vi "RS_SMBV100A.vi"(4 "error in":T15, 7 "Command":T16) -> (0 "error out":T15, 3 "Response":T13)   [LabVIEW 2018]
uses:
  MOKO_LabViewLibrary/MokoLowLevel/MokoLowLovelControl/MLLC_Command.ctl
  MOKO_LabViewLibrary/MokoLowLevel/MokoLowLovelControl/MLLC_Error.ctl
  MOKO_LabViewLibrary/MokoLowLevel/MokoLowLovelControl/MLLC_Mode.ctl
  MOKO_LabViewLibrary/MokoLowLevel/MokoLowLovelControl/MLLC_Response.ctl
  data/RS_SMBV100A_DynamWaypoints.ctl
  data/RS_SMBV100A_DynamWaypoint.ctl
  MOKO_LabViewLibrary/MokoLowLevel/MokoLowLovelControl/MLLC_ConnectCluster.ctl
  MOKO_LabViewLibrary/MokoLowLevel/MokoLowLovelControl/MLLC_InterfaceType.ctl
  MOKO_LabViewLibrary/MokoLowLevel/MokoLowLovelControl/MLLC_OpenedSession.ctl
  MOKO_LabViewLibrary/MokoLowLevel/MokoLowLovelControl/MLLC_InterfaceSettings.ctl
  MOKO_LabViewLibrary/MokoLowLevel/MokoLowLovelControl/MLLC_InterfaceKind.ctl
  MOKO_LabViewLibrary/MokoLowLevel/MokoLowLovelControl/MLLC_DriverName.ctl
  MOKO_LabViewLibrary/MokoLowLevel/MokoLowLovelControl/MLLC_ErrorCode.ctl
  MOKO_LabViewLibrary/MokoLowLevel/MokoLowLovelControl/MLLC_ResponseInit.ctl
  MOKO_LabViewLibrary/MokoLowLevel/MokoLowLovelControl/MLLC_Request.ctl
panel:
  in  "Request":T1="*IDN?"
  in  "ResponseInit":T2="Rohde&Schwarz,SMBV100A"
  in  "Error Code":T3=5450
  in  "Driver Name":T4="RS_SMBV100A"
  in  "Settings":T12={"GPS SCENARIO"="****************************** MOVEMENT FILE ******************************\nRESOLUTION: 50\nREFERENCE: 11.583333,48.150,500\nSTART: 0, 0, 0, 10\nSTAY: 10000\nLINE: 200, 0, 0\nLINE: 100, 0, 19.6\nLINE: 600, 0, 0\nLINE: 100, 0, -19.6\nARC: 1000, 500, 180\nLINE: -200, 0, 0\nLINE: -100, 0, 19.6\nLINE: -600, 0, 0\nLINE: -100, 0, -19.6\nARC: 0, 500, 180", "GLONASS SCENARIO"="****************************** MOVEMENT FILE ******************************\nRESOLUTION: 50\nREFERENCE: 11.583333,48.150,500\nSTART: 0, 0, 0, 10\nSTAY: 10000\nLINE: 200, 0, 0\nLINE: 100, 0, 19.6\nLINE: 600, 0, 0\nLINE: 100, 0, -19.6\nARC: 1000, 500, 180\nLINE: -200, 0, 0\nLINE: -100, 0, 19.6\nLINE: -600, 0, 0\nLINE: -100, 0, -19.6\nARC: 0, 500, 180", "GPS WAYPOINTS"=[], "GLONASS WAYPOINTS"=[], "GALILOE SCENARIO"="****************************** MOVEMENT FILE ******************************\nRESOLUTION: 50\nREFERENCE: 11.583333,48.150,500\nSTART: 0, 0, 0, 10\nSTAY: 10000\nLINE: 200, 0, 0\nLINE: 100, 0, 19.6\nLINE: 600, 0, 0\nLINE: 100, 0, -19.6\nARC: 1000, 500, 180\nLINE: -200, 0, 0\nLINE: -100, 0, 19.6\nLINE: -600, 0, 0\nLINE: -100, 0, -19.6\nARC: 0, 500, 180", "GALILEO WAYPOINTS"=[], "GPS WAYPOINTS STRING"="", "BASEBAND"="GPS", "BEIDOU SCENARIO"="****************************** MOVEMENT FILE ******************************\nRESOLUTION: 50\nREFERENCE: 11.583333,48.150,500\nSTART: 0, 0, 0, 10\nSTAY: 10000\nLINE: 200, 0, 0\nLINE: 100, 0, 19.6\nLINE: 600, 0, 0\nLINE: 100, 0, -19.6\nARC: 1000, 500, 180\nLINE: -200, 0, 0\nLINE: -100, 0, 19.6\nLINE: -600, 0, 0\nLINE: -100, 0, -19.6\nARC: 0, 500, 180", "QZSS SCENARIO"="****************************** MOVEMENT FILE ******************************\nRESOLUTION: 50\nREFERENCE: 11.583333,48.150,500\nSTART: 0, 0, 0, 10\nSTAY: 10000\nLINE: 200, 0, 0\nLINE: 100, 0, 19.6\nLINE: 600, 0, 0\nLINE: 100, 0, -19.6\nARC: 1000, 500, 180\nLINE: -200, 0, 0\nLINE: -100, 0, 19.6\nLINE: -600, 0, 0\nLINE: -100, 0, -19.6\nARC: 0, 500, 180", "BEIDOU WAYPOINTS"=[], "SSDK WAYPOINTS"=[], "Saved Data"=variant, "Data"={"Connect"={"InterfaceType"=enum."VISA", "OpenedSession"="TCPIP0::169.254.1.111::INSTR", "InterfaceSettings"={"Interface"=enum."Ethernet", "EOS 4 read"=enum."LF (\\n)", "EOS 4 write"=enum."LF (\\n)", "TMO, ms"=1000, "Sett"=variant}}}} {"SSDK WAYPOINTS"."Time" format="%<%.3X>T"; "SSDK WAYPOINTS"."Speed" format="%#.10g"; "SSDK WAYPOINTS"."Heigth" format="%#.10g"; "SSDK WAYPOINTS"."Longitude" format="%#.10g"; "SSDK WAYPOINTS"."Latitude" format="%#.10g"; "BEIDOU WAYPOINTS"."Time" format="%<%.3X>T"; "BEIDOU WAYPOINTS"."Speed" format="%#.10g"; "BEIDOU WAYPOINTS"."Heigth" format="%#.10g"; "BEIDOU WAYPOINTS"."Longitude" format="%#.10g"; "BEIDOU WAYPOINTS"."Latitude" format="%#.10g"; "GALILEO WAYPOINTS"."Time" format="%<%.3X>T"; "GALILEO WAYPOINTS"."Speed" format="%#.10g"; "GALILEO WAYPOINTS"."Heigth" format="%#.10g"; "GALILEO WAYPOINTS"."Longitude" format="%#.10g"; "GALILEO WAYPOINTS"."Latitude" format="%#.10g"; "GLONASS WAYPOINTS"."Time" format="%<%.3X>T"; "GLONASS WAYPOINTS"."Speed" format="%#.10g"; "GLONASS WAYPOINTS"."Heigth" format="%#.10g"; "GLONASS WAYPOINTS"."Longitude" format="%#.10g"; "GLONASS WAYPOINTS"."Latitude" format="%#.10g"; "GPS WAYPOINTS"."Time" format="%<%.3X>T"; "GPS WAYPOINTS"."Speed" format="%#.10g"; "GPS WAYPOINTS"."Heigth" format="%#.10g"; "GPS WAYPOINTS"."Longitude" format="%#.10g"; "GPS WAYPOINTS"."Latitude" format="%#.10g"}
  in  "Mode":T14=enum."Check"
  # "RS_SMBV100A"
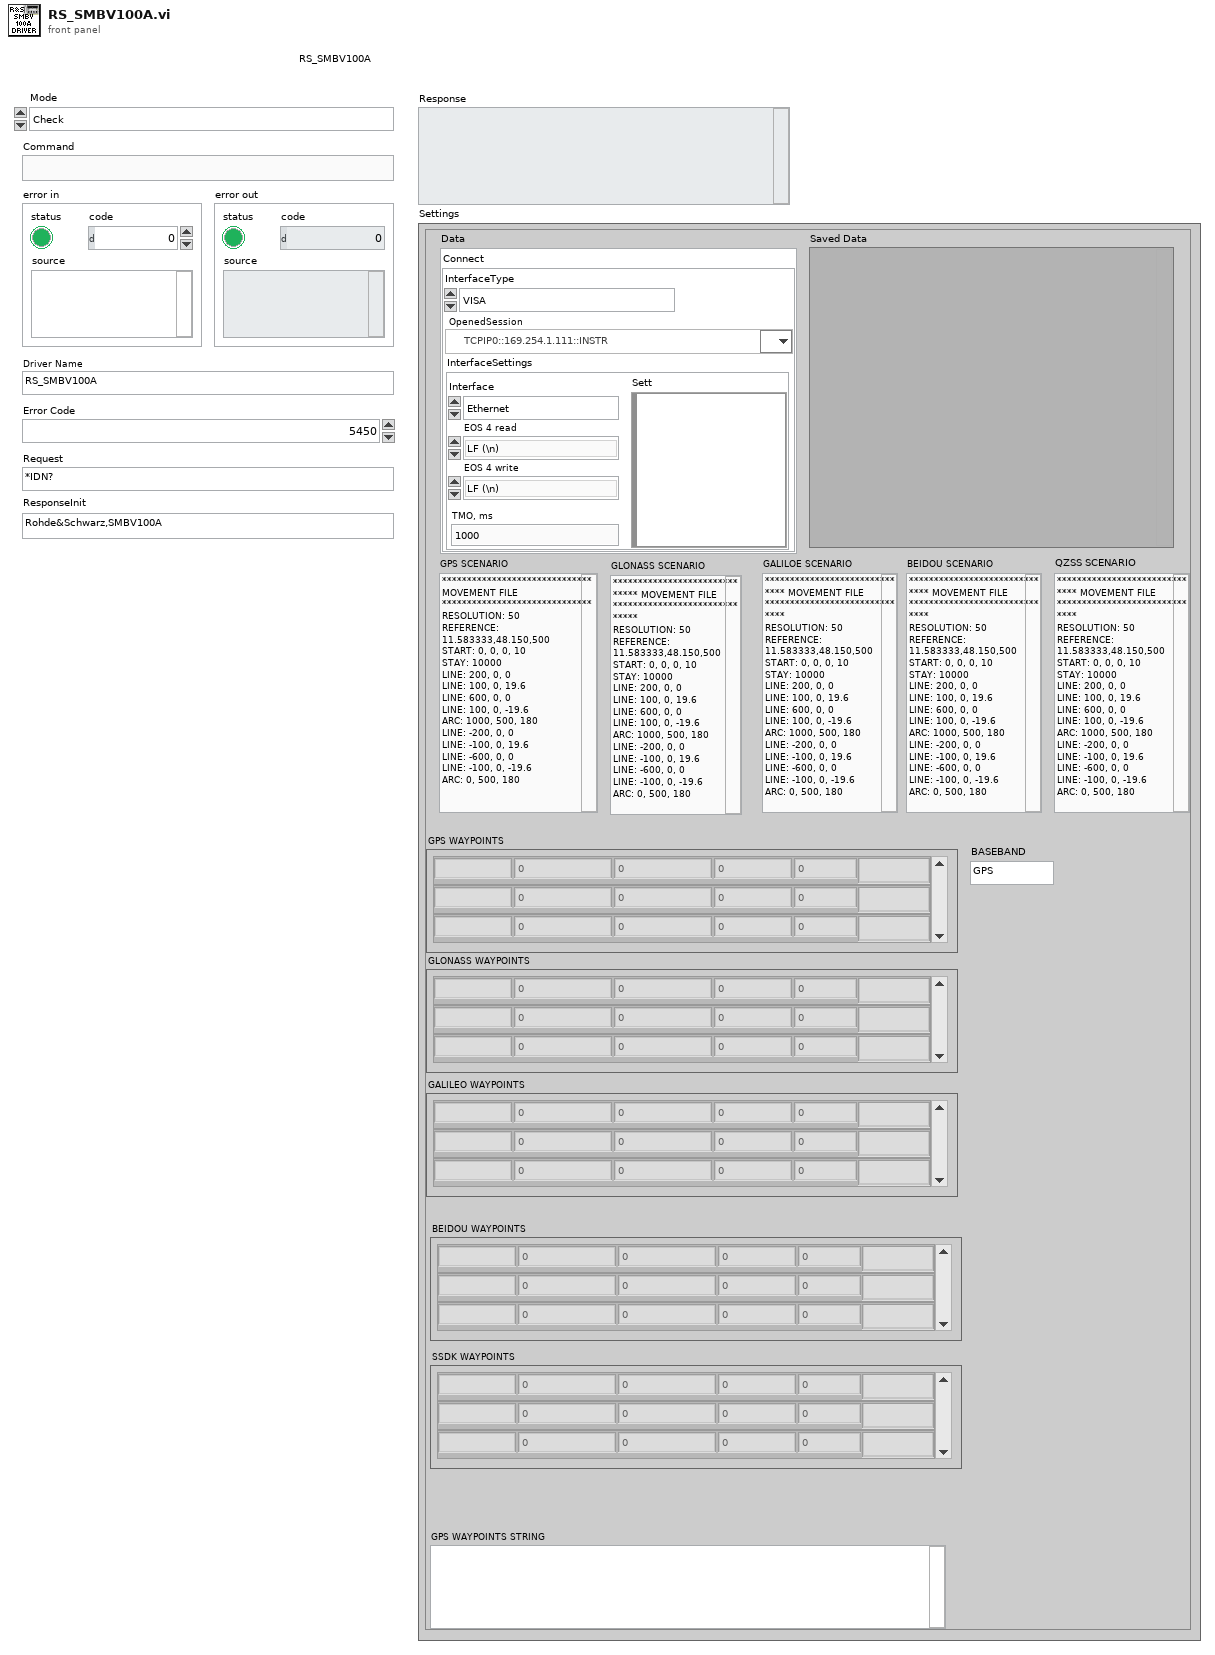
[diagram p1: front panel]
types:
  T1 = typedef "MLLC_Request.ctl" = string
  T2 = typedef "MLLC_ResponseInit.ctl" = string
  T3 = typedef "MLLC_ErrorCode.ctl" = u32
  T4 = typedef "MLLC_DriverName.ctl" = string
  T5 = typedef "RS_SMBV100A_DynamWaypoints.ctl" = T6[]
  T6 = typedef "RS_SMBV100A_DynamWaypoint.ctl" = cluster{"Time":timestamp, "Latitude":ext, "Longitude":ext, "Heigth":dbl, "Speed":dbl, "Scenario":string}
  T7 = typedef "MLLC_ConnectCluster.ctl" = cluster{"InterfaceType":T8, "OpenedSession":T9, "InterfaceSettings":T10}
  T8 = typedef "MLLC_InterfaceType.ctl" = enum16{"VISA", "Prologix USB-GPIB"}
  T9 = typedef "MLLC_OpenedSession.ctl" = refnum<visa-resource-name>
  T10 = typedef "MLLC_InterfaceSettings.ctl" = cluster{"Interface":T11, "EOS 4 read":enum16{"Default (=EOS 4 write)", "CR (\\r)", "LF (\\n)", "None"}, "EOS 4 write":enum16{"CR+LF (\\r\\n)", "CR (\\r)", "LF (\\n)", "None"}, "TMO, ms":i32, "Sett":variant}
  T11 = typedef "MLLC_InterfaceKind.ctl" = enum16{"RS232", "GPIB", "USB", "Ethernet", "another"}
  T12 = cluster{"GPS SCENARIO":string, "GLONASS SCENARIO":string, "GPS WAYPOINTS":T5, "GLONASS WAYPOINTS":T5, "GALILOE SCENARIO":string, "GALILEO WAYPOINTS":T5, "GPS WAYPOINTS STRING":string, "BASEBAND":string, "BEIDOU SCENARIO":string, "QZSS SCENARIO":string, "BEIDOU WAYPOINTS":T5, "SSDK WAYPOINTS":T5, "Saved Data":variant, "Data":cluster{"Connect":T7}}
  T13 = typedef "MLLC_Response.ctl" = string
  T14 = typedef "MLLC_Mode.ctl" = enum16{"get", "set", "close", "Init", "Check"}
  T15 = typedef "MLLC_Error.ctl" = errorcluster
  T16 = typedef "MLLC_Command.ctl" = string
  T17 = enum16{"open", "replace", "create", "open or create", "replace or create", "replace or create with confirmation"}
  T18 = typedef "RS_SMBV100A_Parsing Satelite.ctl" = cluster{"Time":dbl[], "Sat":dbl[], "State":dbl[], "NUMBERINSKY":dbl[], "STANDART":string[]}
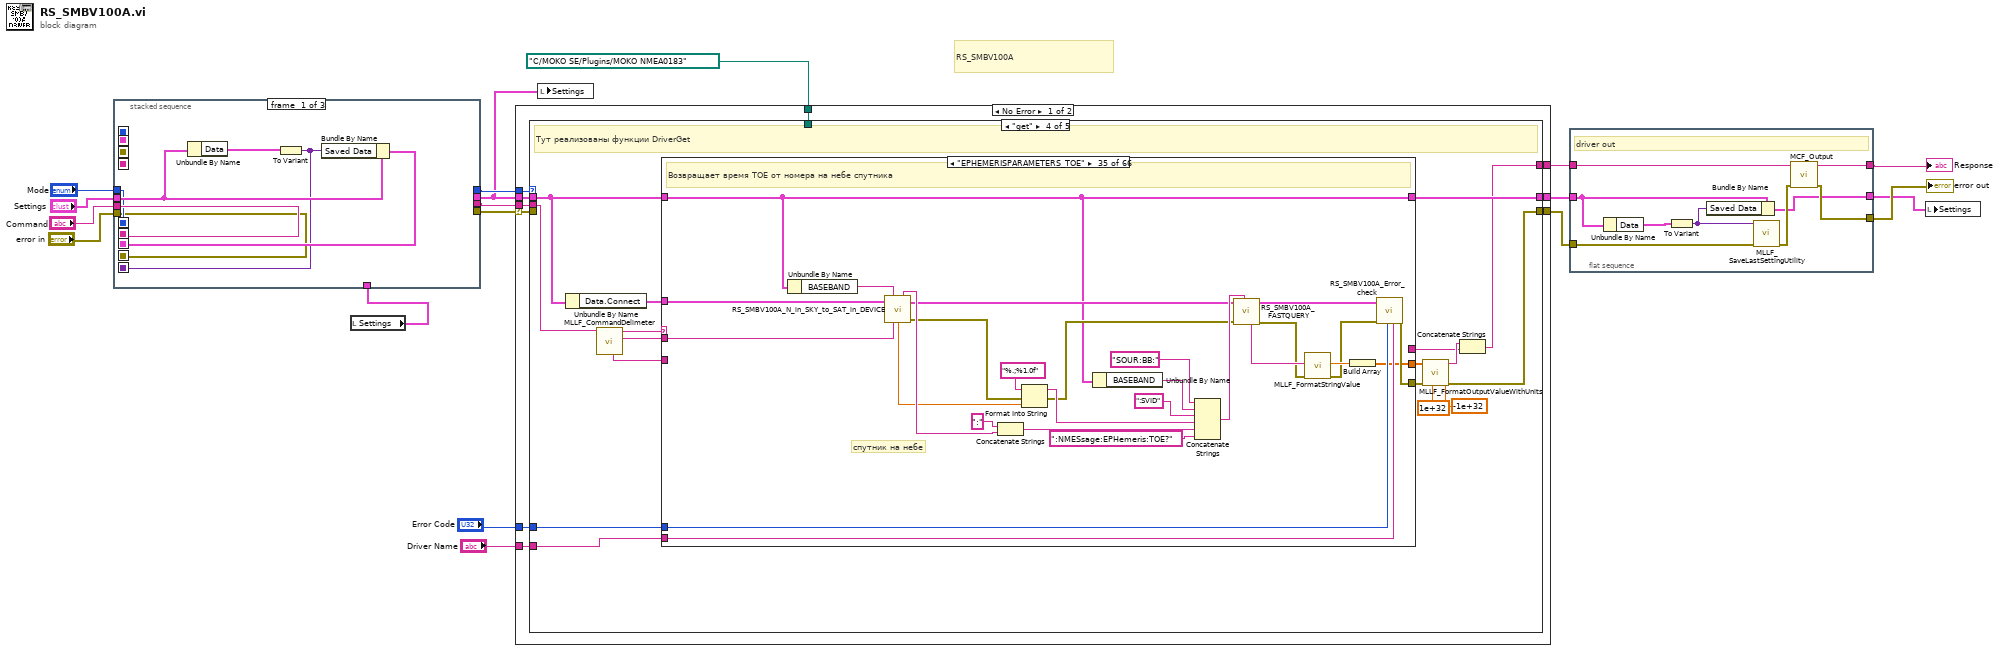
[diagram p0: block diagram]
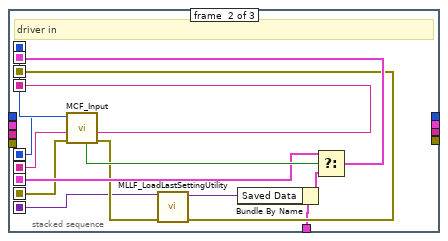
[diagram p2: hidden frame]
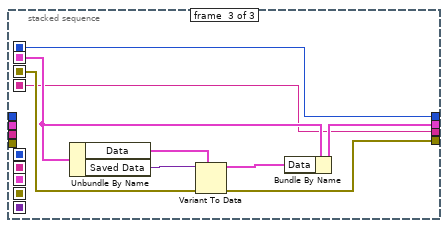
[diagram p3: hidden frame]
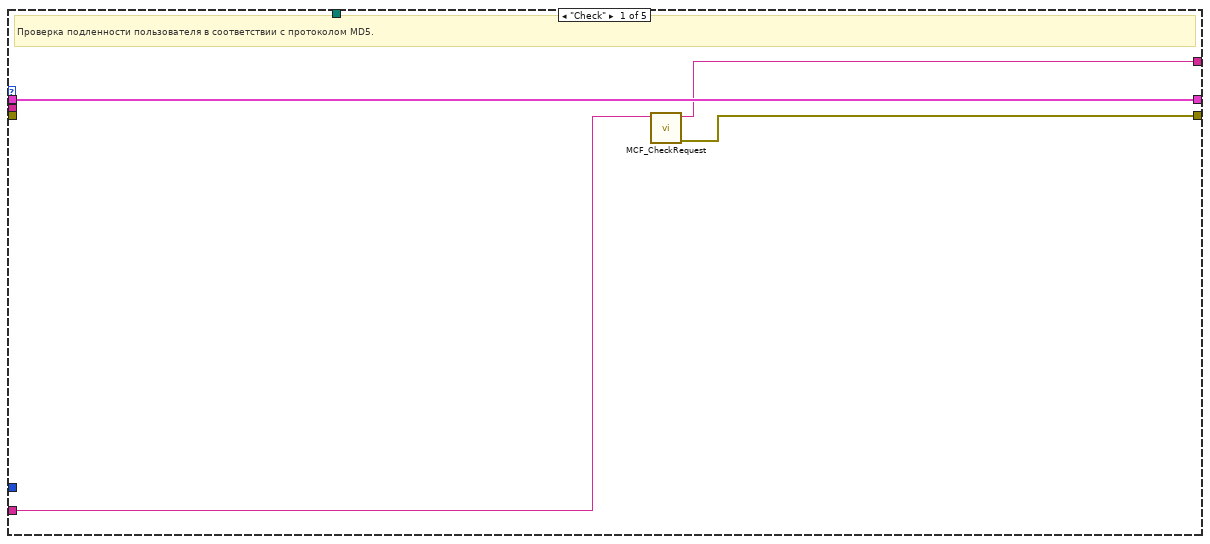
[diagram p4: hidden frame]
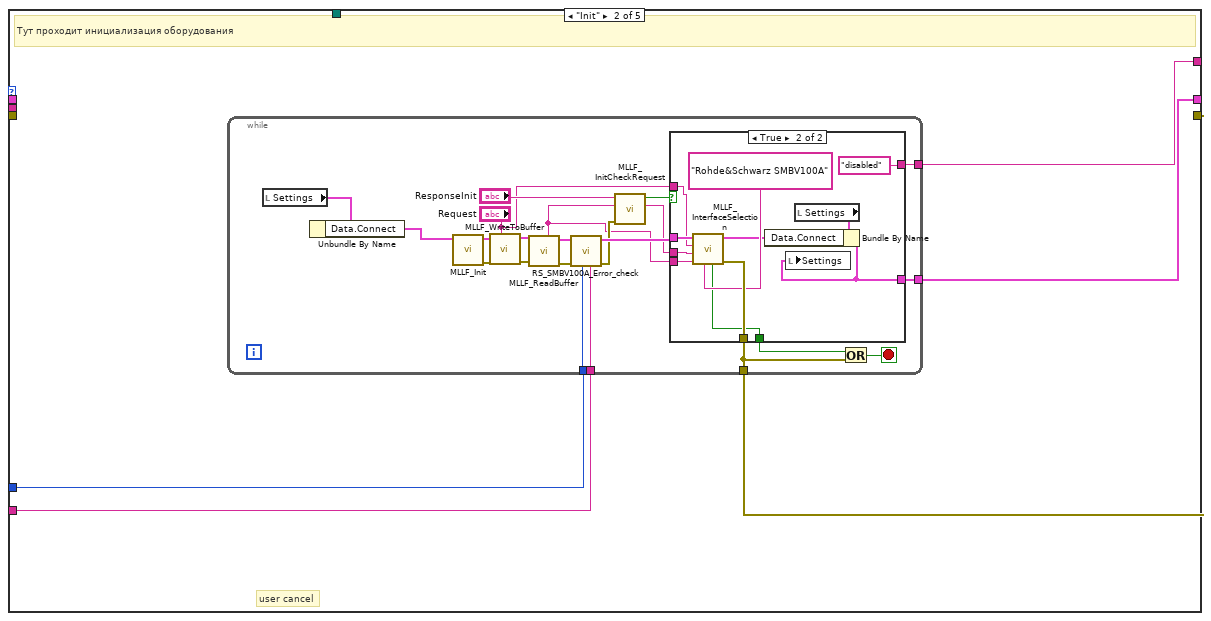
[diagram p5: hidden frame]
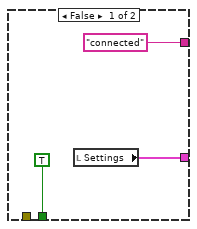
[diagram p6: hidden frame]
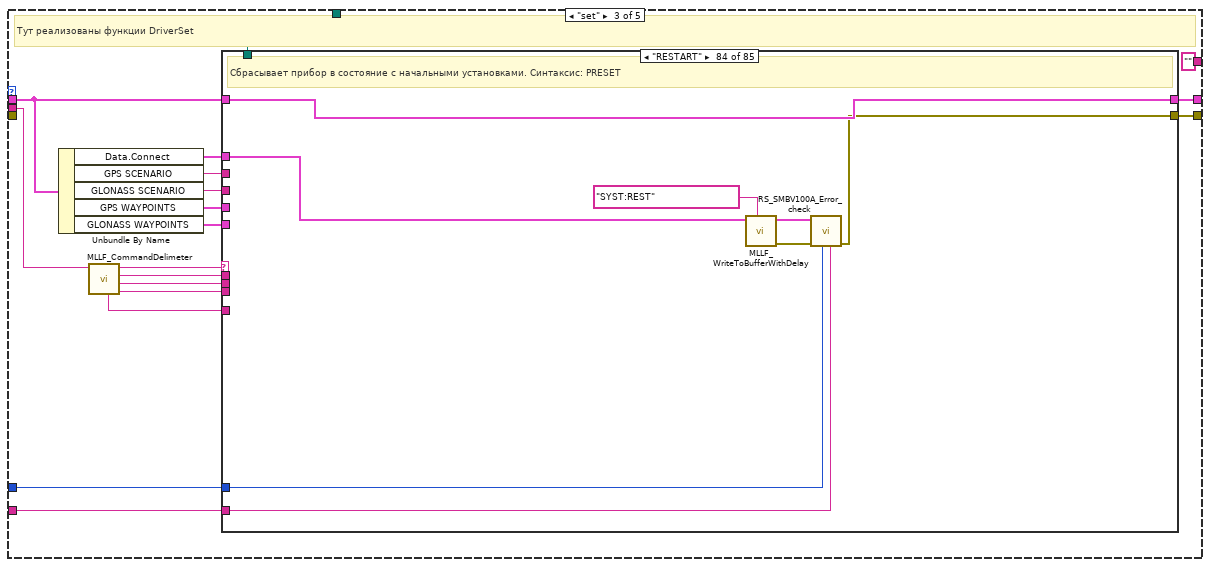
[diagram p7: hidden frame]
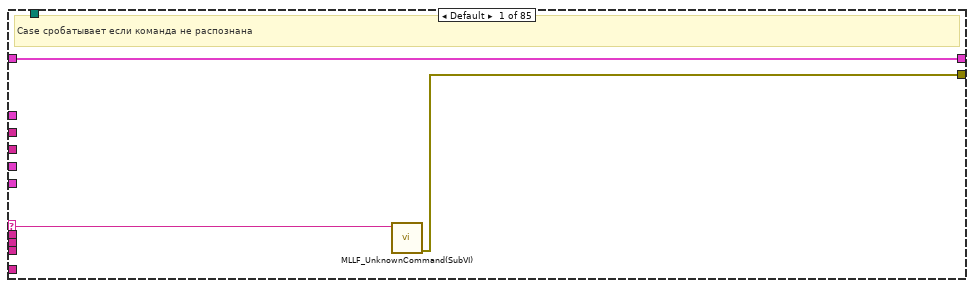
[diagram p8: hidden frame]
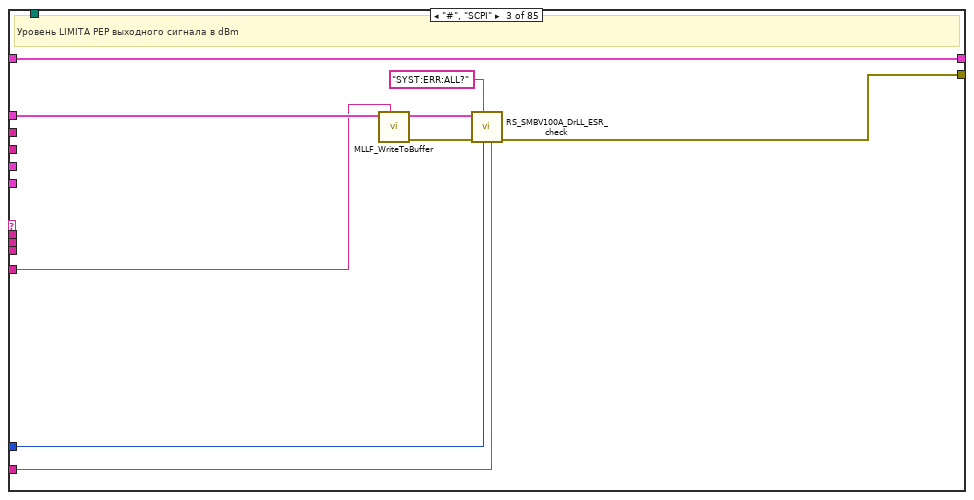
[diagram p10: hidden frame]
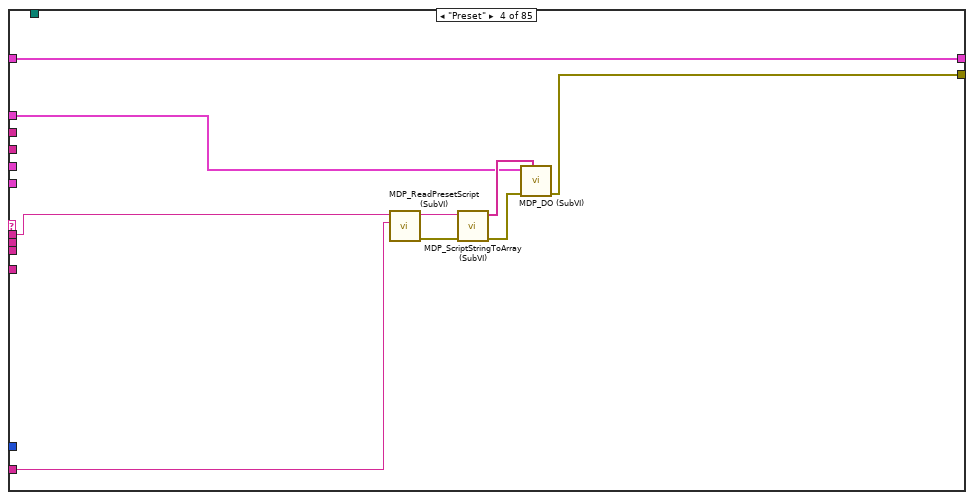
[diagram p11: hidden frame]
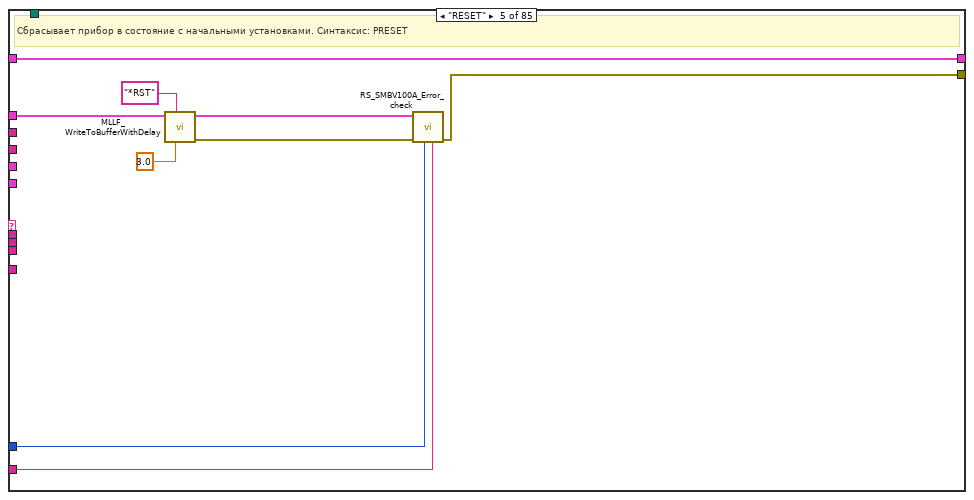
[diagram p12: hidden frame]
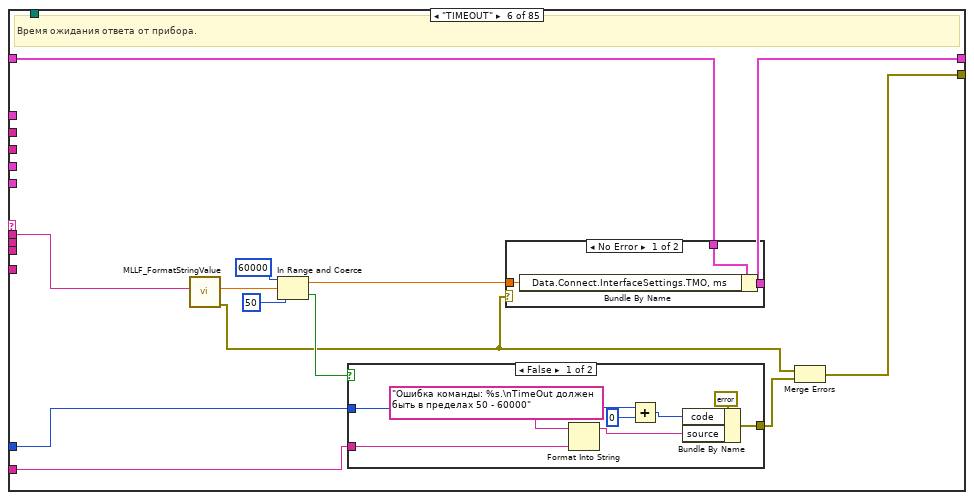
[diagram p13: hidden frame]
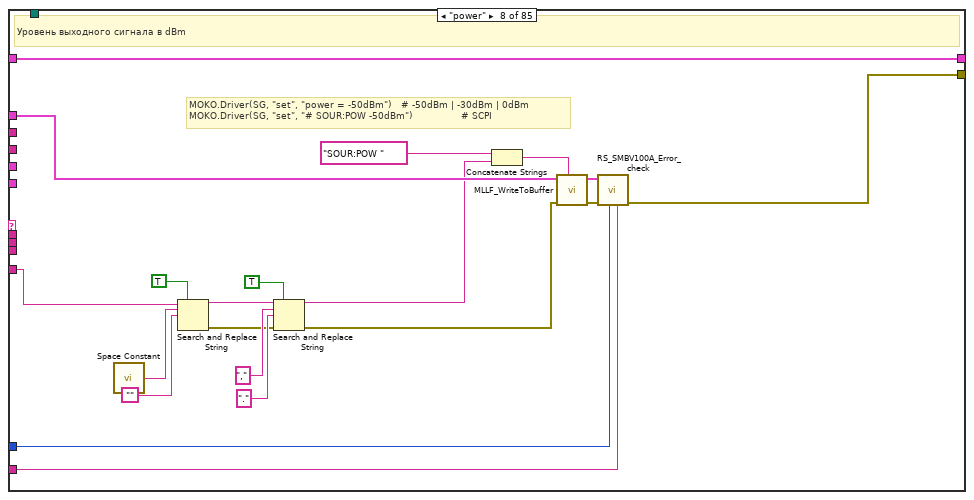
[diagram p17: hidden frame]
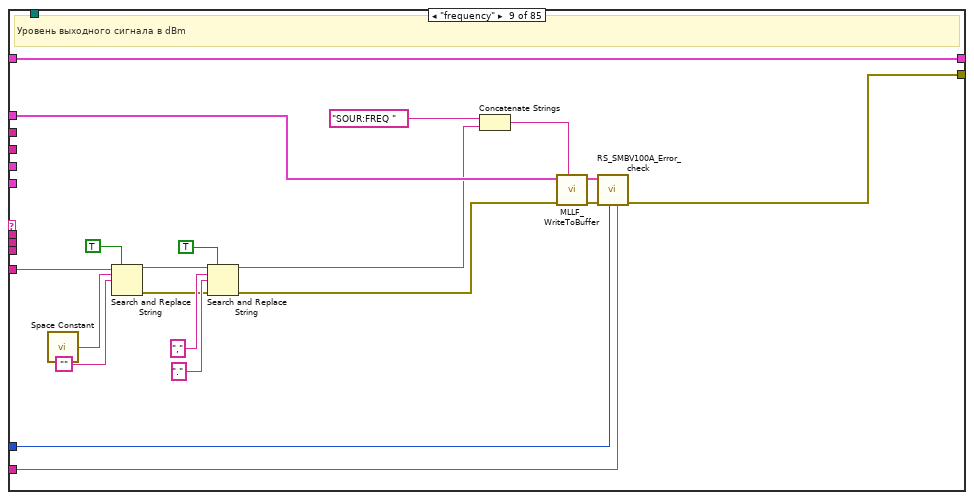
[diagram p18: hidden frame]
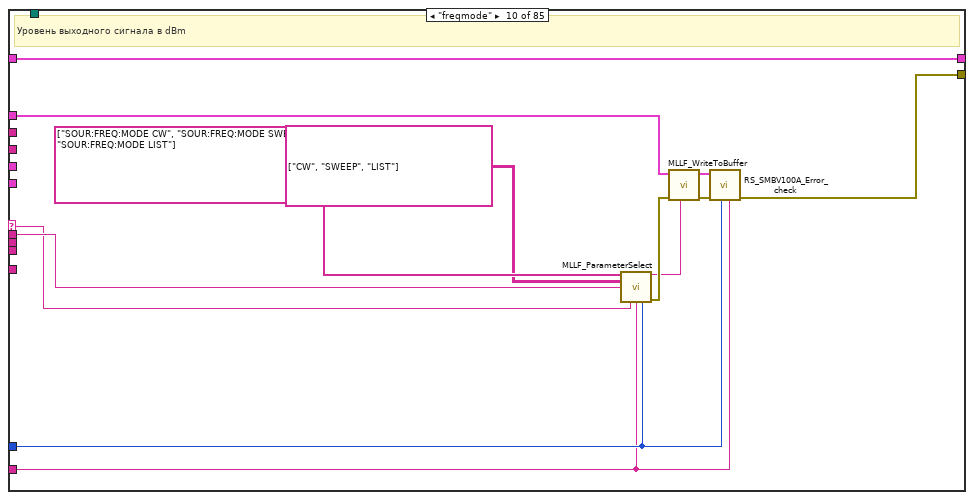
[diagram p19: hidden frame]
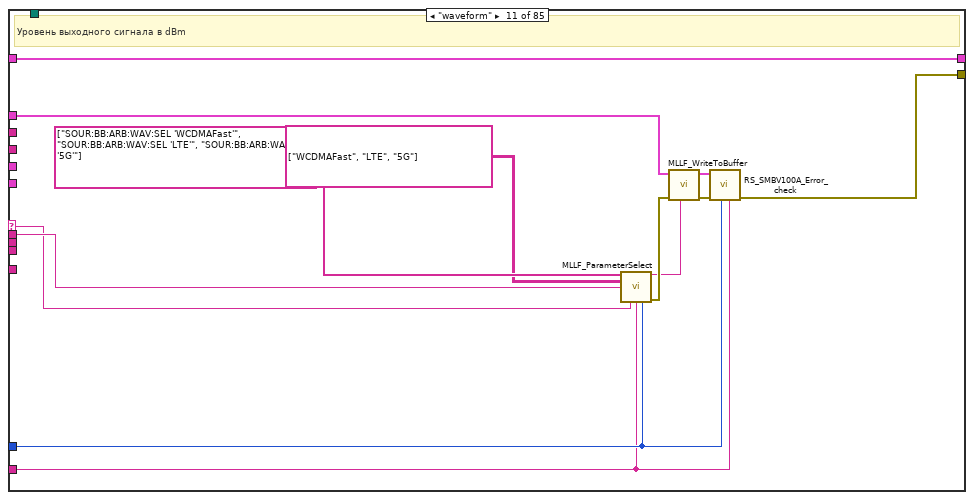
[diagram p20: hidden frame]
diagram:
  # "RS_SMBV100A"
  n1 = local read "Settings"() -> (w7:T12)
  n2 = stacked-sequence {
    seq-local: [w21 _ _] -> [_ w37 _]
    seq-local: [w20 _ _] -> [_ w38 _]
    seq-local: [w23 _ _] -> [_ w33 _]
    seq-local: [w19 _ _] -> [_ w32 _]
    seq-local: [w22 _ _] -> [_ w28 _]
    seq-local: [_ w29 _] -> [_ _ w45]
    seq-local: [_ w39 _] -> [_ _ w42]
    seq-local: [_ w36 _] -> [_ _ w41]
    seq-local: [_ w35 _] -> [_ _ w46]
    tunnel: "Command" -> [w21 _ _]
    tunnel: "Mode" -> [w20 _ _]
    tunnel: "error in" -> [w19 _ _]
    tunnel: "Settings" -> [w24 _ _]
    tunnel: w7 -> [_ w27 _]
    tunnel: [_ _ w41] -> w9
    tunnel: [_ _ w44] -> w10
    tunnel: [_ _ w43] -> w8
    tunnel: [_ _ w42] -> w11
    frame #0 {
      n3 = Unbundle By Name(w24) -> ("Data"=w25:cluster{"Connect":T7})
      n4 = To Variant(anything=w25) -> (Variant=w22:variant)
      n5 = Bundle By Name(cluster=w24, "Saved Data"=w22) -> (w23:T12)
    }
    frame #1 {
      # "driver in"
      n6 = call "MCF_Input.vi"("Error In"=w32, "Command in"=w37, "Mode in"=w38) -> ("Error Out"=w31:errorcluster, "Command out"=w36:string, "Mode out"=w39:T14, "Boolean"=w34:bool)  [unwired: 5 in]
      n7 = call "MLLF_LoadLastSettingUtility.vi"("Error In"=w31, "Save data in"=w28) -> ("Error Out"=w29:errorcluster, "Save data out"=w26:variant)  [unwired: 8 in]
      n8 = Bundle By Name(cluster=w27, "Saved Data"=w26) -> (w30:T12)
      n9 = Select(t=w33, s=w34, f=w30) -> (s? t:f=w35:T12)
    }
    frame #2 {
      n10 = Unbundle By Name(w46) -> ("Data"=w47:cluster{"Connect":T7}, "Saved Data"=w40:variant)
      n11 = Variant To Data(error in=w45, type=w47, Variant=w40) -> (data=w48:cluster{"Connect":T7}, error out=w43:errorcluster)
      n12 = Bundle By Name(cluster=w46, "Data"=w48) -> (w44:T12)
    }
  }
  n13 = case shown="No Error" w8 {
    selector: w8 -> [w55 w2154]
    tunnel: [w57 w2154] -> w4
    tunnel: w11 -> [w49 _]
    tunnel: [w58 _] -> w6
    tunnel: w9 -> [w56 _]
    tunnel: w10 -> [w52 w2153]
    tunnel: "Error Code" -> [w54 _]
    tunnel: "Driver Name" -> [w53 _]
    tunnel: [w51 w2153] -> w5
    tunnel: path "C:/MOKO SE/Plugins/MOKO NMEA0183" ("base path") -> [w50 _]
    frame No Error {
      n14 = case shown="\"get\"" w49 {
        tunnel: [w60 w63 "" ("Output String") w1264 "" ("Output String")] -> w58
        tunnel: [w59 w64 w121 w1263 w2151] -> w57
        tunnel: w56 -> [_ _ w104 w1276 _]
        tunnel: w55 -> [_ _ _ _ _]
        tunnel: w54 -> [_ w67 w120 w1273 _]
        tunnel: w53 -> [w61 w66 w117 w1272 _]
        tunnel: w52 -> [w62 _ w119 w1275 w2150]
        tunnel: [w62 w65 w118 w1274 w2150] -> w51
        tunnel: w50 -> [_ _ w116 _ _]
        frame "Check" {
          # "Проверка подленности пользователя в соответствии с протоколом MD5."
          n15 = call "MCF_CheckRequest.vi"("Driver Name"=w61) -> ("Error Out"=w59:errorcluster, "Output String"=w60:string)  [unwired: 9 in]
        }
        frame "Init" {
          # "user cancel"
          # "Тут проходит инициализация оборудования"
          n16 = while {
            tunnel: [w82] -> w64
            tunnel: w67 -> [w79]
            tunnel: w66 -> [w78]
            tunnel: [w75] -> w65
            tunnel: [w74] -> w63
            stop <- w81 stop-if-true
            n17 = local read "Settings"() -> (w84:T12)
            n18 = Unbundle By Name(w84) -> ("Data.Connect"=w85:T7)
            n19 = call "MLLF_Init.vi"("DriverConnect in"=w85) -> ("Error Out"=w87:errorcluster, "DriverConnect out"=w86:T7)  [unwired: 7 in]
            n20 = call "MLLF_WriteToBuffer.vi"("String"="Request", "error in"=w87, "DriverConnect in"=w86) -> ("error out"=w89:T15, "DriverConnect out"=w88:T7)  [unwired: 5 in]
            n21 = call "MLLF_ReadBuffer.vi"("Error In"=w89, "DriverConnect in"=w88) -> ("Error Out"=w76:errorcluster, "DriverConnect out"=w77:T7, "String"=w70:string)  [unwired: 6 in]
            n22 = call "RS_SMBV100A_Error_check.vi"("Driver Name"=w78, "Error Code"=w79, "Error In"=w76, "DriverConnect in"=w77) -> ("Error Out"=w72:errorcluster, "DriverConnect out"=w80:T7)  [unwired: 6 in]
            n23 = call "MLLF_InitCheckRequest.vi"("error in (no error)"=w72, "Answer"=w70, "Response Init"="ResponseInit") -> ("ResponseInit out"=w69:string, "Design"=w71:bool)  [unwired: 5 in, 2 out]
            n24 = case shown="True" w71 {
              tunnel: w80 -> [_ w102]
              tunnel: [TRUE w96] -> w83
              tunnel: [_ w103] -> w82
              tunnel: [w91 w98] -> w75
              tunnel: ["connected" "disabled"] -> w74
              tunnel: w70 -> [_ w95]
              tunnel: w69 -> [_ w94]
              tunnel: "Request" -> [_ w93]
              frame False {
                n25 = local read "Settings"() -> (w91:T12)
              }
              frame True {
                n26 = call "MLLF_InterfaceSelection.vi"("Driver Name"="Rohde&Schwarz SMBV100A" ("String"), "Answer:"=w95, "Response"=w94, "Request"=w93, "DriverConnect in"=w102) -> ("error out"=w103:T15, "DriverConnect out"=w100:T7, "stop init?"=w96:bool)  [unwired: 2 in, 2 out]
                n27 = local read "Settings"() -> (w99:T12)
                n28 = Bundle By Name(cluster=w99, "Data.Connect"=w100) -> (w98:T12)
                n29 = local write "Settings"(w98) -> ()
              }
            }
            n30 = Or(x=w83, y=w82) -> (x .or. y?=w81:bool)
          }
        }
        frame "set" {
          # "Тут реализованы функции DriverSet"
          n31 = Unbundle By Name(w119) -> ("Data.Connect"=w114:T7, "GPS SCENARIO"=w113:string, "GLONASS SCENARIO"=w112:string, "GPS WAYPOINTS"=w111:T5, "GLONASS WAYPOINTS"=w110:T5)
          n32 = call "MLLF_CommandDelimeter.vi"("command with param"=w104) -> ("param 3"=w106:string, "param 2"=w107:string, "param 1"=w108:string, "command"=w109:string, "Spit delimetre"=w105:string)  [unwired: 6 in]
          n33 = case shown="\"RESTART\"" w109 {
            selector: w109 -> [w123 _ _ _ _ _ _ _ _ w224 w237 _ w258 w266 _ _ _ _ _ _ _ _ _ _ _ _ w396 _ _ _ _ _ _ _ w530 w547 w562 _ _ _ w622 _ w661 w678 w697 _ _ w750 _ _ _ w793 _ w830 _ w862 w878 _ _ w913 _ _ w982 _ w1000 w1017 w1034 w1051 _ _ w1087 _ _ _ _ w1150 _ _ _ _ _ _ _ _ _]
            tunnel: [w122 _ w126 w135 w144 w156 _ w192 w212 w221 w234 w246 w255 w268 _ _ _ _ w304 w322 _ w351 _ w358 w374 w393 w404 _ w427 w446 w465 w484 w503 w522 w544 w561 w578 w594 w612 _ w630 w655 w669 w686 w711 w726 w739 w758 _ w778 w787 w801 w825 w840 w856 w871 w887 w901 _ w927 w948 w979 w990 _ w1008 w1025 w1043 w1059 w1075 _ w1095 w1110 w1122 _ w1144 w1166 _ w1181 w1200 _ w1215 w1222 w1230 w1238 w1253] -> w121
            tunnel: w120 -> [_ _ w130 _ w146 w157 _ w197 w217 w223 w236 w248 w257 w273 _ _ _ _ w303 _ _ w355 _ _ _ _ w409 _ w432 w451 w470 w489 w508 w527 w528 w545 w563 w593 _ _ w635 w660 w674 w691 w695 w731 w744 w748 _ w774 w792 w806 w829 w845 w861 w876 w892 w906 _ w911 w950 w981 w995 _ w1013 w1030 w1047 w1064 w1080 _ w1085 w1109 w1124 _ w1149 w1153 _ w1180 _ _ w1220 w1224 w1232 w1240 w1258]
            tunnel: w119 -> [w124 w125 w134 w143 w152 w155 w178 w198 w218 w231 w244 w252 w265 w278 w279 w280 w284 w288 w313 w326 w331 w338 w356 w359 w363 w387 w403 w413 w416 w436 w455 w472 w491 w510 w534 w551 w568 w603 w616 w621 w629 w644 w663 w680 w699 w714 w735 w752 w765 w769 w782 w795 w814 w832 w848 w865 w879 w897 w910 w915 w930 w953 w984 w999 w1002 w1019 w1037 w1053 w1069 w1084 w1089 w1105 w1117 w1128 w1129 w1154 w1167 w1190 w1203 w1207 w1221 w1229 w1237 w1245 w1259]
            tunnel: [w124 w125 w134 w143 w152 w154 w178 w198 w218 w231 w244 w252 w265 w278 w279 w280 w283 w288 w312 w325 w331 w338 w356 w359 w363 w387 w403 w413 w416 w436 w455 w472 w491 w510 w534 w551 w568 w602 w615 w621 w629 w644 w663 w680 w699 w714 w735 w752 w765 w769 w782 w795 w814 w832 w848 w865 w879 w897 w910 w915 w930 w953 w984 w999 w1002 w1019 w1037 w1053 w1069 w1084 w1089 w1105 w1117 w1128 w1129 w1154 w1167 w1189 w1202 w1207 w1221 w1229 w1237 w1245 w1259] -> w118
            tunnel: w114 -> [_ _ w133 w138 w147 _ _ w195 w215 w226 w239 w249 w260 w271 _ _ _ _ w306 _ _ w350 _ _ w383 w395 w407 _ w430 w449 w468 w487 w506 w525 w538 w555 w572 w596 _ _ w633 w658 w672 w689 w705 w729 w742 w759 _ w781 w790 w804 w824 w843 w859 w874 w890 w904 _ w923 w947 w978 w993 _ w1011 w1028 w1046 w1062 w1078 _ w1096 w1111 w1125 _ w1147 w1162 _ w1183 _ _ w1218 w1225 w1233 w1241 w1256]
            tunnel: w117 -> [_ _ w129 w136 w145 w158 _ w196 w216 w222 w235 w247 w256 w272 _ _ _ _ w302 _ _ w354 _ _ _ _ w408 _ w431 w450 w469 w488 w507 w526 w529 w546 w564 w592 _ _ w634 w659 w673 w690 w696 w730 w743 w749 _ w775 w791 w805 w828 w844 w860 w875 w891 w905 _ w912 w949 w980 w994 _ w1012 w1029 w1035 w1063 w1079 _ w1086 w1108 w1123 _ w1148 w1152 _ w1179 _ _ w1219 w1223 w1231 w1239 w1257]
            tunnel: w108 -> [_ _ _ w137 _ w153 _ _ _ w225 w238 _ w259 w267 _ _ w281 _ w291 w316 _ w333 _ _ w361 w392 w397 _ w418 w438 w457 w475 w494 w513 w531 w548 w565 w581 w606 _ w623 w641 w662 w679 w698 w716 w732 w751 _ w766 _ w794 w811 w831 w847 _ _ w894 _ w914 w934 w958 w983 _ w1001 w1018 w1036 w1052 w1068 _ w1088 w1102 _ _ w1135 w1151 _ w1169 w1195 _ w1211 _ _ _ w1249]
            tunnel: w113 -> [_ _ _ _ _ _ _ _ _ _ _ _ _ _ _ _ _ _ _ _ _ _ _ _ w369 _ _ _ _ _ _ _ _ _ _ _ _ _ _ _ _ _ _ _ _ _ _ _ _ _ _ _ _ _ _ _ _ _ _ _ _ _ _ _ _ _ _ _ _ _ _ _ _ _ _ _ _ _ _ _ _ _ _ _ _]
            tunnel: w112 -> [_ _ _ _ _ _ _ _ _ _ _ _ _ _ _ _ _ _ _ _ _ _ _ _ _ w389 _ _ _ _ _ _ _ _ _ _ _ _ _ _ _ _ _ _ _ _ _ _ _ _ _ _ _ _ _ _ _ _ _ _ _ _ _ _ _ _ _ _ _ _ _ _ _ _ _ _ _ _ _ _ _ _ _ _ _]
            tunnel: w111 -> [_ _ _ _ _ _ _ _ _ _ _ _ _ _ _ _ _ _ _ _ _ _ _ _ _ _ _ _ _ _ _ _ _ _ _ _ _ _ _ _ _ _ _ _ _ _ _ _ _ _ _ _ _ _ _ _ _ _ _ _ _ _ _ _ _ _ _ _ _ _ _ _ _ _ _ _ _ _ _ _ _ _ _ _ _]
            tunnel: w110 -> [_ _ _ _ _ _ _ _ _ _ _ _ _ _ _ _ _ _ _ _ _ _ _ w357 _ _ _ _ _ _ _ _ _ _ _ _ _ _ _ _ _ _ _ _ _ _ _ _ _ _ _ _ _ _ _ _ _ _ _ _ _ _ _ _ _ _ _ _ _ _ _ _ _ _ _ _ _ _ _ _ _ _ _ _ _]
            tunnel: w116 -> [_ _ _ _ _ _ _ _ _ _ _ _ _ _ _ _ _ _ w289 w315 _ _ _ _ w364 _ _ _ _ _ _ _ _ _ _ _ _ w579 w605 _ _ _ _ _ _ _ _ _ _ _ _ _ _ _ _ _ _ _ _ _ _ _ _ _ _ _ _ _ _ _ _ _ _ _ _ _ _ w1168 w1192 _ _ _ _ _ _]
            tunnel: w107 -> [_ _ _ _ _ _ _ _ _ _ _ _ _ _ _ _ _ _ _ _ _ w332 _ _ w360 _ _ _ _ _ _ _ _ _ _ _ _ _ _ _ _ w640 _ _ _ _ _ _ _ _ _ _ w810 _ _ _ _ _ _ _ _ _ _ _ _ _ _ _ _ _ _ _ _ _ _ _ _ _ _ _ _ _ _ _ _]
            tunnel: w106 -> [_ _ _ _ _ _ _ _ _ _ _ _ _ _ _ _ _ _ _ _ _ _ _ _ _ _ _ _ _ _ _ _ _ _ _ _ _ _ _ _ _ w639 _ _ _ _ _ _ _ _ _ _ _ _ _ _ _ _ _ _ _ _ _ _ _ _ _ _ _ _ _ _ _ _ _ _ _ _ _ _ _ _ _ _ _]
            tunnel: w105 -> [_ _ w132 _ _ _ _ w184 w209 _ _ _ _ _ _ _ _ _ _ _ _ _ _ _ _ _ _ _ _ _ _ _ _ _ _ _ _ _ _ _ _ _ _ _ _ _ _ _ _ _ _ _ _ _ _ _ _ _ _ _ _ _ _ _ _ _ _ _ _ _ _ _ _ _ _ _ _ _ _ _ _ _ _ _ _]
            frame Default {
              # "Case сробатывает если команда не распознана"
              n34 = call "MLLF_UnknownCommand(SubVI).vi"("Unknown command"=w123) -> ("error out"=w122:errorcluster)  [unwired: 10 in]
            }
            frame "______________ Standart ________________" {
            }
            frame "#", "SCPI" {
              # "Уровень LIMITA PEP выходного сигнала в dBm"
              n35 = call "MLLF_WriteToBuffer.vi"("String"=w132, "DriverConnect in"=w133) -> ("error out"=w127:T15, "DriverConnect out"=w128:T7)  [unwired: 6 in]
              n36 = call "RS_SMBV100A_DrLL_ESR_check.vi"("Driver Name"=w129, "Error Code"=w130, "Error Query"="SYST:ERR:ALL?", "Error In"=w127, "DriverConnect in"=w128) -> ("Error Out"=w126:errorcluster)  [unwired: 5 in, 1 out]
            }
            frame "Preset" {
              n37 = call "MDP_ReadPresetScript (SubVI).vi"("Driver Name"=w136, "String in"=w137) -> ("Error Out"=w140:errorcluster, "String out"=w141:string)  [unwired: 8 in]
              n38 = call "MDP_ScriptStringToArray (SubVI).vi"("Error In"=w140, "String script"=w141) -> ("Error Out"=w142:errorcluster, "Array script"=w139:string[])  [unwired: 8 in]
              n39 = call "MDP_DO (SubVI).vi"("Array script"=w139, "Error in (no error)"=w142, "DriverConnect in"=w138) -> ("Error Out"=w135:errorcluster)  [unwired: 7 in, 1 out]
            }
            frame "RESET" {
              # "Сбрасывает прибор в состояние с начальными установками. Синтаксис: PRESET"
              n40 = call "MLLF_WriteToBufferWithDelay.vi"("Delay Time ( 0,05 s)"=3.0, "Command"="*RST" ("String"), "DriverConnect in"=w147) -> ("Error Out"=w150:errorcluster, "DriverConnect out"=w151:T7)  [unwired: 7 in]
              n41 = call "RS_SMBV100A_Error_check.vi"("Driver Name"=w145, "Error Code"=w146, "Error In"=w150, "DriverConnect in"=w151) -> ("Error Out"=w144:errorcluster)  [unwired: 6 in, 1 out]
            }
            frame "TIMEOUT" {
              # "Время ожидания ответа от прибора."
              n42 = call "MLLF_FormatStringValue.vi"("String Value"=w153) -> ("error out"=w160:T15, "number"=w159:dbl)  [unwired: 8 in, 1 out]
              n43 = In Range and Coerce(upper limit=60000, x=w159, lower limit=50) -> (coerced(x)=w163:dbl, In Range?=w161:bool)
              n44 = case shown="False" w161 {
                tunnel: [w172 _] -> w162
                tunnel: w157 -> [w171 _]
                tunnel: w158 -> [w170 _]
                frame False {
                  n45 = Format Into String(format string="Ошибка команды: %s.\nTimeOut должен быть в пределах 50 - 60000", w170) -> (resulting string=w174:string)  [unwired: 2 in, 1 out]
                  n46 = Add(x=w171, y=0) -> (x+y=w175:T3)
                  n47 = Bundle By Name(cluster=errorcluster {"status"=TRUE, "code"=0, "source"=""} ("error out"), "code"=w175, "source"=w174) -> (w172:errorcluster)
                }
                frame True {
                }
              }
              n48 = case shown="No Error" w160 {
                tunnel: [w168 w169] -> w154
                tunnel: w155 -> [w167 w169]
                tunnel: w163 -> [w166 _]
                frame No Error {
                  n49 = Bundle By Name(cluster=w167, "Data.Connect.InterfaceSettings.TMO, ms"=w166) -> (w168:T12)
                }
                frame Error {
                }
              }
              n50 = Merge Errors(w160, w162) -> (w156:errorcluster)
            }
            frame "________________ Settings ________________" {
            }
            frame "power" {
              # "MOKO.Driver(SG, \"set\", \"power = -50dBm\")   # -50dBm | -30dBm | 0dBm\nMOKO.Driver(SG, \"set\", \"# SOUR:POW -50dBm\")                # SCPI"
              # "Уровень выходного сигнала в dBm"
              n51 = call <vilib>:"Space Constant.vi"() -> ("String"=w180:string)
              n52 = Search and Replace String(replace all?=TRUE ("replace all? (F)"), input string=w184, search string=w180, replace string="") -> (result string=w185:string, error out=w182:errorcluster)  [unwired: 4 in, 2 out]
              n53 = Search and Replace String(replace all?=TRUE ("replace all? (F)"), input string=w185, search string=",", replace string="." ("replace string (\"\")"), error in=w182) -> (result string=w183:string, error out=w181:errorcluster)  [unwired: 3 in, 2 out]
              n54 = Concatenate Strings("SOUR:POW " ("string"), w183) -> (w190:string)
              n55 = call "MLLF_WriteToBuffer.vi"("String"=w190, "error in"=w181, "DriverConnect in"=w195) -> ("error out"=w193:T15, "DriverConnect out"=w194:T7)  [unwired: 5 in]
              n56 = call "RS_SMBV100A_Error_check.vi"("Driver Name"=w196, "Error Code"=w197, "Error In"=w193, "DriverConnect in"=w194) -> ("Error Out"=w192:errorcluster)  [unwired: 6 in, 1 out]
            }
            frame "frequency" {
              # "Уровень выходного сигнала в dBm"
              n57 = call <vilib>:"Space Constant.vi"() -> ("String"=w201:string)
              n58 = Search and Replace String(replace all?=TRUE ("replace all? (F)"), input string=w209, search string=w201, replace string="") -> (result string=w204:string, error out=w199:errorcluster)  [unwired: 4 in, 2 out]
              n59 = Search and Replace String(replace all?=TRUE ("replace all? (F)"), input string=w204, search string=",", replace string="." ("replace string (\"\")"), error in=w199) -> (result string=w203:string, error out=w202:errorcluster)  [unwired: 3 in, 2 out]
              n60 = Concatenate Strings("SOUR:FREQ " ("string"), w203) -> (w210:string)
              n61 = call "MLLF_WriteToBuffer.vi"("String"=w210, "error in"=w202, "DriverConnect in"=w215) -> ("error out"=w213:T15, "DriverConnect out"=w214:T7)  [unwired: 5 in]
              n62 = call "RS_SMBV100A_Error_check.vi"("Driver Name"=w216, "Error Code"=w217, "Error In"=w213, "DriverConnect in"=w214) -> ("Error Out"=w212:errorcluster)  [unwired: 6 in, 1 out]
            }
            frame "freqmode" {
              # "Уровень выходного сигнала в dBm"
              n63 = call "MLLF_ParameterSelect.vi"("Command to equipment"=string[] ["SOUR:FREQ:MODE CW", "SOUR:FREQ:MODE SWEEP", "SOUR:FREQ:MODE LIST"], "Names"=string[][] [["CW"], ["SWEEP"], ["LIST"]], "Input"=w225, "Command"=w224, "Driver Name"=w222, "Error Code"=w223) -> ("Choice"=w219:string, "Error Out"=w229:errorcluster)  [unwired: 8 in]
              n64 = call "MLLF_WriteToBuffer.vi"("String"=w219, "error in"=w229, "DriverConnect in"=w226) -> ("error out"=w227:T15, "DriverConnect out"=w228:T7)  [unwired: 5 in]
              n65 = call "RS_SMBV100A_Error_check.vi"("Driver Name"=w222, "Error Code"=w223, "Error In"=w227, "DriverConnect in"=w228) -> ("Error Out"=w221:errorcluster)  [unwired: 6 in, 1 out]
            }
            frame "waveform" {
              # "Уровень выходного сигнала в dBm"
              n66 = call "MLLF_ParameterSelect.vi"("Command to equipment"=string[] ["SOUR:BB:ARB:WAV:SEL 'WCDMAFast'", "SOUR:BB:ARB:WAV:SEL 'LTE'", "SOUR:BB:ARB:WAV:SEL '5G'"], "Names"=string[][] [["WCDMAFast"], ["LTE"], ["5G"]], "Input"=w238, "Command"=w237, "Driver Name"=w235, "Error Code"=w236) -> ("Choice"=w232:string, "Error Out"=w242:errorcluster)  [unwired: 8 in]
              n67 = call "MLLF_WriteToBuffer.vi"("String"=w232, "error in"=w242, "DriverConnect in"=w239) -> ("error out"=w240:T15, "DriverConnect out"=w241:T7)  [unwired: 5 in]
              n68 = call "RS_SMBV100A_Error_check.vi"("Driver Name"=w235, "Error Code"=w236, "Error In"=w240, "DriverConnect in"=w241) -> ("Error Out"=w234:errorcluster)  [unwired: 6 in, 1 out]
            }
            frame "arb_reset" {
              # "Уровень выходного сигнала в dBm"
              n69 = call "MLLF_WriteToBuffer.vi"("String"="SOUR:BB:ARB:PRESet" ("Choice"), "DriverConnect in"=w249) -> ("error out"=w250:T15, "DriverConnect out"=w251:T7)  [unwired: 6 in]
              n70 = call "RS_SMBV100A_Error_check.vi"("Driver Name"=w247, "Error Code"=w248, "Error In"=w250, "DriverConnect in"=w251) -> ("Error Out"=w246:errorcluster)  [unwired: 6 in, 1 out]
            }
            frame "arb_state" {
              # "Уровень выходного сигнала в dBm"
              n71 = call "MLLF_ParameterSelect.vi"("Command to equipment"=string[] ["SOUR:BB:ARB:STAT ON", "SOUR:BB:ARB:STAT OFF"], "Names"=string[][] [["ON"], ["OFF"]], "Input"=w259, "Command"=w258, "Driver Name"=w256, "Error Code"=w257) -> ("Choice"=w253:string, "Error Out"=w263:errorcluster)  [unwired: 8 in]
              n72 = call "MLLF_WriteToBuffer.vi"("String"=w253, "error in"=w263, "DriverConnect in"=w260) -> ("error out"=w261:T15, "DriverConnect out"=w262:T7)  [unwired: 5 in]
              n73 = call "RS_SMBV100A_Error_check.vi"("Driver Name"=w256, "Error Code"=w257, "Error In"=w261, "DriverConnect in"=w262) -> ("Error Out"=w255:errorcluster)  [unwired: 6 in, 1 out]
            }
            frame "output" {
              # "ка = щт щаа"
              # "Включение\\Выключение блока RF\\A Mod"
              n74 = call "MLLF_ParameterSelect.vi"("Command to equipment"=string[] ["OUTP:STAT ON", "OUTP:STAT OFF"], "Names"=string[][] [["ON"], ["OFF"]], "Input"=w267, "Command"=w266, "Driver Name"=w272, "Error Code"=w273) -> ("Choice"=w274:string, "Error Out"=w275:errorcluster)  [unwired: 8 in]
              n75 = call "MLLF_WriteToBuffer.vi"("String"=w274, "error in"=w275, "DriverConnect in"=w271) -> ("error out"=w269:T15, "DriverConnect out"=w270:T7)  [unwired: 5 in]
              n76 = call "RS_SMBV100A_Error_check.vi"("Driver Name"=w272, "Error Code"=w273, "Error In"=w269, "DriverConnect in"=w270) -> ("Error Out"=w268:errorcluster)  [unwired: 6 in, 1 out]
            }
            frame "_______________________________________" {
            }
            frame "----- BASEBAND -----" {
              # "МОДУЛЬ BASEBAND"
            }
            frame "BASEBAND" {
              # "BASEBAND= GPS\nBASEBAND= GLON GLONASS\nBASEBAND  =   GALILEO GAL"
              # "МОДУЛЬ BASEBAND"
              n77 = case shown="\"GLON\", \"GLONASS\"" w281 {
                tunnel: ["GLON" ("regular expression") "GPS" "GAL" ("regular expression")] -> w282
                frame "GLON", "GLONASS" {
                }
                frame "GPS", Default {
                }
                frame "GAL", "GALILEO" {
                }
              }
              n78 = Bundle By Name(cluster=w284, "BASEBAND"=w282) -> (w283:T12)
            }
            frame "----GALILEO BASEBAND----" {
            }
            frame "GALILEO_LOAD_SCENARIO" {
              w310 = "'" ("string")
              # "?????????????????????????????????????????????????"
              # "Осуществляется подгрузка и в прибор и в драйвер сценария."
              # "загружаем сценарий для локации GAL"
              n79 = Search and Replace String(replace all?=TRUE, input string=w291, search string="\"", replace string="") -> (result string=w290:string)  [unwired: 4 in, 3 out]
              n80 = Concatenate Strings("GNSS\\scenario\\", w290, ".txt") -> (w300:string)
              n81 = Build Path(base path=w289, name or relative path=w300) -> (appended path=w295:path)
              n82 = Concatenate Strings("/hdd/unitess/GNSS/scenario/", w290, ".txt") -> (w296:string)
              n83 = Read from Text File(file (use dialog)=w295) -> (text=w314:string, error out=w305:errorcluster)  [unwired: 3 in, 2 out]
              n84 = Bundle By Name(cluster=w313, "GALILOE SCENARIO"=w314) -> (w312:T12)
              n85 = Concatenate Strings("SOUR:BB:GAL:LOC:WAYP:FILE " ("string"), w310, w296, w310) -> (w307:string)
              n86 = call "MLLF_WriteToBuffer.vi"("String"=w307, "error in"=w305, "DriverConnect in"=w306) -> ("error out"=w308:T15, "DriverConnect out"=w309:T7)  [unwired: 5 in]
              n87 = call "RS_SMBV100A_Error_check.vi"("Driver Name"=w302, "Error Code"=w303, "Error In"=w308, "DriverConnect in"=w309) -> ("Error Out"=w304:errorcluster)  [unwired: 6 in, 1 out]
            }
            frame "GALILEO_LOAD_WAYPOINTS" {
              # "Импортируем WAyPOINTS в драйвер"
              n88 = Search and Replace String(replace all?=TRUE, input string=w316, search string="\"", replace string="") -> (result string=w317:string)  [unwired: 4 in, 3 out]
              n89 = Concatenate Strings("GNSS\\waypoints\\", w317, ".txt") -> (w329:string)
              n90 = Build Path(base path=w315, name or relative path=w329) -> (appended path=w327:path)
              n91 = Read from Text File(file (use dialog)=w327) -> (text=w324:string, error out=w323:errorcluster)  [unwired: 3 in, 2 out]
              n92 = call "RS_SMBV100A_arrayStringToDOUBLE.vi"("string"=w324, "error in"=w323) -> ("Dynam waypoints"=w321:T5, "error out"=w322:errorcluster)  [unwired: 1 in]
              n93 = Bundle By Name(cluster=w326, "GALILEO WAYPOINTS"=w321) -> (w325:T12)
            }
            frame "---- GLONASS BASEBAND -----" {
              # "Функции настройки в локации GLONASS"
            }
            frame "EPHEMERIS_PARAMETERS_TOE", "EPHEMERISPARAMETERS_TOE" {
              # "спутник на небе"
              # "Функции настройки ephemeris в локации GPS - TOE"
              n94 = Unbundle By Name(w338) -> ("BASEBAND"=w335:string)
              n95 = To Upper Case(1:w333) -> (0:w334:string)
              n96 = call "RS_SMBV100A_N_in_SKY_to_SAT_in_DEVICE.vi"("DriverConnect in"=w350, "BASEBAND"=w335, "String Value"=w334) -> ("GNSS"=w342:string, "DriverConnect out"=w346:T7, "SATINSKY_for_DEVICE"=w339:dbl, "Error Out"=w345:errorcluster)  [unwired: 8 in, 1 out]
              n97 = Concatenate Strings(":" ("regular expression"), w342) -> (w341:string)
              n98 = Format Into String(format string="%.;%1.0f" ("format"), error in=w345, w339) -> (resulting string=w348:string, error out=w344:errorcluster)  [unwired: 1 in]
              n99 = Concatenate Strings("SOUR:BB:" ("regular expression"), w335, ":SVID" ("regular expression"), w348, w341, ":NMESsage:EPHemeris:TOE " ("regular expression"), w332) -> (w347:string)
              n100 = call "MLLF_WriteToBuffer.vi"("String"=w347, "error in"=w344, "DriverConnect in"=w346) -> ("error out"=w352:T15, "DriverConnect out"=w353:T7)  [unwired: 5 in]
              n101 = call "RS_SMBV100A_Error_check.vi"("Driver Name"=w354, "Error Code"=w355, "Error In"=w352, "DriverConnect in"=w353) -> ("Error Out"=w351:errorcluster)  [unwired: 6 in, 1 out]
            }
            frame "---------------------------- EXPORT ----------------------------------" {
            }
            frame "EXPORT_LOAD_EDWAYPOINTS_2_NMEA", "EXPORTLOADEDWAYPOINTS2NMEA" {
              # "ЭТОТ ФУНКЦИОНАЛ НЕ ИСПОЛЬЗУЕТСЯ"
              # "Импортируем загруженные файлы NMEA программу"
              n102 = call "RS_SMBV100A_ImportToNMEA.vi"("Dynam waypoints"=w357) -> ("error out"=w358:errorcluster)  [unwired: 10 in]
            }
            frame "EXPORTWAYPOINTS2FILE" {
              # "Записываем WAYPOINT по GLON в файл"
              n103 = Unbundle By Name(w363) -> ("BASEBAND"=w362:string)
              n104 = call "MLLF_FormatStringValue.vi"("String Value"=w361) -> ("error out"=w384:T15, "number"=w385:dbl)  [unwired: 8 in, 1 out]
              n105 = Search and Replace String(replace all?=TRUE, input string=w360, search string="\"", replace string="") -> (result string=w365:string)  [unwired: 4 in, 3 out]
              n106 = Concatenate Strings("GNSS\\waypoints\\", w365, ".txt") -> (w372:string)
              n107 = Build Path(base path=w364, name or relative path=w372) -> (appended path=w371:path)
              n108 = call "RS_SMBV100A_RequestWaypoints.vi"("DriverConnect in"=w383, "scenario time, c"=w385, "Error In"=w384, "BASEBAND"=w362, "Scenario in"=w369) -> ("Waypoints, txt"=w375:string, "Error Out"=w376:errorcluster)  [unwired: 7 in, 2 out]
              n109 = Open/Create/Replace File(file path (use dialog)=w371, error in=w376, operation (0:open)=T17."replace or create", access (0:read/write)=enum16{"read/write", "read-only", "write-only"}."read/write") -> (refnum out=w380:refnum<file>, error out=w377:errorcluster)  [unwired: 2 in, 1 out]
              n110 = Write to Text File(file (use dialog)=w380, text=w375, error in=w377) -> (refnum out=w378:refnum<file>, error out=w379:errorcluster)  [unwired: 1 in, 1 out]
              n111 = Close File(refnum=w378, error in=w379) -> (error out=w374:errorcluster)  [unwired: 1 out]
            }
            frame "EXPORTWAYPOINTS2NMEA" {
              # "Импортируем файлы NMEA программу"
              n112 = Unbundle By Name(w387) -> ("BASEBAND"=w386:string)
              n113 = call "MLLF_FormatStringValue.vi"("String Value"=w392) -> ("error out"=w390:T15, "number"=w391:dbl)  [unwired: 8 in, 1 out]
              n114 = call "RS_SMBV100A_RequestWaypoints.vi"("DriverConnect in"=w395, "scenario time, c"=w391, "Error In"=w390, "BASEBAND"=w386, "Scenario in"=w389) -> ("Dynam waypoints"=w388:T5, "Error Out"=w394:errorcluster)  [unwired: 7 in, 2 out]
              n115 = call "RS_SMBV100A_ImportToNMEA.vi"("error in"=w394, "Dynam waypoints"=w388) -> ("error out"=w393:errorcluster)  [unwired: 9 in]
            }
            frame "GLOBAL_EPHEMERIS_REAL_TIME_PROJECTION", "GLOBALEPHEMERISREAL_TIMEPROJECTION" {
              # "SOUR:BB:GLON:SAT:GRTP"
              # "GLON _ Global Ephemeris Real-Time Projection"
              n116 = Unbundle By Name(w403) -> ("BASEBAND"=w401:string)
              n117 = call "MLLF_ParameterSelect.vi"("Command to equipment"=string[] ["ON", "OFF"], "Names"=string[][] [["ON", "1", "ENABLE", "EN"], ["OFF", "0", "DISABLE", "DIS"]], "Input"=w397, "Command"=w396, "Driver Name"=w408, "Error Code"=w409) -> ("Choice"=w399:string, "Error Out"=w410:errorcluster)  [unwired: 8 in]
              n118 = Concatenate Strings("SOUR:BB:", w401, ":SAT:GRTP ", w399) -> (w398:string)
              n119 = call "MLLF_WriteToBuffer.vi"("String"=w398, "error in"=w410, "DriverConnect in"=w407) -> ("error out"=w405:T15, "DriverConnect out"=w406:T7)  [unwired: 5 in]
              n120 = call "RS_SMBV100A_Error_check.vi"("Driver Name"=w408, "Error Code"=w409, "Error In"=w405, "DriverConnect in"=w406) -> ("Error Out"=w404:errorcluster)  [unwired: 6 in, 1 out]
            }
            frame "---------------------- GNSS_CONFIGURATION ---------------------------------" {
            }
            frame "GNSS_CONFIGURATION_ALMANAC_FILE_GALILEO", "GNSSCONFIGURATION_ALMANACFILE_GALILEO" {
              w424 = "'" ("string")
              # "Выбор файла АЛЬМАНАХА GPS in GLON"
              n121 = Search and Replace String(replace all?=TRUE, input string=w418, search string="\"", replace string="") -> (result string=w417:string)  [unwired: 4 in, 3 out]
              n122 = Unbundle By Name(w416) -> ("BASEBAND"=w415:string)
              n123 = Concatenate Strings("/hdd/GNSS/almanac/" ("string"), w417) -> (w422:string)
              n124 = Concatenate Strings("SOURce1:BB:" ("string"), w415, ":NAVigation:ALManac:GAL:FILE " ("string"), w424, w422, w424) -> (w425:string)
              n125 = call "MLLF_WriteToBuffer.vi"("String"=w425, "DriverConnect in"=w430) -> ("error out"=w428:T15, "DriverConnect out"=w429:T7)  [unwired: 6 in]
              n126 = call "RS_SMBV100A_Error_check.vi"("Driver Name"=w431, "Error Code"=w432, "Error In"=w428, "DriverConnect in"=w429) -> ("Error Out"=w427:errorcluster)  [unwired: 6 in, 1 out]
            }
            frame "GNSS_CONFIGURATION_ALMANAC_FILE_GLONASS", "GNSSCONFIGURATION_ALMANACFILE_GLONASS" {
              w444 = "'" ("string")
              # "Выбор файла АЛЬМАНАХА Glonas in GLON"
              n127 = Search and Replace String(replace all?=TRUE, input string=w438, search string="\"", replace string="") -> (result string=w437:string)  [unwired: 4 in, 3 out]
              n128 = Unbundle By Name(w436) -> ("BASEBAND"=w435:string)
              n129 = Concatenate Strings("/hdd/GNSS/almanac/" ("string"), w437) -> (w442:string)
              n130 = Concatenate Strings("SOURce1:BB:" ("string"), w435, ":NAVigation:ALManac:GLON:FILE " ("string"), w444, w442, w444) -> (w445:string)
              n131 = call "MLLF_WriteToBuffer.vi"("String"=w445, "DriverConnect in"=w449) -> ("error out"=w447:T15, "DriverConnect out"=w448:T7)  [unwired: 6 in]
              n132 = call "RS_SMBV100A_Error_check.vi"("Driver Name"=w450, "Error Code"=w451, "Error In"=w447, "DriverConnect in"=w448) -> ("Error Out"=w446:errorcluster)  [unwired: 6 in, 1 out]
            }
            frame "GNSS_CONFIGURATION_ALMANAC_FILE_GPS", "GNSSCONFIGURATION_ALMANACFILE_GPS" {
              w463 = "'" ("string")
              # "Выбор файла АЛЬМАНАХА GPS in GLON"
              n133 = Search and Replace String(replace all?=TRUE, input string=w457, search string="\"", replace string="") -> (result string=w456:string)  [unwired: 4 in, 3 out]
              n134 = Concatenate Strings("/hdd/GNSS/almanac/" ("string"), w456) -> (w461:string)
              n135 = Unbundle By Name(w455) -> ("BASEBAND"=w453:string)
              n136 = Concatenate Strings("SOURce1:BB:" ("string"), w453, ":NAVigation:ALManac:GPS:FILE " ("string"), w463, w461, w463) -> (w464:string)
              n137 = call "MLLF_WriteToBuffer.vi"("String"=w464, "DriverConnect in"=w468) -> ("error out"=w466:T15, "DriverConnect out"=w467:T7)  [unwired: 6 in]
              n138 = call "RS_SMBV100A_Error_check.vi"("Driver Name"=w469, "Error Code"=w470, "Error In"=w466, "DriverConnect in"=w467) -> ("Error Out"=w465:errorcluster)  [unwired: 6 in, 1 out]
            }
            frame "GNSS_CONFIGURATION_RINEX_FILE_GAL", "GNSSCONFIGURATION_RINEXFILE_GAL" {
              w481 = "'" ("string")
              # "Выбор файла GPS RINEX GLON"
              n139 = Search and Replace String(replace all?=TRUE, input string=w475, search string="\"", replace string="") -> (result string=w474:string)  [unwired: 4 in, 3 out]
              n140 = Concatenate Strings("/hdd/GNSS/rinex/" ("string"), w474) -> (w479:string)
              n141 = Unbundle By Name(w472) -> ("BASEBAND"=w473:string)
              n142 = Concatenate Strings("SOURce1:BB:" ("string"), w473, ":RIN:ALM:GAL:FILE " ("string"), w481, w479, w481) -> (w482:string)
              n143 = call "MLLF_WriteToBuffer.vi"("String"=w482, "DriverConnect in"=w487) -> ("error out"=w485:T15, "DriverConnect out"=w486:T7)  [unwired: 6 in]
              n144 = call "RS_SMBV100A_Error_check.vi"("Driver Name"=w488, "Error Code"=w489, "Error In"=w485, "DriverConnect in"=w486) -> ("Error Out"=w484:errorcluster)  [unwired: 6 in, 1 out]
            }
            frame "GNSS_CONFIGURATION_RINEXFILE_GLONASS", "GNSSCONFIGURATION_RINEXFILE_GLONASS" {
              w500 = "'" ("string")
              # "Выбор файла GPS RINEX GLON"
              n145 = Search and Replace String(replace all?=TRUE, input string=w494, search string="\"", replace string="") -> (result string=w493:string)  [unwired: 4 in, 3 out]
              n146 = Concatenate Strings("/hdd/GNSS/rinex/" ("string"), w493) -> (w498:string)
              n147 = Unbundle By Name(w491) -> ("BASEBAND"=w492:string)
              n148 = Concatenate Strings("SOURce1:BB:" ("string"), w492, ":RIN:ALM:GLON:FILE " ("string"), w500, w498, w500) -> (w501:string)
              n149 = call "MLLF_WriteToBuffer.vi"("String"=w501, "DriverConnect in"=w506) -> ("error out"=w504:T15, "DriverConnect out"=w505:T7)  [unwired: 6 in]
              n150 = call "RS_SMBV100A_Error_check.vi"("Driver Name"=w507, "Error Code"=w508, "Error In"=w504, "DriverConnect in"=w505) -> ("Error Out"=w503:errorcluster)  [unwired: 6 in, 1 out]
            }
            frame "GNSS_CONFIGURATION_RINEX_FILE_GPS", "GNSSCONFIGURATION_RINEXFILE_GPS" {
              w519 = "'" ("string")
              # "Выбор файла GPS RINEX GLON"
              n151 = Search and Replace String(replace all?=TRUE, input string=w513, search string="\"", replace string="") -> (result string=w512:string)  [unwired: 4 in, 3 out]
              n152 = Concatenate Strings("/hdd/GNSS/rinex/" ("string"), w512) -> (w517:string)
              n153 = Unbundle By Name(w510) -> ("BASEBAND"=w511:string)
              n154 = Concatenate Strings("SOURce1:BB:" ("string"), w511, ":RIN:ALM:GPS:FILE " ("string"), w519, w517, w519) -> (w520:string)
              n155 = call "MLLF_WriteToBuffer.vi"("String"=w520, "DriverConnect in"=w525) -> ("error out"=w523:T15, "DriverConnect out"=w524:T7)  [unwired: 6 in]
              n156 = call "RS_SMBV100A_Error_check.vi"("Driver Name"=w526, "Error Code"=w527, "Error In"=w523, "DriverConnect in"=w524) -> ("Error Out"=w522:errorcluster)  [unwired: 6 in, 1 out]
            }
            frame "GNSS_CONFIGURATION_RINEX_FILE_GAL_STATE", "GNSSCONFIGURATION_RINEXFILE_GAL_STATE" {
              # "SOUR:BB:GLON:NAV:RIN:GAL:STAT OFF"
              # "Активировать\\Деактивировать GPS файла RINEX GLON"
              n157 = Unbundle By Name(w534) -> ("BASEBAND"=w536:string)
              n158 = call "MLLF_ParameterSelect.vi"("Command to equipment"=string[] ["ON\n", "OFF"], "Names"=string[][] [["ON", "1", "ENABLE", "EN"], ["OFF", "0", "DISABLE", "DIS"]], "Input"=w531, "Command"=w530, "Driver Name"=w529, "Error Code"=w528) -> ("Choice"=w533:string, "Error Out"=w541:errorcluster)  [unwired: 8 in]
              n159 = Concatenate Strings("SOUR:BB:", w536, ":NAV:RIN:GAL:STAT ", w533) -> (w532:string)
              n160 = call "MLLF_WriteToBuffer.vi"("String"=w532, "error in"=w541, "DriverConnect in"=w538) -> ("error out"=w539:T15, "DriverConnect out"=w540:T7)  [unwired: 5 in]
              n161 = call "RS_SMBV100A_Error_check.vi"("Driver Name"=w529, "Error Code"=w528, "Error In"=w539, "DriverConnect in"=w540) -> ("Error Out"=w544:errorcluster)  [unwired: 6 in, 1 out]
            }
            frame "GNSS_CONFIGURATION_RINEX_FILE_GLONASS_STATE", "GNSSCONFIGURATION_RINEXFILE_GLONASS_STATE" {
              # "SOUR:BB:GLON:NAV:RIN:GAL:STAT OFF"
              # "Активировать\\Деактивировать GPS файла RINEX GLON"
              n162 = Unbundle By Name(w551) -> ("BASEBAND"=w553:string)
              n163 = call "MLLF_ParameterSelect.vi"("Command to equipment"=string[] ["ON\n", "OFF"], "Names"=string[][] [["ON", "1", "ENABLE", "EN"], ["OFF", "0", "DISABLE", "DIS"]], "Input"=w548, "Command"=w547, "Driver Name"=w546, "Error Code"=w545) -> ("Choice"=w550:string, "Error Out"=w558:errorcluster)  [unwired: 8 in]
              n164 = Concatenate Strings("SOUR:BB:", w553, ":NAV:RIN:GLON:STAT ", w550) -> (w549:string)
              n165 = call "MLLF_WriteToBuffer.vi"("String"=w549, "error in"=w558, "DriverConnect in"=w555) -> ("error out"=w556:T15, "DriverConnect out"=w557:T7)  [unwired: 5 in]
              n166 = call "RS_SMBV100A_Error_check.vi"("Driver Name"=w546, "Error Code"=w545, "Error In"=w556, "DriverConnect in"=w557) -> ("Error Out"=w561:errorcluster)  [unwired: 6 in, 1 out]
            }
            frame "GNSS_CONFIGURATION_RINEX_FILE_GPS_STATE", "GNSSCONFIGURATION_RINEXFILE_GPS_STATE" {
              # "SOUR:BB:GLON:NAV:RIN:GAL:STAT OFF"
              # "Активировать\\Деактивировать GPS файла RINEX GLON"
              n167 = Unbundle By Name(w568) -> ("BASEBAND"=w570:string)
              n168 = call "MLLF_ParameterSelect.vi"("Command to equipment"=string[] ["ON\n", "OFF"], "Names"=string[][] [["ON", "1", "ENABLE", "EN"], ["OFF", "0", "DISABLE", "DIS"]], "Input"=w565, "Command"=w562, "Driver Name"=w564, "Error Code"=w563) -> ("Choice"=w567:string, "Error Out"=w575:errorcluster)  [unwired: 8 in]
              n169 = Concatenate Strings("SOUR:BB:", w570, ":NAV:RIN:GPS:STAT ", w567) -> (w566:string)
              n170 = call "MLLF_WriteToBuffer.vi"("String"=w566, "error in"=w575, "DriverConnect in"=w572) -> ("error out"=w573:T15, "DriverConnect out"=w574:T7)  [unwired: 5 in]
              n171 = call "RS_SMBV100A_Error_check.vi"("Driver Name"=w564, "Error Code"=w563, "Error In"=w573, "DriverConnect in"=w574) -> ("Error Out"=w578:errorcluster)  [unwired: 6 in, 1 out]
            }
            frame "GLONASS_LOAD_SCENARIO" {
              w600 = "'" ("string")
              # "Осуществляется подгрузка и в прибор и в драйвер сценария."
              # "загружаем сценарий для локации GLON"
              n172 = Search and Replace String(replace all?=TRUE, input string=w581, search string="\"", replace string="") -> (result string=w580:string)  [unwired: 4 in, 3 out]
              n173 = Concatenate Strings("GNSS\\scenario\\", w580, ".txt") -> (w590:string)
              n174 = Build Path(base path=w579, name or relative path=w590) -> (appended path=w585:path)
              n175 = Concatenate Strings("/hdd/GNSS/scenario/", w580, ".txt") -> (w586:string)
              n176 = Read from Text File(file (use dialog)=w585) -> (text=w604:string, error out=w595:errorcluster)  [unwired: 3 in, 2 out]
              n177 = Bundle By Name(cluster=w603, "GLONASS SCENARIO"=w604) -> (w602:T12)
              n178 = Concatenate Strings("SOUR:BB:GLON:LOC:WAYP:FILE " ("string"), w600, w586, w600) -> (w597:string)
              n179 = call "MLLF_WriteToBuffer.vi"("String"=w597, "error in"=w595, "DriverConnect in"=w596) -> ("error out"=w598:T15, "DriverConnect out"=w599:T7)  [unwired: 5 in]
              n180 = call "RS_SMBV100A_Error_check.vi"("Driver Name"=w592, "Error Code"=w593, "Error In"=w598, "DriverConnect in"=w599) -> ("Error Out"=w594:errorcluster)  [unwired: 6 in, 1 out]
            }
            frame "GLONASS_LOAD_WAYPOINTS" {
              # "Импортируем WAyPOINTS в драйвер"
              n181 = Search and Replace String(replace all?=TRUE, input string=w606, search string="\"", replace string="") -> (result string=w607:string)  [unwired: 4 in, 3 out]
              n182 = Concatenate Strings("GNSS\\waypoints\\", w607, ".txt") -> (w619:string)
              n183 = Build Path(base path=w605, name or relative path=w619) -> (appended path=w617:path)
              n184 = Read from Text File(file (use dialog)=w617) -> (text=w614:string, error out=w613:errorcluster)  [unwired: 3 in, 2 out]
              n185 = call "RS_SMBV100A_arrayStringToDOUBLE.vi"("string"=w614, "error in"=w613) -> ("Dynam waypoints"=w611:T5, "error out"=w612:errorcluster)  [unwired: 1 in]
              n186 = Bundle By Name(cluster=w616, "GLONASS WAYPOINTS"=w611) -> (w615:T12)
            }
            frame "------------------------------------ LOCALIZATION_DATA -----------------------------------" {
            }
            frame "LOCALIZATION_DATA_GEOGRAPHYCLOCATION", "LOCALIZATIONDATA_GEOGRAPHYCLOCATION" {
              # "выбираем позицию GLON приемника"
              n187 = Unbundle By Name(w629) -> ("BASEBAND"=w628:string)
              n188 = call "MLLF_ParameterSelect.vi"("Command to equipment"=string[] ["\"Waypoints\"", "\"User Defined\"", "\"New York\"", "\"BEIJING\"", "\"SEOUL\"", "\"SINGAPORE\"", "\"TAIPEI\"", "\"TOKYO\"", "\"SYDNEY\"", "\"LONDON\"", "\"MOSCOW\"", "\"MUNICH\"", "\"PARIS\""], "Names"=string[][] [["WAIPOINTS", "", ""], ["USER_DEFINE", "USER", "USER DEFINE"], ["NEW YORK", "NEW_YORK", ""], ["BEIJING", "", ""], ["SEOUL", "", ""], ["SINGAPORE", "", ""], ["TAIPEI", "", ""], ["TOKYO", "", ""], ["SYDNEY", "", ""], ["LONDON", "", ""], ["MOSCOW", "", ""], ["MUNICH", "", ""], ["PARIS", "", ""]], "Input"=w623, "Command"=w622, "Driver Name"=w634, "Error Code"=w635) -> ("Choice"=w625:string, "Error Out"=w636:errorcluster)  [unwired: 8 in]
              n189 = Concatenate Strings("SOUR:BB:", w628, ":LOC:SEL ", w625) -> (w624:string)
              n190 = call "MLLF_WriteToBuffer.vi"("String"=w624, "error in"=w636, "DriverConnect in"=w633) -> ("error out"=w631:T15, "DriverConnect out"=w632:T7)  [unwired: 5 in]
              n191 = call "RS_SMBV100A_Error_check.vi"("Driver Name"=w634, "Error Code"=w635, "Error In"=w631, "DriverConnect in"=w632) -> ("Error Out"=w630:errorcluster)  [unwired: 6 in, 1 out]
            }
            frame "LOCALIZATION_DATA_POSITION", "LOCALIZATIONDATA_POSITION" {
              w651 = ", " ("string")
              w653 = " %.;%1.7f" ("format")
              # "вот так правильно!"
              # "Позиция GLON приемника при USER DEFINE <Latitude> ,<Longitude>,<Altitude>"
              n192 = call "MLLF_FormatStringValue.vi"("String Value"=w641, "Format"=w653) -> ("error out"=w650:T15, "String Value Formated"=w645:T16)  [unwired: 7 in, 1 out]
              n193 = Unbundle By Name(w644) -> ("BASEBAND"=w642:string)
              n194 = call "MLLF_FormatStringValue.vi"("error in"=w650, "String Value"=w640, "Format"=w653) -> ("error out"=w649:T15, "String Value Formated"=w646:T16)  [unwired: 6 in, 1 out]
              n195 = call "MLLF_FormatStringValue.vi"("error in"=w649, "String Value"=w639, "Format"=w653) -> ("error out"=w648:T15, "String Value Formated"=w652:T16)  [unwired: 6 in, 1 out]
              n196 = Concatenate Strings("SOUR:BB:", w642, ":LOC:COOR:DEC " ("string"), w646, w651, w645, w651, w652) -> (w647:string)
              n197 = call "MLLF_WriteToBuffer.vi"("String"=w647, "error in"=w648, "DriverConnect in"=w658) -> ("error out"=w656:T15, "DriverConnect out"=w657:T7)  [unwired: 5 in]
              n198 = call "RS_SMBV100A_Error_check.vi"("Driver Name"=w659, "Error Code"=w660, "Error In"=w656, "DriverConnect in"=w657) -> ("Error Out"=w655:errorcluster)  [unwired: 6 in, 1 out]
            }
            frame "LOCALIZATION_DATA_READ_OUTMODE", "LOCALIZATIONDATA_READOUTMODE" {
              # "Использование сценария GLON"
              n199 = Unbundle By Name(w663) -> ("BASEBAND"=w664:string)
              n200 = call "MLLF_ParameterSelect.vi"("Command to equipment"=string[] ["CYCL", "OWAY", "RTR"], "Names"=string[][] [["CYCLE", "CYCLIC", ""], ["ONE WAY", "ONE", "OWAY"], ["ROUND TRIP", "ROUND", "RTR"]], "Input"=w662, "Command"=w661, "Driver Name"=w673, "Error Code"=w674) -> ("Choice"=w666:string, "Error Out"=w675:errorcluster)  [unwired: 8 in]
              n201 = Concatenate Strings("SOUR:BB:", w664, ":LOC:WAYP:ROM ", w666) -> (w665:string)
              n202 = call "MLLF_WriteToBuffer.vi"("String"=w665, "error in"=w675, "DriverConnect in"=w672) -> ("error out"=w670:T15, "DriverConnect out"=w671:T7)  [unwired: 5 in]
              n203 = call "RS_SMBV100A_Error_check.vi"("Driver Name"=w673, "Error Code"=w674, "Error In"=w670, "DriverConnect in"=w671) -> ("Error Out"=w669:errorcluster)  [unwired: 6 in, 1 out]
            }
            frame "LOCALIZATION_DATA_REFERENCE_FRAME", "LOCALIZATIONDATA_REFERENCEFRAME" {
              # "Использование сценария GLON"
              n204 = Unbundle By Name(w680) -> ("BASEBAND"=w683:string)
              n205 = call "MLLF_ParameterSelect.vi"("Command to equipment"=string[] ["WGS84", "PZ90"], "Names"=string[][] [["WGS84", "WGS_84", "WGS-84"], ["PZ90", "PZ_90", "PZ-90"]], "Input"=w679, "Command"=w678, "Driver Name"=w690, "Error Code"=w691) -> ("Choice"=w682:string, "Error Out"=w692:errorcluster)  [unwired: 8 in]
              n206 = Concatenate Strings("SOUR:BB:", w683, ":LOC:COOR:RFR ", w682) -> (w681:string)
              n207 = call "MLLF_WriteToBuffer.vi"("String"=w681, "error in"=w692, "DriverConnect in"=w689) -> ("error out"=w687:T15, "DriverConnect out"=w688:T7)  [unwired: 5 in]
              n208 = call "RS_SMBV100A_Error_check.vi"("Driver Name"=w690, "Error Code"=w691, "Error In"=w687, "DriverConnect in"=w688) -> ("Error Out"=w686:errorcluster)  [unwired: 6 in, 1 out]
            }
            frame "LOCALIZATION_DATA_SMOOTH_MOVEMENT", "LOCALIZATIONDATA_SMOOTHMOVEMENT" {
              # "Активировать функцию Smooth Movement"
              n209 = Unbundle By Name(w699) -> ("BASEBAND"=w702:string)
              n210 = call "MLLF_ParameterSelect.vi"("Command to equipment"=string[] ["ON\n", "OFF"], "Names"=string[][] [["ON", "1", "ENABLE", "EN"], ["OFF", "0", "DISABLE", "DIS"]], "Input"=w698, "Command"=w697, "Driver Name"=w696, "Error Code"=w695) -> ("Choice"=w701:string, "Error Out"=w708:errorcluster)  [unwired: 8 in]
              n211 = Concatenate Strings("SOUR:BB:", w702, ":LOC:SMOV ", w701) -> (w700:string)
              n212 = call "MLLF_WriteToBuffer.vi"("String"=w700, "error in"=w708, "DriverConnect in"=w705) -> ("error out"=w706:T15, "DriverConnect out"=w707:T7)  [unwired: 5 in]
              n213 = call "RS_SMBV100A_Error_check.vi"("Driver Name"=w696, "Error Code"=w695, "Error In"=w706, "DriverConnect in"=w707) -> ("Error Out"=w711:errorcluster)  [unwired: 6 in, 1 out]
            }
            frame "LOCALIZATION_DATA_WAIPOINTS", "LOCALIZATIONDATA_WAIPOINTS" {
              w723 = "'" ("string")
              # "Выбор файла сценария GPS приемника"
              n214 = Search and Replace String(replace all?=TRUE, input string=w716, search string="\"", replace string="") -> (result string=w715:string)  [unwired: 4 in, 3 out]
              n215 = Unbundle By Name(w714) -> ("BASEBAND"=w713:string)
              n216 = Concatenate Strings("/hdd/GNSS/scenario/" ("string"), w715, ".txt" ("string")) -> (w720:string)
              n217 = Concatenate Strings("SOUR:BB:", w713, ":LOC:WAYP:FILE " ("string"), w723, w720, w723) -> (w724:string)
              n218 = call "MLLF_WriteToBuffer.vi"("String"=w724, "DriverConnect in"=w729) -> ("error out"=w727:T15, "DriverConnect out"=w728:T7)  [unwired: 6 in]
              n219 = call "RS_SMBV100A_Error_check.vi"("Driver Name"=w730, "Error Code"=w731, "Error In"=w727, "DriverConnect in"=w728) -> ("Error Out"=w726:errorcluster)  [unwired: 6 in, 1 out]
            }
            frame "RFBAND" {
              # "Настройка частоты GLONASS грожданская/военная"
              n220 = Unbundle By Name(w735) -> ("BASEBAND"=w736:string)
              n221 = call "MLLF_ParameterSelect.vi"("Command to equipment"=string[] ["L1", "L2"], "Names"=string[][] [["L1", "L1/E2"], ["L2", ""]], "Input"=w732, "Driver Name"=w743, "Error Code"=w744) -> ("Choice"=w733:string, "Error Out"=w745:errorcluster)  [unwired: 9 in]
              n222 = Concatenate Strings("BB:", w736, ":RFB ", w733) -> (w734:string)
              n223 = call "MLLF_WriteToBuffer.vi"("String"=w734, "error in"=w745, "DriverConnect in"=w742) -> ("error out"=w740:T15, "DriverConnect out"=w741:T7)  [unwired: 5 in]
              n224 = call "RS_SMBV100A_Error_check.vi"("Driver Name"=w743, "Error Code"=w744, "Error In"=w740, "DriverConnect in"=w741) -> ("Error Out"=w739:errorcluster)  [unwired: 6 in, 1 out]
            }
            frame "TimeProjectionOfNavigationData" {
              # "<subsystem>:SVID<ch>:<GNSS>:NMESsage:\nRTPRojection."
              n225 = Unbundle By Name(w752) -> ("BASEBAND"=w755:string)
              n226 = call "MLLF_ParameterSelect.vi"("Command to equipment"=string[] ["ON\n", "OFF"], "Names"=string[][] [["ON", "1", "ENABLE", "EN"], ["OFF", "0", "DISABLE", "DIS"]], "Input"=w751, "Command"=w750, "Driver Name"=w749, "Error Code"=w748) -> ("Choice"=w753:string, "Error Out"=w762:errorcluster)  [unwired: 8 in]
              n227 = Concatenate Strings("SOURce1:BB:", w755, ":SATellite:GRTProjection ", w753) -> (w754:string)
              n228 = call "MLLF_WriteToBuffer.vi"("String"=w754, "error in"=w762, "DriverConnect in"=w759) -> ("error out"=w760:T15, "DriverConnect out"=w761:T7)  [unwired: 5 in]
              n229 = call "RS_SMBV100A_Error_check.vi"("Driver Name"=w749, "Error Code"=w748, "Error In"=w760, "DriverConnect in"=w761) -> ("Error Out"=w758:errorcluster)  [unwired: 6 in, 1 out]
            }
            frame "------------------------ SATELLITE_CONFIGURATIONS ---------------------------" {
            }
            frame "SATELLITE_CONFIGURATIONS_ELEVATION_MASK", "SATELLITECONFIGURATIONS_ELEVATIONMASK" {
              # "Угол отсечки по GLON"
              n230 = Unbundle By Name(w769) -> ("BASEBAND"=w770:string)
              n231 = call "MLLF_ParameterSelect.vi"("Command to equipment"=string[] ["0", "2.5", "5", "7.5", "10"], "Names"=string[][] [["0", ""], ["2.5", "2,5"], ["5", ""], ["7.5", "7,5"], ["10", ""]], "Input"=w766, "Driver Name"=w775, "Error Code"=w774) -> ("Choice"=w768:string, "Error Out"=w773:errorcluster)  [unwired: 9 in]
              n232 = Concatenate Strings("SOUR:BB:", w770, ":SEM ", w768) -> (w767:string)
              n233 = call "MLLF_WriteToBuffer.vi"("String"=w767, "error in"=w773, "DriverConnect in"=w781) -> ("error out"=w779:T15, "DriverConnect out"=w780:T7)  [unwired: 5 in]
              n234 = call "RS_SMBV100A_Error_check.vi"("Driver Name"=w775, "Error Code"=w774, "Error In"=w779, "DriverConnect in"=w780) -> ("Error Out"=w778:errorcluster)  [unwired: 6 in, 1 out]
            }
            frame "SATELLITECONFIGURATIONS_GETOPTIMALCONSTELATION" {
              # "Установить оптимальную конфигурацию спутников"
              n235 = Unbundle By Name(w782) -> ("BASEBAND"=w784:string)
              n236 = Concatenate Strings("SOUR:BB:", w784, ":GOC ") -> (w783:string)
              n237 = call "MLLF_WriteToBuffer.vi"("String"=w783, "DriverConnect in"=w790) -> ("error out"=w788:T15, "DriverConnect out"=w789:T7)  [unwired: 6 in]
              n238 = call "RS_SMBV100A_Error_check.vi"("Driver Name"=w791, "Error Code"=w792, "Error In"=w788, "DriverConnect in"=w789) -> ("Error Out"=w787:errorcluster)  [unwired: 6 in, 1 out]
            }
            frame "SATELLITECONFIGURATIONS_MAXIMUMNUMBEROFSATELLITES" {
              # "Колличество спутников В модуле GLON"
              n239 = Unbundle By Name(w795) -> ("BASEBAND"=w798:string)
              n240 = call "MLLF_ParameterSelect.vi"("Command to equipment"=string[] ["1", "4", "5", "6", "7", "8", "9", "10", "11", "12", "13", "14", "15", "16", "17", "18", "19", "20", "21", "22", "23", "24"], "Names"=string[][] [["1"], ["4"], ["5"], ["6"], ["7"], ["8"], ["9"], ["10"], ["11"], ["12"], ["13"], ["14"], ["15"], ["16"], ["17"], ["18"], ["19"], ["20"], ["21"], ["22"], ["23"], ["24"]], "Input"=w794, "Command"=w793, "Driver Name"=w805, "Error Code"=w806) -> ("Choice"=w796:string, "Error Out"=w807:errorcluster)  [unwired: 8 in]
              n241 = Concatenate Strings("SOUR:BB:", w798, ":SAT:COUNT ", w796) -> (w797:string)
              n242 = call "MLLF_WriteToBuffer.vi"("String"=w797, "error in"=w807, "DriverConnect in"=w804) -> ("error out"=w802:T15, "DriverConnect out"=w803:T7)  [unwired: 5 in]
              n243 = call "RS_SMBV100A_Error_check.vi"("Driver Name"=w805, "Error Code"=w806, "Error In"=w802, "DriverConnect in"=w803) -> ("Error Out"=w801:errorcluster)  [unwired: 6 in, 1 out]
            }
            frame "SATELLITECONFIGURATIONS_PseudorangeBias" {
              # "Функции настройки ephemeris в локации GPS - TOE"
              n244 = Unbundle By Name(w814) -> ("BASEBAND"=w812:string)
              n245 = call "RS_SMBV100A_N_in_SKY_to_SAT_in_DEVICE.vi"("DriverConnect in"=w824, "BASEBAND"=w812, "String Value"=w811) -> ("DriverConnect out"=w820:T7, "SAT"=w815:dbl, "Error Out"=w819:errorcluster)  [unwired: 8 in, 2 out]
              n246 = Format Into String(format string="%.;%1.0f" ("format"), error in=w819, w815) -> (resulting string=w816:string, error out=w818:errorcluster)  [unwired: 1 in]
              n247 = Concatenate Strings("SOUR:BB:", w812, ":SATellite" ("regular expression"), w816, ":PRBias " ("regular expression"), w810) -> (w821:string)
              n248 = call "MLLF_WriteToBuffer.vi"("String"=w821, "error in"=w818, "DriverConnect in"=w820) -> ("error out"=w826:T15, "DriverConnect out"=w827:T7)  [unwired: 5 in]
              n249 = call "RS_SMBV100A_Error_check.vi"("Driver Name"=w828, "Error Code"=w829, "Error In"=w826, "DriverConnect in"=w827) -> ("Error Out"=w825:errorcluster)  [unwired: 6 in, 1 out]
            }
            frame "SATELLITECONFIGURATIONS_POWERMODE" {
              # "Модуль мощности GLON"
              n250 = Unbundle By Name(w832) -> ("BASEBAND"=w835:string)
              n251 = call "MLLF_ParameterSelect.vi"("Command to equipment"=string[] ["USER", "AUTO"], "Names"=string[][] [["USER"], ["AUTO"]], "Input"=w831, "Command"=w830, "Driver Name"=w844, "Error Code"=w845) -> ("Choice"=w834:string, "Error Out"=w846:errorcluster)  [unwired: 8 in]
              n252 = Concatenate Strings("SOUR:BB:", w835, ":POW:MODE ", w834) -> (w833:string)
              n253 = call "MLLF_WriteToBuffer.vi"("String"=w833, "error in"=w846, "DriverConnect in"=w843) -> ("error out"=w841:T15, "DriverConnect out"=w842:T7)  [unwired: 5 in]
              n254 = call "RS_SMBV100A_Error_check.vi"("Driver Name"=w844, "Error Code"=w845, "Error In"=w841, "DriverConnect in"=w842) -> ("Error Out"=w840:errorcluster)  [unwired: 6 in, 1 out]
            }
            frame "SATELLITECONFIGURATIONS_REFPOWER" {
              # "от -145 до 20 dBm"
              # "Опорная Мощность по GLON"
              n255 = call "MLLF_FormatStringValue.vi"("String Value"=w847, "Format"=" %.;%1.2f" ("format")) -> ("error out"=w852:T15, "String Value Formated"=w853:T16)  [unwired: 7 in, 1 out]
              n256 = Unbundle By Name(w848) -> ("BASEBAND"=w849:string)
              n257 = Concatenate Strings("SOUR:BB:", w849, ":POW:REF:POW " ("string"), w853) -> (w851:string)
              n258 = call "MLLF_WriteToBuffer.vi"("String"=w851, "error in"=w852, "DriverConnect in"=w859) -> ("error out"=w857:T15, "DriverConnect out"=w858:T7)  [unwired: 5 in]
              n259 = call "RS_SMBV100A_Error_check.vi"("Driver Name"=w860, "Error Code"=w861, "Error In"=w857, "DriverConnect in"=w858) -> ("Error Out"=w856:errorcluster)  [unwired: 6 in, 1 out]
            }
            frame "SATELLITECONFIGURATIONS_REFSATELLITE" {
              # "!!!!!!!!!!!!!!!! N.A. -  устанавливается по умолчанию при сбросе\nНО не выставляется из CASE!!! так как указано в документации\n!!!!!!!!!!!!!!!!!!!!!!!!!!!!!!!!!!!!!!!!!!!!!!!!!!!!!!!!!!!!!!!!!!!!!!!!!!!!!!!!!\nПроизводители вкурсе ИХ КАСЯК!!!"
              # "Опорный спутник по мощности GLON"
              n260 = Unbundle By Name(w865) -> ("BASEBAND"=w866:string)
              n261 = call "MLLF_ParameterSelect.vi"("Command to equipment"=string[] ["-1", "1", "2", "3", "4", "5", "6", "7", "8", "9", "10", "11", "12", "13", "14", "15", "16", "17", "18", "19", "20", "21", "22", "23", "24"], "Names"=string[][] [["N.A.", "NA"], ["1", ""], ["2", ""], ["3", ""], ["4", ""], ["5", ""], ["6", ""], ["7", ""], ["8", ""], ["9", ""], ["10", ""], ["11", ""], ["12", ""], ["13", ""], ["14", ""], ["15", ""], ["16", ""], ["17", ""], ["18", ""], ["19", ""], ["20", ""], ["21", ""], ["22", ""], ["23", ""], ["24", ""]], "Input"=w862, "Driver Name"=w875, "Error Code"=w876) -> ("Choice"=w863:string, "Error Out"=w877:errorcluster)  [unwired: 9 in]
              n262 = Concatenate Strings("SOUR:BB:", w866, ":POW:REF:SAT ", w863) -> (w864:string)
              n263 = call "MLLF_WriteToBuffer.vi"("String"=w864, "error in"=w877, "DriverConnect in"=w874) -> ("error out"=w872:T15, "DriverConnect out"=w873:T7)  [unwired: 5 in]
              n264 = call "RS_SMBV100A_Error_check.vi"("Driver Name"=w875, "Error Code"=w876, "Error In"=w872, "DriverConnect in"=w873) -> ("Error Out"=w871:errorcluster)  [unwired: 6 in, 1 out]
            }
            frame "SATELLITECONFIGURATIONS_REFSTANDART" {
              # "SOUR:BB:GLON:POW:REF:STAN GAL"
              # "Опорный стандарт по мощности GLON"
              n265 = Unbundle By Name(w879) -> ("BASEBAND"=w882:string)
              n266 = call "MLLF_ParameterSelect.vi"("Command to equipment"=string[] ["GPS", "GLON", "GAL"], "Names"=string[][] [["GPS"], ["GLONASS"], ["GALILEO"]], "Input"=w878, "Driver Name"=w891, "Error Code"=w892) -> ("Choice"=w880:string, "Error Out"=w893:errorcluster)  [unwired: 9 in]
              n267 = Concatenate Strings("SOUR:BB:", w882, ":POW:REF:STAN ", w880) -> (w881:string)
              n268 = call "MLLF_WriteToBuffer.vi"("String"=w881, "error in"=w893, "DriverConnect in"=w890) -> ("error out"=w888:T15, "DriverConnect out"=w889:T7)  [unwired: 5 in]
              n269 = call "RS_SMBV100A_Error_check.vi"("Driver Name"=w891, "Error Code"=w892, "Error In"=w888, "DriverConnect in"=w889) -> ("Error Out"=w887:errorcluster)  [unwired: 6 in, 1 out]
            }
            frame "SIMULATIONMODE", "SMODE" {
              # "SOUR:BB:GLON:SMOD  USER"
              # "Выбор симуляции GLONASS статический\\автоматический\\пользовательский"
              n270 = Unbundle By Name(w897) -> ("BASEBAND"=w898:string)
              n271 = call "MLLF_ParameterSelect.vi"("Command to equipment"=string[] ["STAT", "AUTO", "USER"], "Names"=string[][] [["STATIC"], ["AUTO"], ["USER"]], "Input"=w894, "Driver Name"=w905, "Error Code"=w906) -> ("Choice"=w895:string, "Error Out"=w907:errorcluster)  [unwired: 9 in]
              n272 = Concatenate Strings("SOUR:BB:", w898, ":SMOD ", w895) -> (w896:string)
              n273 = call "MLLF_WriteToBuffer.vi"("String"=w896, "error in"=w907, "DriverConnect in"=w904) -> ("error out"=w902:T15, "DriverConnect out"=w903:T7)  [unwired: 5 in]
              n274 = call "RS_SMBV100A_Error_check.vi"("Driver Name"=w905, "Error Code"=w906, "Error In"=w902, "DriverConnect in"=w903) -> ("Error Out"=w901:errorcluster)  [unwired: 6 in, 1 out]
            }
            frame "----------------------------  SIMULATION_START_TIME ----------------------------------------" {
            }
            frame "SIMULATION_START_TIME", "SIMULATIONSTARTTIME" {
              # "SOUR:BB:GLON:NAV:SIM:TBAS UTC"
              # "Формат времени GLON"
              n275 = Unbundle By Name(w915) -> ("BASEBAND"=w918:string)
              n276 = call "MLLF_ParameterSelect.vi"("Command to equipment"=string[] ["UTC", "GLO", "GPS"], "Names"=string[][] [["UTC", ""], ["GLO", "GLONASS"], ["GPS", ""]], "Input"=w914, "Command"=w913, "Driver Name"=w912, "Error Code"=w911) -> ("Choice"=w916:string, "Error Out"=w924:errorcluster)  [unwired: 8 in]
              n277 = Concatenate Strings("SOUR:BB:", w918, ":NAV:SIM:TBAS ", w916) -> (w917:string)
              n278 = call "MLLF_WriteToBuffer.vi"("String"=w917, "error in"=w924, "DriverConnect in"=w923) -> ("error out"=w921:T15, "DriverConnect out"=w922:T7)  [unwired: 5 in]
              n279 = call "RS_SMBV100A_Error_check.vi"("Driver Name"=w912, "Error Code"=w911, "Error In"=w921, "DriverConnect in"=w922) -> ("Error Out"=w927:errorcluster)  [unwired: 6 in, 1 out]
            }
            frame "SIMULATIONSTARTTIME_DATE" {
              # "SOUR:BB:GLON:NAV:SIM:DATE %,;%<%Y,%m,%d>T"
              # "Вносим дату времени GLON"
              n280 = Search and Replace String(replace all?=TRUE, input string=w934, search string=".", replace string=",") -> (result string=w936:string, error out=w935:errorcluster)  [unwired: 4 in, 2 out]
              n281 = Unbundle By Name(w930) -> ("BASEBAND"=w931:string)
              n282 = Scan From String(format string="%.;%<%d,%m,%Y>T", input string=w936, error in=w935) -> (error out=w940:errorcluster, output 1=w943:timestamp)  [unwired: 2 in, 2 out]
              n283 = Format Into String(format string="%,;%<%Y,%m,%d>T", error in=w940, w943) -> (resulting string=w929:string, error out=w941:errorcluster)  [unwired: 1 in]
              n284 = Concatenate Strings("SOUR:BB:", w931, ":NAV:SIM:DATE ", w929) -> (w928:string)
              n285 = call "MLLF_WriteToBuffer.vi"("String"=w928, "error in"=w941, "DriverConnect in"=w947) -> ("error out"=w945:T15, "DriverConnect out"=w946:T7)  [unwired: 5 in]
              n286 = call "RS_SMBV100A_Error_check.vi"("Driver Name"=w949, "Error Code"=w950, "Error In"=w945, "DriverConnect in"=w946) -> ("Error Out"=w948:errorcluster)  [unwired: 6 in, 1 out]
            }
            frame "SIMULATIONSTARTTIME_TIME" {
              w966 = " %.;%1.3f" ("format")
              # "SOUR:BB:GLON:NAV:SIM:TIME %.;%<%H,%M,%S%5u>T"
              # "string               sec     sec"
              # "GLONASS_SIMULATIONSTARTTIME_TIME= 05,00,00.000 3456 -34551"
              # "Вносим время времени GLON"
              n287 = Unbundle By Name(w953) -> ("BASEBAND"=w954:string)
              n288 = Match Pattern(string=w958, regular expression="[\\s\\t]+") -> (before substring=w962:string, after substring=w967:string)  [unwired: 1 in, 2 out]
              n289 = Match Pattern(string=w967, regular expression="[\\s\\t]+") -> (before substring=w964:string, after substring=w963:string)  [unwired: 1 in, 2 out]
              n290 = call "MLLF_FormatStringValue.vi"("String Value"=w964, "Format"=w966) -> ("error out"=w965:T15, "number"=w960:dbl)  [unwired: 7 in, 1 out]
              n291 = call "MLLF_FormatStringValue.vi"("error in"=w965, "String Value"=w963, "Format"=w966) -> ("error out"=w961:T15, "number"=w959:dbl)  [unwired: 6 in, 1 out]
              n292 = Scan From String(format string="%.;%<%H,%M,%S%5u>T", input string=w962, error in=w961) -> (error out=w972:errorcluster, output 1=w973:timestamp)  [unwired: 2 in, 2 out]
              n293 = Add(x=w973, y=w960) -> (x+y=w970:timestamp)
              n294 = Add(x=w970, y=w959) -> (x+y=w971:timestamp)
              n295 = Format Into String(format string="%.;%<%H,%M,%S%5u>T", error in=w972, w971) -> (resulting string=w952:string, error out=w957:errorcluster)  [unwired: 1 in]
              n296 = Concatenate Strings("SOUR:BB:", w954, ":NAV:SIM:TIME ", w952) -> (w951:string)
              n297 = call "MLLF_WriteToBuffer.vi"("String"=w951, "error in"=w957, "DriverConnect in"=w978) -> ("error out"=w976:T15, "DriverConnect out"=w977:T7)  [unwired: 5 in]
              n298 = call "RS_SMBV100A_Error_check.vi"("Driver Name"=w980, "Error Code"=w981, "Error In"=w976, "DriverConnect in"=w977) -> ("Error Out"=w979:errorcluster)  [unwired: 6 in, 1 out]
            }
            frame "STATE" {
              # "Включение/выключения модуляции"
              n299 = Unbundle By Name(w984) -> ("BASEBAND"=w987:string)
              n300 = call "MLLF_ParameterSelect.vi"("Command to equipment"=string[] ["ON", "OFF"], "Names"=string[][] [["ON", "1", "ENABLE", "EN"], ["OFF", "0", "DISABLE", "DIS"]], "Input"=w983, "Command"=w982, "Driver Name"=w994, "Error Code"=w995) -> ("Choice"=w986:string, "Error Out"=w996:errorcluster)  [unwired: 8 in]
              n301 = Concatenate Strings("SOUR:BB:", w987, ":STAT ", w986) -> (w985:string)
              n302 = call "MLLF_WriteToBuffer.vi"("String"=w985, "error in"=w996, "DriverConnect in"=w993) -> ("error out"=w991:T15, "DriverConnect out"=w992:T7)  [unwired: 5 in]
              n303 = call "RS_SMBV100A_Error_check.vi"("Driver Name"=w994, "Error Code"=w995, "Error In"=w991, "DriverConnect in"=w992) -> ("Error Out"=w990:errorcluster)  [unwired: 6 in, 1 out]
            }
            frame "-------------------- SYSTEM_CONFIGURATION -----------------------------------" {
            }
            frame "SYSTEM_CONFIGURATION_ANTI_SPOOFING", "SYSTEMCONFIGURATION_ANTI_SPOOFING" {
              # "GLON ANTI-SPOOFING"
              n304 = Unbundle By Name(w1002) -> ("BASEBAND"=w1005:string)
              n305 = call "MLLF_ParameterSelect.vi"("Command to equipment"=string[] ["ON", "OFF"], "Names"=string[][] [["ON", "1", "ENABLE", "EN"], ["OFF", "0", "DISABLE", "DIS"]], "Input"=w1001, "Command"=w1000, "Driver Name"=w1012, "Error Code"=w1013) -> ("Choice"=w1004:string, "Error Out"=w1014:errorcluster)  [unwired: 8 in]
              n306 = Concatenate Strings("SOUR:BB:", w1005, ":SAT:ASP ", w1004) -> (w1003:string)
              n307 = call "MLLF_WriteToBuffer.vi"("String"=w1003, "error in"=w1014, "DriverConnect in"=w1011) -> ("error out"=w1009:T15, "DriverConnect out"=w1010:T7)  [unwired: 5 in]
              n308 = call "RS_SMBV100A_Error_check.vi"("Driver Name"=w1012, "Error Code"=w1013, "Error In"=w1009, "DriverConnect in"=w1010) -> ("Error Out"=w1008:errorcluster)  [unwired: 6 in, 1 out]
            }
            frame "SYSTEM_CONFIGURATION_GLONASS", "SYSTEMCONFIGURATION_GLONASS" {
              # "Подмешиваем спутники GLONASS"
              n309 = Unbundle By Name(w1019) -> ("BASEBAND"=w1022:string)
              n310 = call "MLLF_ParameterSelect.vi"("Command to equipment"=string[] ["ON", "OFF"], "Names"=string[][] [["ON", "1", "ENABLE", "EN"], ["OFF", "0", "DISABLE", "DIS"]], "Input"=w1018, "Command"=w1017, "Driver Name"=w1029, "Error Code"=w1030) -> ("Choice"=w1021:string, "Error Out"=w1031:errorcluster)  [unwired: 8 in]
              n311 = Concatenate Strings("SOUR:BB:", w1022, ":HYBR:GLON:STAT  ", w1021) -> (w1020:string)
              n312 = call "MLLF_WriteToBuffer.vi"("String"=w1020, "error in"=w1031, "DriverConnect in"=w1028) -> ("error out"=w1026:T15, "DriverConnect out"=w1027:T7)  [unwired: 5 in]
              n313 = call "RS_SMBV100A_Error_check.vi"("Driver Name"=w1029, "Error Code"=w1030, "Error In"=w1026, "DriverConnect in"=w1027) -> ("Error Out"=w1025:errorcluster)  [unwired: 6 in, 1 out]
            }
            frame "SYSTEM_CONFIGURATION_GALILEO", "SYSTEMCONFIGURATION_GALILEO" {
              # "Подмешиваем спутники GPS"
              n314 = Unbundle By Name(w1037) -> ("BASEBAND"=w1040:string)
              n315 = call "MLLF_ParameterSelect.vi"("Command to equipment"=string[] ["ON", "OFF"], "Names"=string[][] [["ON", "1", "ENABLE", "EN"], ["OFF", "0", "DISABLE", "DIS"]], "Input"=w1036, "Command"=w1034, "Driver Name"=w1035, "Error Code"=w1047) -> ("Choice"=w1038:string, "Error Out"=w1048:errorcluster)  [unwired: 8 in]
              n316 = Concatenate Strings("SOUR:BB:", w1040, ":HYBR:GAL:STAT  ", w1038) -> (w1039:string)
              n317 = call "MLLF_WriteToBuffer.vi"("String"=w1039, "error in"=w1048, "DriverConnect in"=w1046) -> ("error out"=w1044:T15, "DriverConnect out"=w1045:T7)  [unwired: 5 in]
              n318 = call "RS_SMBV100A_Error_check.vi"("Driver Name"=w1035, "Error Code"=w1047, "Error In"=w1044, "DriverConnect in"=w1045) -> ("Error Out"=w1043:errorcluster)  [unwired: 6 in, 1 out]
            }
            frame "SYSTEM_CONFIGURATION_GPS", "SYSTEMCONFIGURATION_GPS" {
              # "Подмешиваем спутники GPS"
              n319 = Unbundle By Name(w1053) -> ("BASEBAND"=w1056:string)
              n320 = call "MLLF_ParameterSelect.vi"("Command to equipment"=string[] ["ON", "OFF"], "Names"=string[][] [["ON", "1", "ENABLE", "EN"], ["OFF", "0", "DISABLE", "DIS"]], "Input"=w1052, "Command"=w1051, "Driver Name"=w1063, "Error Code"=w1064) -> ("Choice"=w1055:string, "Error Out"=w1065:errorcluster)  [unwired: 8 in]
              n321 = Concatenate Strings("SOUR:BB:", w1056, ":HYBR:GPS:STAT  ", w1055) -> (w1054:string)
              n322 = call "MLLF_WriteToBuffer.vi"("String"=w1054, "error in"=w1065, "DriverConnect in"=w1062) -> ("error out"=w1060:T15, "DriverConnect out"=w1061:T7)  [unwired: 5 in]
              n323 = call "RS_SMBV100A_Error_check.vi"("Driver Name"=w1063, "Error Code"=w1064, "Error In"=w1060, "DriverConnect in"=w1061) -> ("Error Out"=w1059:errorcluster)  [unwired: 6 in, 1 out]
            }
            frame "SYSTEM_CONFIGURATION_USE_COMMON_RF_FREQUENCY", "SYSTEMCONFIGURATION_USECOMMONRFFREQUENCY" {
              # "Используем опорную частоту GLON"
              n324 = Unbundle By Name(w1069) -> ("BASEBAND"=w1072:string)
              n325 = call "MLLF_ParameterSelect.vi"("Command to equipment"=string[] ["ON", "OFF"], "Names"=string[][] [["ON", "1", "ENABLE", "EN"], ["OFF", "0", "DISABLE", "DIS"]], "Input"=w1068, "Driver Name"=w1079, "Error Code"=w1080) -> ("Choice"=w1070:string, "Error Out"=w1081:errorcluster)  [unwired: 9 in]
              n326 = Concatenate Strings("SOUR:BB:", w1072, ":UCRF ", w1070) -> (w1071:string)
              n327 = call "MLLF_WriteToBuffer.vi"("String"=w1071, "error in"=w1081, "DriverConnect in"=w1078) -> ("error out"=w1076:T15, "DriverConnect out"=w1077:T7)  [unwired: 5 in]
              n328 = call "RS_SMBV100A_Error_check.vi"("Driver Name"=w1079, "Error Code"=w1080, "Error In"=w1076, "DriverConnect in"=w1077) -> ("Error Out"=w1075:errorcluster)  [unwired: 6 in, 1 out]
            }
            frame "---------------------------- TIME_CONVERSION_CONFIGURATION  ----------------------------" {
            }
            frame "TIME_CONVERSION_CONFIGURATION_SIMULATE_LEAP_SECOND_TRANSITION", "TIMECONVERSIONCONFIGURATION_SIMULATELEAPSECONDTRANSITION" {
              # "SOUR:BB:GLON:NAVigation:TCONversion:LEAP:SLST ON"
              n329 = Unbundle By Name(w1089) -> ("BASEBAND"=w1092:string)
              n330 = call "MLLF_ParameterSelect.vi"("Command to equipment"=string[] ["ON\n", "OFF"], "Names"=string[][] [["ON", "1", "ENABLE", "EN"], ["OFF", "0", "DISABLE", "DIS"]], "Input"=w1088, "Command"=w1087, "Driver Name"=w1086, "Error Code"=w1085) -> ("Choice"=w1090:string, "Error Out"=w1099:errorcluster)  [unwired: 8 in]
              n331 = Concatenate Strings("SOUR:BB:", w1092, ":NAVigation:TCONversion:LEAP:SLST ", w1090) -> (w1091:string)
              n332 = call "MLLF_WriteToBuffer.vi"("String"=w1091, "error in"=w1099, "DriverConnect in"=w1096) -> ("error out"=w1097:T15, "DriverConnect out"=w1098:T7)  [unwired: 5 in]
              n333 = call "RS_SMBV100A_Error_check.vi"("Driver Name"=w1086, "Error Code"=w1085, "Error In"=w1097, "DriverConnect in"=w1098) -> ("Error Out"=w1095:errorcluster)  [unwired: 6 in, 1 out]
            }
            frame "TIME_CONVERSION_CONFIGURATION_CURRENT_LEAP_SECONDS", "TIMECONVERSIONCONFIGURATION_CURRENTLEAPSECONDS" {
              n334 = call "MLLF_FormatStringValue.vi"("String Value"=w1102, "Format"=" %.;%1.7f" ("format")) -> ("error out"=w1112:T15, "String Value Formated"=w1113:T16)  [unwired: 7 in, 1 out]
              n335 = Unbundle By Name(w1105) -> ("BASEBAND"=w1104:string)
              n336 = Concatenate Strings("SOUR:BB:", w1104, ":NAVigation:TCONversion:LEAP:SEC " ("string"), w1113) -> (w1107:string)
              n337 = call "MLLF_WriteToBuffer.vi"("String"=w1107, "error in"=w1112, "DriverConnect in"=w1111) -> ("error out"=w1115:T15, "DriverConnect out"=w1116:T7)  [unwired: 5 in]
              n338 = call "RS_SMBV100A_Error_check.vi"("Driver Name"=w1108, "Error Code"=w1109, "Error In"=w1115, "DriverConnect in"=w1116) -> ("Error Out"=w1110:errorcluster)  [unwired: 6 in, 1 out]
            }
            frame "TIME_CONVERSION_CONFIGURATION_SYNCHRONIZE", "TIMECONVERSIONCONFIGURATION_SYNCHRONIZE" {
              n339 = Unbundle By Name(w1117) -> ("BASEBAND"=w1120:string)
              n340 = Concatenate Strings("SOUR:BB:", w1120, ":NAVigation:TCONversion:LEAP:SYNC" ("string")) -> (w1118:string)
              n341 = call "MLLF_WriteToBuffer.vi"("String"=w1118, "DriverConnect in"=w1125) -> ("error out"=w1126:T15, "DriverConnect out"=w1127:T7)  [unwired: 6 in]
              n342 = call "RS_SMBV100A_Error_check.vi"("Driver Name"=w1123, "Error Code"=w1124, "Error In"=w1126, "DriverConnect in"=w1127) -> ("Error Out"=w1122:errorcluster)  [unwired: 6 in, 1 out]
            }
            frame "---------------------------------------  VEHICLE ------------------------------------------" {
            }
            frame "VEHICLE_DESCRIPTION_FILE", "VEHICLEDESCRIPTIONFILE" {
              w1142 = "\"" ("string")
              # "Выбор СВОЙСТВА средства передвижения GLON приемника"
              n343 = Search and Replace String(replace all?=TRUE, input string=w1135, search string="\"", replace string="") -> (result string=w1134:string)  [unwired: 4 in, 3 out]
              n344 = Unbundle By Name(w1129) -> ("BASEBAND"=w1132:string)
              n345 = Concatenate Strings("/hdd/GNSS/vehicle/" ("string"), w1134, ".xvd" ("string")) -> (w1140:string)
              n346 = Concatenate Strings(":VEHicle:FILE " ("string"), w1142, w1140, w1142) -> (w1130:string)
              n347 = Concatenate Strings("SOURce1:BB:", w1132, w1130) -> (w1131:string)
              n348 = call "MLLF_WriteToBuffer.vi"("String"=w1131, "DriverConnect in"=w1147) -> ("error out"=w1145:T15, "DriverConnect out"=w1146:T7)  [unwired: 6 in]
              n349 = call "RS_SMBV100A_Error_check.vi"("Driver Name"=w1148, "Error Code"=w1149, "Error In"=w1145, "DriverConnect in"=w1146) -> ("Error Out"=w1144:errorcluster)  [unwired: 6 in, 1 out]
            }
            frame "VEHICLE_TYPE", "VEHICLETYPE" {
              # "Выбор средства передвижения GLON приемника"
              n350 = Unbundle By Name(w1154) -> ("BASEBAND"=w1157:string)
              n351 = call "MLLF_ParameterSelect.vi"("Command to equipment"=string[] ["PEDESTRIAN", "LAND VEHICLE", "SHIP", "AIRCRAFT", "SPACECRAFT", "HIL"], "Names"=string[][] [["PEDESTRIAN"], ["LAND VEHICLE"], ["SHIP"], ["AIRCRAFT"], ["SPACECRAFT"], ["HIL"]], "Input"=w1151, "Command"=w1150, "Driver Name"=w1152, "Error Code"=w1153) -> ("Choice"=w1155:string, "Error Out"=w1163:errorcluster)  [unwired: 8 in]
              n352 = Concatenate Strings("SOUR:BB:", w1157, ":VEH:TYPE ", w1155) -> (w1156:string)
              n353 = call "MLLF_WriteToBuffer.vi"("String"=w1156, "error in"=w1163, "DriverConnect in"=w1162) -> ("error out"=w1160:T15, "DriverConnect out"=w1161:T7)  [unwired: 5 in]
              n354 = call "RS_SMBV100A_Error_check.vi"("Driver Name"=w1152, "Error Code"=w1153, "Error In"=w1160, "DriverConnect in"=w1161) -> ("Error Out"=w1166:errorcluster)  [unwired: 6 in, 1 out]
            }
            frame "----- LOAD SCENARIO -----" {
              # "Функции настройки в локации GPS"
            }
            frame "GPS_LOAD_SCENARIO" {
              w1187 = "'" ("string")
              # "Осуществляется подгрузка и в прибор и в драйвер сценария."
              # "загружаем сценарий для локации GPS"
              n355 = Search and Replace String(replace all?=TRUE, input string=w1169, search string="\"", replace string="") -> (result string=w1170:string)  [unwired: 4 in, 3 out]
              n356 = Concatenate Strings("GNSS\\scenario\\", w1170) -> (w1178:string)
              n357 = Build Path(base path=w1168, name or relative path=w1178) -> (appended path=w1174:path)
              n358 = Concatenate Strings("/hdd/GNSS/scenario/", w1170) -> (w1175:string)
              n359 = Read from Text File(file (use dialog)=w1174) -> (text=w1191:string, error out=w1182:errorcluster)  [unwired: 3 in, 2 out]
              n360 = Bundle By Name(cluster=w1190, "GPS SCENARIO"=w1191) -> (w1189:T12)
              n361 = Concatenate Strings("SOUR:BB:GPS:LOC:WAYP:FILE " ("string"), w1187, w1175, w1187) -> (w1184:string)
              n362 = call "MLLF_WriteToBuffer.vi"("String"=w1184, "error in"=w1182, "DriverConnect in"=w1183) -> ("error out"=w1185:T15, "DriverConnect out"=w1186:T7)  [unwired: 5 in]
              n363 = call "RS_SMBV100A_Error_check.vi"("Driver Name"=w1179, "Error Code"=w1180, "Error In"=w1185, "DriverConnect in"=w1186) -> ("Error Out"=w1181:errorcluster)  [unwired: 6 in, 1 out]
            }
            frame "GPS_LOAD_WAYPOINTS" {
              # "Импортируем WAYPOINTS в драйвер"
              n364 = Search and Replace String(replace all?=TRUE, input string=w1195, search string="\"", replace string="") -> (result string=w1194:string)  [unwired: 4 in, 3 out]
              n365 = Concatenate Strings("GNSS\\waypoints\\", w1194) -> (w1206:string)
              n366 = Build Path(base path=w1192, name or relative path=w1206) -> (appended path=w1204:path)
              n367 = Read from Text File(file (use dialog)=w1204) -> (text=w1193:string, error out=w1201:errorcluster)  [unwired: 3 in, 2 out]
              n368 = call "RS_SMBV100A_arrayStringToDOUBLE.vi"("string"=w1193, "error in"=w1201) -> ("Dynam waypoints"=w1199:T5, "error out"=w1200:errorcluster)  [unwired: 1 in]
              n369 = Bundle By Name(cluster=w1203, "GPS WAYPOINTS"=w1199, "GPS WAYPOINTS STRING"=w1193) -> (w1202:T12)
            }
            frame "----- Standart Function -----" {
              # "Стандартные функции"
            }
            frame "LEVEL", "RF_LEVEL_AMPLITUDE" {
              # "Уровень выходного сигнала в dBm"
              n370 = call "MLLF_FormatStringValue.vi"("String Value"=w1211, "Format"=" %.;%1.2f" ("format")) -> ("error out"=w1210:T15, "String Value Formated"=w1212:T16)  [unwired: 7 in, 1 out]
              n371 = Concatenate Strings("SOUR:POW:LEV:IMM:AMPL " ("string"), w1212, " dBm" ("string")) -> (w1209:string)
              n372 = call "MLLF_WriteToBuffer.vi"("String"=w1209, "error in"=w1210, "DriverConnect in"=w1218) -> ("error out"=w1216:T15, "DriverConnect out"=w1217:T7)  [unwired: 5 in]
              n373 = call "RS_SMBV100A_Error_check.vi"("Driver Name"=w1219, "Error Code"=w1220, "Error In"=w1216, "DriverConnect in"=w1217) -> ("Error Out"=w1215:errorcluster)  [unwired: 6 in, 1 out]
            }
            frame "SHUTDOWN" {
              # "Сбрасывает прибор в состояние с начальными установками. Синтаксис: PRESET"
              n374 = call "MLLF_WriteToBufferWithDelay.vi"("Command"="SYST:SHUT" ("String"), "DriverConnect in"=w1225) -> ("Error Out"=w1227:errorcluster, "DriverConnect out"=w1228:T7)  [unwired: 8 in]
              n375 = call "RS_SMBV100A_Error_check.vi"("Driver Name"=w1223, "Error Code"=w1224, "Error In"=w1227, "DriverConnect in"=w1228) -> ("Error Out"=w1222:errorcluster)  [unwired: 6 in, 1 out]
            }
            frame "REBOOT" {
              # "Сбрасывает прибор в состояние с начальными установками. Синтаксис: PRESET"
              n376 = call "MLLF_WriteToBufferWithDelay.vi"("Command"="SYST:REB" ("String"), "DriverConnect in"=w1233) -> ("Error Out"=w1235:errorcluster, "DriverConnect out"=w1236:T7)  [unwired: 8 in]
              n377 = call "RS_SMBV100A_Error_check.vi"("Driver Name"=w1231, "Error Code"=w1232, "Error In"=w1235, "DriverConnect in"=w1236) -> ("Error Out"=w1230:errorcluster)  [unwired: 6 in, 1 out]
            }
            frame "RESTART" {
              # "Сбрасывает прибор в состояние с начальными установками. Синтаксис: PRESET"
              n378 = call "MLLF_WriteToBufferWithDelay.vi"("Command"="SYST:REST" ("String"), "DriverConnect in"=w1241) -> ("Error Out"=w1243:errorcluster, "DriverConnect out"=w1244:T7)  [unwired: 8 in]
              n379 = call "RS_SMBV100A_Error_check.vi"("Driver Name"=w1239, "Error Code"=w1240, "Error In"=w1243, "DriverConnect in"=w1244) -> ("Error Out"=w1238:errorcluster)  [unwired: 6 in, 1 out]
            }
            frame "RF_LEVEL_LIMIT" {
              # "Уровень LIMITA PEP выходного сигнала в dBm"
              n380 = call "MLLF_FormatStringValue.vi"("String Value"=w1249, "Format"=" %.;%1.2f" ("format")) -> ("error out"=w1248:T15, "String Value Formated"=w1250:T16)  [unwired: 7 in, 1 out]
              n381 = Concatenate Strings("SOUR:POW:LIM:AMPL " ("string"), w1250, " dBm" ("string")) -> (w1247:string)
              n382 = call "MLLF_WriteToBuffer.vi"("String"=w1247, "error in"=w1248, "DriverConnect in"=w1256) -> ("error out"=w1254:T15, "DriverConnect out"=w1255:T7)  [unwired: 5 in]
              n383 = call "RS_SMBV100A_Error_check.vi"("Driver Name"=w1257, "Error Code"=w1258, "Error In"=w1254, "DriverConnect in"=w1255) -> ("Error Out"=w1253:errorcluster)  [unwired: 6 in, 1 out]
            }
          }
        }
        frame "get" {
          # "Тут реализованы функции DriverGet"
          n384 = Unbundle By Name(w1275) -> ("Data.Connect"=w1269:T7)
          n385 = call "MLLF_CommandDelimeter.vi"("command with param"=w1276) -> ("param 1"=w1261:string, "command"=w1262:string, "Spit delimetre"=w1260:string)  [unwired: 6 in, 2 out]
          n386 = case shown="\"EPHEMERISPARAMETERS_TOE\"" w1262 {
            selector: w1262 -> [w1278 _ _ _ _ _ _ _ _ _ _ _ _ _ _ _ _ _ _ _ _ _ _ _ _ _ _ _ _ _ _ _ _ _ _ _ _ _ _ _ _ _ _ _ _ _ _ _ _ _ _ _ _ _ _ _ _ _ _ _ _ _ _ _ _ _]
            tunnel: [w1277 _ w1284 _ _ _ w1303 w1317 w1331 _ _ _ w1352 w1368 w1384 w1399 w1415 w1431 w1447 w1463 w1479 w1495 w1511 w1527 w1543 w1559 w1575 w1591 w1607 w1623 w1639 w1655 w1671 _ w1703 w1721 w1745 w1757 w1770 w1810 w1846 w1870 w1882 w1913 _ w1925 w1936 w1947 w1958 w1969 w1980 w1991 w2002 w2013 w2024 w2035 w2046 w2057 w2068 w2079 w2090 w2101 w2112 w2118 w2135 w2146] -> w1268
            tunnel: w1273 -> [_ _ _ _ _ _ _ _ _ _ _ _ w1354 w1370 w1386 w1401 w1417 w1433 w1449 w1465 w1481 w1497 w1513 w1529 w1545 w1561 w1577 w1593 w1609 w1625 w1641 w1657 w1673 _ w1705 w1723 w1747 w1759 w1769 w1809 w1845 w1869 w1881 w1915 _ w1927 w1938 w1949 w1960 w1971 w1982 w1993 w2004 w2015 w2026 w2037 w2048 w2059 w2070 w2081 w2092 w2103 w2114 w2126 w2137 w2148]
            tunnel: [w1281 w1282 w1283 w1290 w1291 w1292 w1302 w1316 w1330 w1339 w1340 w1341 w1343 w1359 w1375 w1392 w1407 w1423 w1439 w1455 w1472 w1487 w1503 w1520 w1536 w1552 w1568 w1584 w1599 w1615 w1631 w1647 w1663 w1678 w1679 w1706 w1741 w1749 w1762 w1793 w1833 w1850 w1874 w1905 w1916 w1918 w1930 w1941 w1952 w1962 w1973 w1984 w1995 w2006 w2017 w2028 w2039 w2050 w2061 w2072 w2083 w2094 w2105 w2116 w2128 w2139] -> w1274
            tunnel: w1275 -> [w1281 w1282 w1283 w1290 w1291 w1292 w1302 w1316 w1330 w1339 w1340 w1341 w1343 w1359 w1375 w1392 w1407 w1423 w1439 w1455 w1472 w1487 w1503 w1520 w1536 w1552 w1568 w1584 w1599 w1615 w1631 w1647 w1663 w1678 w1679 w1706 w1741 w1749 w1762 w1793 w1833 w1850 w1874 w1905 w1916 w1918 w1930 w1941 w1952 w1962 w1973 w1984 w1995 w2006 w2017 w2028 w2039 w2050 w2061 w2072 w2083 w2094 w2105 w2116 w2128 w2139]
            tunnel: [w1279 _ _ w1288 _ _ _ _ _ _ _ _ w1351 w1367 w1383 w1393 w1410 w1425 w1441 w1457 w1474 w1490 w1507 w1521 w1538 w1554 w1570 w1586 w1601 w1617 w1634 w1649 w1665 _ w1702 _ _ _ _ _ w1841 w1865 _ w1912 _ w1924 w1935 w1946 w1954 w1965 w1976 w1986 w1998 w2009 w2020 w2031 w2042 w2052 w2064 w2075 w2086 w2097 w2108 _ w2131 w2142] -> w1270
            tunnel: w1269 -> [_ _ w1287 _ _ _ w1304 w1318 w1332 _ _ _ w1350 w1366 w1382 w1398 w1414 w1430 w1446 w1462 w1478 w1494 w1510 w1526 w1542 w1558 w1574 w1590 w1606 w1622 w1638 w1654 w1670 _ w1701 w1719 w1731 w1753 w1766 w1801 w1838 w1860 w1878 w1911 _ w1923 w1934 w1945 w1957 w1968 w1979 w1990 w2001 w2012 w2023 w2034 w2045 w2056 w2067 w2078 w2089 w2100 w2111 w2124 w2134 w2145]
            tunnel: w1272 -> [_ _ _ _ _ _ _ _ _ _ _ _ w1353 w1369 w1385 w1400 w1416 w1432 w1448 w1464 w1480 w1496 w1512 w1528 w1544 w1560 w1576 w1592 w1608 w1624 w1640 w1656 w1672 _ w1704 w1722 w1746 w1758 w1768 w1808 w1844 w1868 w1880 w1914 _ w1926 w1937 w1948 w1959 w1970 w1981 w1992 w2003 w2014 w2025 w2036 w2047 w2058 w2069 w2080 w2091 w2102 w2113 w2125 w2136 w2147]
            tunnel: [_ _ w1285 _ _ _ w1295 w1312 w1327 _ _ _ _ _ _ _ _ _ _ _ _ _ _ _ _ _ _ _ _ _ _ _ _ _ _ w1715 w1734 w1754 w1788 w1828 _ _ w1900 _ _ _ _ _ _ _ _ _ _ _ _ _ _ _ _ _ _ _ _ w2122 _ _] -> w1265
            tunnel: w1261 -> [_ _ _ _ _ _ _ _ _ _ _ _ w1347 w1363 w1379 w1395 w1411 w1427 w1443 w1459 w1475 w1491 w1506 w1523 w1539 w1555 w1571 w1587 w1603 w1619 w1635 w1651 w1667 _ w1700 _ _ _ w1765 w1797 w1837 w1862 w1877 w1910 _ _ _ _ _ _ _ _ _ _ _ _ _ _ _ _ _ _ _ _ _ _]
            tunnel: w1260 -> [_ _ w1286 _ _ _ _ _ _ _ _ _ _ _ _ _ _ _ _ _ _ _ _ _ _ _ _ _ _ _ _ _ _ _ _ _ _ _ _ _ _ _ _ _ _ _ _ _ _ _ _ _ _ _ _ _ _ _ _ _ _ _ _ _ _ _]
            frame "False", Default {
              # "DEFAULT"
              n387 = call "MLLF_UnknownCommand(SubVI).vi"("Unknown command"=w1278) -> ("error out"=w1277:errorcluster)  [unwired: 10 in]
              n388 = Build Array(0 ("TimeOut")) -> (w1279:i32[])
            }
            frame "______________ Standart ________________" {
            }
            frame "#", "SCPI" {
              n389 = call "RS_SMBV100A_FASTQUERY.vi"("input"=w1286, "DriverConnect in"=w1287) -> ("Error Out"=w1284:errorcluster, "output"=w1285:string)  [unwired: 7 in, 1 out]
            }
            frame "TIMEOUT" {
              # "Время ожидания ответа от прибора."
              n390 = Unbundle By Name(w1290) -> ("Data.Connect.InterfaceSettings.TMO, ms"=w1289:i32)
              n391 = Build Array(w1289) -> (w1288:i32[])
            }
            frame "________________________________________" {
            }
            frame "------ID-------" {
            }
            frame "model" {
              n392 = call "RS_SMBV100A_FASTQUERY.vi"("input"="*IDN?", "DriverConnect in"=w1304) -> ("Error Out"=w1303:errorcluster, "output"=w1301:string)  [unwired: 7 in, 1 out]
              n393 = for {
                N: 4 -> [_]
                shift-right: [w1306] -> _
                shift-left: w1301 -> [w1309]
                tunnel: [w1308] -> w1300 mode=indexing
                stop <- w1307 stop-if-true
                n394 = Match Pattern(string=w1309, regular expression=",") -> (before substring=w1308:string, after substring=w1306:string)  [unwired: 1 in, 2 out]
                n395 = Empty String/Path?(string/path=w1306) -> (empty?=w1307:bool)
              }
              n396 = Index Array(array=w1300, index #1=0 ("index"), index #2=1 ("index")) -> (element #1=w1298:string, element #2=w1296:string)
              n397 = Concatenate Strings(w1298, " " ("string"), w1296) -> (w1295:string)
            }
            frame "FW", "ver", "version" {
              n398 = call "RS_SMBV100A_FASTQUERY.vi"("input"="*IDN?", "DriverConnect in"=w1318) -> ("Error Out"=w1317:errorcluster, "output"=w1313:string)  [unwired: 7 in, 1 out]
              n399 = for {
                N: 4 -> [_]
                shift-right: [w1320] -> _
                shift-left: w1313 -> [w1323]
                tunnel: [w1322] -> w1315 mode=indexing
                stop <- w1321 stop-if-true
                n400 = Match Pattern(string=w1323, regular expression=",") -> (before substring=w1322:string, after substring=w1320:string)  [unwired: 1 in, 2 out]
                n401 = Empty String/Path?(string/path=w1320) -> (empty?=w1321:bool)
              }
              n402 = Index Array(array=w1315, index=3) -> (element=w1312:string)
            }
            frame "serial", "serialNum", "SN" {
              n403 = call "RS_SMBV100A_FASTQUERY.vi"("input"="*IDN?", "DriverConnect in"=w1332) -> ("Error Out"=w1331:errorcluster, "output"=w1326:string)  [unwired: 7 in, 1 out]
              n404 = for {
                N: 4 -> [_]
                shift-right: [w1334] -> _
                shift-left: w1326 -> [w1337]
                tunnel: [w1336] -> w1329 mode=indexing
                stop <- w1335 stop-if-true
                n405 = Match Pattern(string=w1337, regular expression=",") -> (before substring=w1336:string, after substring=w1334:string)  [unwired: 1 in, 2 out]
                n406 = Empty String/Path?(string/path=w1334) -> (empty?=w1335:bool)
              }
              n407 = Index Array(array=w1329, index=2) -> (element=w1327:string)
            }
            frame "----- BASEBAND -----" {
            }
            frame "----- GPS BASEBAND -----" {
            }
            frame "----- GPS BASEBAND MASS WITH SARTIROVKA-----" {
            }
            frame "GNNS_N_NUMBER_ACTIVE_SAT" {
              # "колличество активных спутников на Созвездии."
              n408 = Unbundle By Name(w1343) -> ("BASEBAND"=w1344:string)
              n409 = call "RS_SMBV100A_N_ASKCONFIGURATION.vi"("DriverConnect in"=w1350, "BASEBAND"=w1344, "mass"=w1347) -> ("wrong sat"=w1345:bool, "DriverConnect out"=w1349:T7, "Parsing Satelite"=w1342:T18, "Error Out"=w1348:errorcluster)  [unwired: 9 in]
              n410 = case shown="False" w1345 {
                tunnel: [0.0 ("OUT GNSS NUMBERACTIVESAT") w1357] -> w1346
                tunnel: w1342 -> [_ w1356]
                frame True {
                  # "Если Тру вернуть Ноль\nтогда в скрипте проверку делать"
                }
                frame False {
                  n411 = call "RS_SMBV100A_PARS_SAT_TIME_AND_NUMBER.vi"("Parsing Satelite"=w1356) -> ("OUT GNSS NUMBERACTIVESAT"=w1357:dbl)  [unwired: 13 in, 5 out]
                }
              }
              n412 = Build Array(w1346) -> (w1351:dbl[])
              n413 = call "RS_SMBV100A_Error_check.vi"("Driver Name"=w1353, "Error Code"=w1354, "Error In"=w1348, "DriverConnect in"=w1349) -> ("Error Out"=w1352:errorcluster)  [unwired: 6 in, 1 out]
            }
            frame "GPS_N_NUMBER_ACTIVE_SAT" {
              # "колличество активных спутников GPS на Созвездии."
              n414 = Unbundle By Name(w1359) -> ("BASEBAND"=w1360:string)
              n415 = call "RS_SMBV100A_N_ASKCONFIGURATION.vi"("DriverConnect in"=w1366, "BASEBAND"=w1360, "mass"=w1363) -> ("wrong sat"=w1361:bool, "DriverConnect out"=w1365:T7, "Parsing Satelite"=w1358:T18, "Error Out"=w1364:errorcluster)  [unwired: 9 in]
              n416 = case shown="False" w1361 {
                tunnel: [0.0 ("OUT GNSS NUMBERACTIVESAT") w1373] -> w1362
                tunnel: w1358 -> [_ w1372]
                frame True {
                  # "Если Тру вернуть Ноль\nтогда в скрипте проверку делать"
                }
                frame False {
                  n417 = call "RS_SMBV100A_PARS_SAT_TIME_AND_NUMBER.vi"("Parsing Satelite"=w1372) -> ("OUT GPS NUMBERACTIVESAT"=w1373:dbl)  [unwired: 13 in, 5 out]
                }
              }
              n418 = Build Array(w1362) -> (w1367:dbl[])
              n419 = call "RS_SMBV100A_Error_check.vi"("Driver Name"=w1369, "Error Code"=w1370, "Error In"=w1364, "DriverConnect in"=w1365) -> ("Error Out"=w1368:errorcluster)  [unwired: 6 in, 1 out]
            }
            frame "GLONASS_N_NUMBER_ACTIVE_SAT" {
              # "колличество активных спутников GLONASS на Созвездии."
              n420 = Unbundle By Name(w1375) -> ("BASEBAND"=w1376:string)
              n421 = call "RS_SMBV100A_N_ASKCONFIGURATION.vi"("DriverConnect in"=w1382, "BASEBAND"=w1376, "mass"=w1379) -> ("wrong sat"=w1378:bool, "DriverConnect out"=w1381:T7, "Parsing Satelite"=w1374:T18, "Error Out"=w1380:errorcluster)  [unwired: 9 in]
              n422 = case shown="False" w1378 {
                tunnel: [0.0 ("OUT GNSS NUMBERACTIVESAT") w1389] -> w1377
                tunnel: w1374 -> [_ w1388]
                frame True {
                  # "Если Тру вернуть Ноль\nтогда в скрипте проверку делать"
                }
                frame False {
                  n423 = call "RS_SMBV100A_PARS_SAT_TIME_AND_NUMBER.vi"("Parsing Satelite"=w1388) -> ("OUT GLONASS NUMBERACTIVESAT"=w1389:dbl)  [unwired: 13 in, 5 out]
                }
              }
              n424 = Build Array(w1377) -> (w1383:dbl[])
              n425 = call "RS_SMBV100A_Error_check.vi"("Driver Name"=w1385, "Error Code"=w1386, "Error In"=w1380, "DriverConnect in"=w1381) -> ("Error Out"=w1384:errorcluster)  [unwired: 6 in, 1 out]
            }
            frame "GNSS_N_SAT_SORTED_MINTOMAX" {
              # "Массив порядка спутников(не номеров собственных) по времени от наименьшего времени"
              n426 = Unbundle By Name(w1392) -> ("BASEBAND"=w1391:string)
              n427 = call "RS_SMBV100A_N_ASKCONFIGURATION.vi"("DriverConnect in"=w1398, "BASEBAND"=w1391, "mass"=w1395) -> ("wrong sat"=w1394:bool, "DriverConnect out"=w1397:T7, "Parsing Satelite"=w1390:T18, "Error Out"=w1396:errorcluster)  [unwired: 9 in]
              n428 = case shown="False" w1394 {
                tunnel: [dbl[] [0.0] ("GNSS_SatSkySortedMinToMax") w1405] -> w1393
                tunnel: w1390 -> [_ w1403]
                frame True {
                  # "Если Тру вернуть Ноль\nтогда в скрипте проверку делать"
                }
                frame False {
                  n429 = call "RS_SMBV100A_PARS_SAT_TIME_AND_NUMBER.vi"("Parsing Satelite"=w1403) -> ("GNSS 2D SAT"=w1404:dbl[][])  [unwired: 13 in, 5 out]
                  n430 = call "RS_SMBV100A_CONVERT_DATASAT_2D_to_N1D.vi"("2D DATA SAT"=w1404) -> ("GNSS_SatSortedMinToMax"=w1405:dbl[])  [unwired: 2 in, 5 out]
                }
              }
              n431 = call "RS_SMBV100A_Error_check.vi"("Driver Name"=w1400, "Error Code"=w1401, "Error In"=w1396, "DriverConnect in"=w1397) -> ("Error Out"=w1399:errorcluster)  [unwired: 6 in, 1 out]
            }
            frame "GPS_N_SAT_SORTED_MINTOMAX" {
              # "Массив порядка GPS спутников(не номеров собственных) по времени от наименьшего времени"
              n432 = Unbundle By Name(w1407) -> ("BASEBAND"=w1408:string)
              n433 = call "RS_SMBV100A_N_ASKCONFIGURATION.vi"("DriverConnect in"=w1414, "BASEBAND"=w1408, "mass"=w1411) -> ("wrong sat"=w1409:bool, "DriverConnect out"=w1413:T7, "Parsing Satelite"=w1406:T18, "Error Out"=w1412:errorcluster)  [unwired: 9 in]
              n434 = case shown="False" w1409 {
                tunnel: [dbl[] [0.0] ("GNSS_SatSkySortedMinToMax") w1420] -> w1410
                tunnel: w1406 -> [_ w1419]
                frame True {
                  # "Если Тру вернуть Ноль\nтогда в скрипте проверку делать"
                }
                frame False {
                  n435 = call "RS_SMBV100A_PARS_SAT_TIME_AND_NUMBER.vi"("Parsing Satelite"=w1419) -> ("GPS 2D SAT"=w1421:dbl[][])  [unwired: 13 in, 5 out]
                  n436 = call "RS_SMBV100A_CONVERT_DATASAT_2D_to_N1D.vi"("2D DATA SAT"=w1421) -> ("GNSS_SatSortedMinToMax"=w1420:dbl[])  [unwired: 2 in, 5 out]
                }
              }
              n437 = call "RS_SMBV100A_Error_check.vi"("Driver Name"=w1416, "Error Code"=w1417, "Error In"=w1412, "DriverConnect in"=w1413) -> ("Error Out"=w1415:errorcluster)  [unwired: 6 in, 1 out]
            }
            frame "GLONASS_N_SAT_SORTED_MINTOMAX" {
              # "Массив порядка GLONASS спутников(не номеров собственных) по времени от наименьшего времени"
              n438 = Unbundle By Name(w1423) -> ("BASEBAND"=w1424:string)
              n439 = call "RS_SMBV100A_N_ASKCONFIGURATION.vi"("DriverConnect in"=w1430, "BASEBAND"=w1424, "mass"=w1427) -> ("wrong sat"=w1426:bool, "DriverConnect out"=w1429:T7, "Parsing Satelite"=w1422:T18, "Error Out"=w1428:errorcluster)  [unwired: 9 in]
              n440 = case shown="False" w1426 {
                tunnel: [dbl[] [0.0] ("GNSS_SatSkySortedMinToMax") w1437] -> w1425
                tunnel: w1422 -> [_ w1435]
                frame True {
                  # "Если Тру вернуть Ноль\nтогда в скрипте проверку делать"
                }
                frame False {
                  n441 = call "RS_SMBV100A_PARS_SAT_TIME_AND_NUMBER.vi"("Parsing Satelite"=w1435) -> ("GLONASS 2D SAT"=w1436:dbl[][])  [unwired: 13 in, 5 out]
                  n442 = call "RS_SMBV100A_CONVERT_DATASAT_2D_to_N1D.vi"("2D DATA SAT"=w1436) -> ("GNSS_SatSortedMinToMax"=w1437:dbl[])  [unwired: 2 in, 5 out]
                }
              }
              n443 = call "RS_SMBV100A_Error_check.vi"("Driver Name"=w1432, "Error Code"=w1433, "Error In"=w1428, "DriverConnect in"=w1429) -> ("Error Out"=w1431:errorcluster)  [unwired: 6 in, 1 out]
            }
            frame "GNSS_N_TIME_SORTED_MINTOMAX" {
              # "Массив времен в секундах GNSS спутников - от наименьшего времени"
              n444 = Unbundle By Name(w1439) -> ("BASEBAND"=w1440:string)
              n445 = call "RS_SMBV100A_N_ASKCONFIGURATION.vi"("DriverConnect in"=w1446, "BASEBAND"=w1440, "mass"=w1443) -> ("wrong sat"=w1442:bool, "DriverConnect out"=w1445:T7, "Parsing Satelite"=w1438:T18, "Error Out"=w1444:errorcluster)  [unwired: 9 in]
              n446 = case shown="False" w1442 {
                tunnel: [dbl[] [0.0] ("GNSS_SatSkySortedMinToMax") w1452] -> w1441
                tunnel: w1438 -> [_ w1451]
                frame True {
                  # "Если Тру вернуть Ноль\nтогда в скрипте проверку делать"
                }
                frame False {
                  n447 = call "RS_SMBV100A_PARS_SAT_TIME_AND_NUMBER.vi"("Parsing Satelite"=w1451) -> ("GNSS 2D SAT"=w1453:dbl[][])  [unwired: 13 in, 5 out]
                  n448 = call "RS_SMBV100A_CONVERT_DATASAT_2D_to_N1D.vi"("2D DATA SAT"=w1453) -> ("GNSS_TimeSortedMinToMax"=w1452:dbl[])  [unwired: 2 in, 5 out]
                }
              }
              n449 = call "RS_SMBV100A_Error_check.vi"("Driver Name"=w1448, "Error Code"=w1449, "Error In"=w1444, "DriverConnect in"=w1445) -> ("Error Out"=w1447:errorcluster)  [unwired: 6 in, 1 out]
            }
            frame "GPS_N_TIME_SORTED_MINTOMAX" {
              # "Массив времен в секундах GPS спутников - от наименьшего времени"
              n450 = Unbundle By Name(w1455) -> ("BASEBAND"=w1456:string)
              n451 = call "RS_SMBV100A_N_ASKCONFIGURATION.vi"("DriverConnect in"=w1462, "BASEBAND"=w1456, "mass"=w1459) -> ("wrong sat"=w1458:bool, "DriverConnect out"=w1461:T7, "Parsing Satelite"=w1454:T18, "Error Out"=w1460:errorcluster)  [unwired: 9 in]
              n452 = case shown="False" w1458 {
                tunnel: [dbl[] [0.0] ("GNSS_SatSkySortedMinToMax") w1468] -> w1457
                tunnel: w1454 -> [_ w1467]
                frame True {
                  # "Если Тру вернуть Ноль\nтогда в скрипте проверку делать"
                }
                frame False {
                  n453 = call "RS_SMBV100A_PARS_SAT_TIME_AND_NUMBER.vi"("Parsing Satelite"=w1467) -> ("GPS 2D SAT"=w1469:dbl[][])  [unwired: 13 in, 5 out]
                  n454 = call "RS_SMBV100A_CONVERT_DATASAT_2D_to_N1D.vi"("2D DATA SAT"=w1469) -> ("GNSS_TimeSortedMinToMax"=w1468:dbl[])  [unwired: 2 in, 5 out]
                }
              }
              n455 = call "RS_SMBV100A_Error_check.vi"("Driver Name"=w1464, "Error Code"=w1465, "Error In"=w1460, "DriverConnect in"=w1461) -> ("Error Out"=w1463:errorcluster)  [unwired: 6 in, 1 out]
            }
            frame "GLONASS_N_TIME_SORTED_MINTOMAX" {
              # "Массив времен в секундах GLONASS спутников - от наименьшего времени"
              n456 = Unbundle By Name(w1472) -> ("BASEBAND"=w1471:string)
              n457 = call "RS_SMBV100A_N_ASKCONFIGURATION.vi"("DriverConnect in"=w1478, "BASEBAND"=w1471, "mass"=w1475) -> ("wrong sat"=w1473:bool, "DriverConnect out"=w1477:T7, "Parsing Satelite"=w1470:T18, "Error Out"=w1476:errorcluster)  [unwired: 9 in]
              n458 = case shown="False" w1473 {
                tunnel: [dbl[] [0.0] ("GNSS_SatSkySortedMinToMax") w1484] -> w1474
                tunnel: w1470 -> [_ w1483]
                frame True {
                  # "Если Тру вернуть Ноль\nтогда в скрипте проверку делать"
                }
                frame False {
                  n459 = call "RS_SMBV100A_PARS_SAT_TIME_AND_NUMBER.vi"("Parsing Satelite"=w1483) -> ("GLONASS 2D SAT"=w1485:dbl[][])  [unwired: 13 in, 5 out]
                  n460 = call "RS_SMBV100A_CONVERT_DATASAT_2D_to_N1D.vi"("2D DATA SAT"=w1485) -> ("GNSS_TimeSortedMinToMax"=w1484:dbl[])  [unwired: 2 in, 5 out]
                }
              }
              n461 = call "RS_SMBV100A_Error_check.vi"("Driver Name"=w1480, "Error Code"=w1481, "Error In"=w1476, "DriverConnect in"=w1477) -> ("Error Out"=w1479:errorcluster)  [unwired: 6 in, 1 out]
            }
            frame "GNSS_N_SKY_SORTED_MINTOMAX" {
              # "Массив номеров GNSS спутников на небе - от наименьшего времени"
              n462 = Unbundle By Name(w1487) -> ("BASEBAND"=w1488:string)
              n463 = call "RS_SMBV100A_N_ASKCONFIGURATION.vi"("DriverConnect in"=w1494, "BASEBAND"=w1488, "mass"=w1491) -> ("wrong sat"=w1489:bool, "DriverConnect out"=w1493:T7, "Parsing Satelite"=w1486:T18, "Error Out"=w1492:errorcluster)  [unwired: 9 in]
              n464 = case shown="False" w1489 {
                tunnel: [dbl[] [0.0] ("GNSS_SatSkySortedMinToMax") w1501] -> w1490
                tunnel: w1486 -> [_ w1499]
                frame True {
                  # "Если Тру вернуть Ноль\nтогда в скрипте проверку делать"
                }
                frame False {
                  n465 = call "RS_SMBV100A_PARS_SAT_TIME_AND_NUMBER.vi"("Parsing Satelite"=w1499) -> ("GNSS 2D SAT"=w1500:dbl[][])  [unwired: 13 in, 5 out]
                  n466 = call "RS_SMBV100A_CONVERT_DATASAT_2D_to_N1D.vi"("2D DATA SAT"=w1500) -> ("GNSS_SatSkySortedMinToMax"=w1501:dbl[])  [unwired: 2 in, 5 out]
                }
              }
              n467 = call "RS_SMBV100A_Error_check.vi"("Driver Name"=w1496, "Error Code"=w1497, "Error In"=w1492, "DriverConnect in"=w1493) -> ("Error Out"=w1495:errorcluster)  [unwired: 6 in, 1 out]
            }
            frame "GPS_N_SKY_SORTED_MINTOMAX" {
              # "Массив номеров GPS спутников на небе - от наименьшего времени"
              n468 = Unbundle By Name(w1503) -> ("BASEBAND"=w1504:string)
              n469 = call "RS_SMBV100A_N_ASKCONFIGURATION.vi"("DriverConnect in"=w1510, "BASEBAND"=w1504, "mass"=w1506) -> ("wrong sat"=w1505:bool, "DriverConnect out"=w1509:T7, "Parsing Satelite"=w1502:T18, "Error Out"=w1508:errorcluster)  [unwired: 9 in]
              n470 = case shown="False" w1505 {
                tunnel: [dbl[] [0.0] ("GNSS_SatSkySortedMinToMax") w1517] -> w1507
                tunnel: w1502 -> [_ w1515]
                frame True {
                  # "Если Тру вернуть Ноль\nтогда в скрипте проверку делать"
                }
                frame False {
                  n471 = call "RS_SMBV100A_PARS_SAT_TIME_AND_NUMBER.vi"("Parsing Satelite"=w1515) -> ("GPS 2D SAT"=w1516:dbl[][])  [unwired: 13 in, 5 out]
                  n472 = call "RS_SMBV100A_CONVERT_DATASAT_2D_to_N1D.vi"("2D DATA SAT"=w1516) -> ("GNSS_SatSkySortedMinToMax"=w1517:dbl[])  [unwired: 2 in, 5 out]
                }
              }
              n473 = call "RS_SMBV100A_Error_check.vi"("Driver Name"=w1512, "Error Code"=w1513, "Error In"=w1508, "DriverConnect in"=w1509) -> ("Error Out"=w1511:errorcluster)  [unwired: 6 in, 1 out]
            }
            frame "GLONASS_N_SKY_SORTED_MINTOMAX" {
              # "Массив номеров GLONASS спутников на небе - от наименьшего времени"
              n474 = Unbundle By Name(w1520) -> ("BASEBAND"=w1519:string)
              n475 = call "RS_SMBV100A_N_ASKCONFIGURATION.vi"("DriverConnect in"=w1526, "BASEBAND"=w1519, "mass"=w1523) -> ("wrong sat"=w1522:bool, "DriverConnect out"=w1525:T7, "Parsing Satelite"=w1518:T18, "Error Out"=w1524:errorcluster)  [unwired: 9 in]
              n476 = case shown="False" w1522 {
                tunnel: [dbl[] [0.0] ("GNSS_SatSkySortedMinToMax") w1532] -> w1521
                tunnel: w1518 -> [_ w1531]
                frame True {
                  # "Если Тру вернуть Ноль\nтогда в скрипте проверку делать"
                }
                frame False {
                  n477 = call "RS_SMBV100A_PARS_SAT_TIME_AND_NUMBER.vi"("Parsing Satelite"=w1531) -> ("GLONASS 2D SAT"=w1533:dbl[][])  [unwired: 13 in, 5 out]
                  n478 = call "RS_SMBV100A_CONVERT_DATASAT_2D_to_N1D.vi"("2D DATA SAT"=w1533) -> ("GNSS_SatSkySortedMinToMax"=w1532:dbl[])  [unwired: 2 in, 5 out]
                }
              }
              n479 = call "RS_SMBV100A_Error_check.vi"("Driver Name"=w1528, "Error Code"=w1529, "Error In"=w1524, "DriverConnect in"=w1525) -> ("Error Out"=w1527:errorcluster)  [unwired: 6 in, 1 out]
            }
            frame "GNSS_N_SAT_SORTED_MAXTOMIN" {
              # "Массив порядка спутников(не номеров собственных) по времени от наибольшего времени"
              n480 = Unbundle By Name(w1536) -> ("BASEBAND"=w1535:string)
              n481 = call "RS_SMBV100A_N_ASKCONFIGURATION.vi"("DriverConnect in"=w1542, "BASEBAND"=w1535, "mass"=w1539) -> ("wrong sat"=w1537:bool, "DriverConnect out"=w1541:T7, "Parsing Satelite"=w1534:T18, "Error Out"=w1540:errorcluster)  [unwired: 9 in]
              n482 = case shown="False" w1537 {
                tunnel: [dbl[] [0.0] ("GNSS_SatSkySortedMinToMax") w1549] -> w1538
                tunnel: w1534 -> [_ w1547]
                frame True {
                  # "Если Тру вернуть Ноль\nтогда в скрипте проверку делать"
                }
                frame False {
                  n483 = call "RS_SMBV100A_PARS_SAT_TIME_AND_NUMBER.vi"("Parsing Satelite"=w1547) -> ("GNSS 2D SAT"=w1548:dbl[][])  [unwired: 13 in, 5 out]
                  n484 = call "RS_SMBV100A_CONVERT_DATASAT_2D_to_N1D.vi"("2D DATA SAT"=w1548) -> ("GNSS_SatSortedMaxToMin"=w1549:dbl[])  [unwired: 2 in, 5 out]
                }
              }
              n485 = call "RS_SMBV100A_Error_check.vi"("Driver Name"=w1544, "Error Code"=w1545, "Error In"=w1540, "DriverConnect in"=w1541) -> ("Error Out"=w1543:errorcluster)  [unwired: 6 in, 1 out]
            }
            frame "GPS_N_SAT_SORTED_MAXTOMIN" {
              # "Массив порядка GPS спутников(не номеров собственных) по времени от наибольшего времени"
              n486 = Unbundle By Name(w1552) -> ("BASEBAND"=w1551:string)
              n487 = call "RS_SMBV100A_N_ASKCONFIGURATION.vi"("DriverConnect in"=w1558, "BASEBAND"=w1551, "mass"=w1555) -> ("wrong sat"=w1553:bool, "DriverConnect out"=w1557:T7, "Parsing Satelite"=w1550:T18, "Error Out"=w1556:errorcluster)  [unwired: 9 in]
              n488 = case shown="False" w1553 {
                tunnel: [dbl[] [0.0] ("GNSS_SatSkySortedMinToMax") w1564] -> w1554
                tunnel: w1550 -> [_ w1563]
                frame True {
                  # "Если Тру вернуть Ноль\nтогда в скрипте проверку делать"
                }
                frame False {
                  n489 = call "RS_SMBV100A_PARS_SAT_TIME_AND_NUMBER.vi"("Parsing Satelite"=w1563) -> ("GPS 2D SAT"=w1565:dbl[][])  [unwired: 13 in, 5 out]
                  n490 = call "RS_SMBV100A_CONVERT_DATASAT_2D_to_N1D.vi"("2D DATA SAT"=w1565) -> ("GNSS_SatSortedMaxToMin"=w1564:dbl[])  [unwired: 2 in, 5 out]
                }
              }
              n491 = call "RS_SMBV100A_Error_check.vi"("Driver Name"=w1560, "Error Code"=w1561, "Error In"=w1556, "DriverConnect in"=w1557) -> ("Error Out"=w1559:errorcluster)  [unwired: 6 in, 1 out]
            }
            frame "GLONASS_N_SAT_SORTED_MAXTOMIN" {
              # "Массив порядка GLONASS спутников(не номеров собственных) по времени от наибольшего времени"
              n492 = Unbundle By Name(w1568) -> ("BASEBAND"=w1567:string)
              n493 = call "RS_SMBV100A_N_ASKCONFIGURATION.vi"("DriverConnect in"=w1574, "BASEBAND"=w1567, "mass"=w1571) -> ("wrong sat"=w1569:bool, "DriverConnect out"=w1573:T7, "Parsing Satelite"=w1566:T18, "Error Out"=w1572:errorcluster)  [unwired: 9 in]
              n494 = case shown="False" w1569 {
                tunnel: [dbl[] [0.0] ("GNSS_SatSkySortedMinToMax") w1581] -> w1570
                tunnel: w1566 -> [_ w1579]
                frame True {
                  # "Если Тру вернуть Ноль\nтогда в скрипте проверку делать"
                }
                frame False {
                  n495 = call "RS_SMBV100A_PARS_SAT_TIME_AND_NUMBER.vi"("Parsing Satelite"=w1579) -> ("GLONASS 2D SAT"=w1580:dbl[][])  [unwired: 13 in, 5 out]
                  n496 = call "RS_SMBV100A_CONVERT_DATASAT_2D_to_N1D.vi"("2D DATA SAT"=w1580) -> ("GNSS_SatSortedMaxToMin"=w1581:dbl[])  [unwired: 2 in, 5 out]
                }
              }
              n497 = call "RS_SMBV100A_Error_check.vi"("Driver Name"=w1576, "Error Code"=w1577, "Error In"=w1572, "DriverConnect in"=w1573) -> ("Error Out"=w1575:errorcluster)  [unwired: 6 in, 1 out]
            }
            frame "GPS_N_TIME_SORTED_MAXTOMIN" {
              # "Массив времен в секундах GPS спутников- по времени от наибольшего времени"
              n498 = Unbundle By Name(w1584) -> ("BASEBAND"=w1583:string)
              n499 = call "RS_SMBV100A_N_ASKCONFIGURATION.vi"("DriverConnect in"=w1590, "BASEBAND"=w1583, "mass"=w1587) -> ("wrong sat"=w1585:bool, "DriverConnect out"=w1589:T7, "Parsing Satelite"=w1582:T18, "Error Out"=w1588:errorcluster)  [unwired: 9 in]
              n500 = case shown="False" w1585 {
                tunnel: [dbl[] [0.0] ("GNSS_SatSkySortedMinToMax") w1596] -> w1586
                tunnel: w1582 -> [_ w1595]
                frame True {
                  # "Если Тру вернуть Ноль\nтогда в скрипте проверку делать"
                }
                frame False {
                  n501 = call "RS_SMBV100A_PARS_SAT_TIME_AND_NUMBER.vi"("Parsing Satelite"=w1595) -> ("GPS 2D SAT"=w1597:dbl[][])  [unwired: 13 in, 5 out]
                  n502 = call "RS_SMBV100A_CONVERT_DATASAT_2D_to_N1D.vi"("2D DATA SAT"=w1597) -> ("GNSS_TimeSortedMaxToMin"=w1596:dbl[])  [unwired: 2 in, 5 out]
                }
              }
              n503 = call "RS_SMBV100A_Error_check.vi"("Driver Name"=w1592, "Error Code"=w1593, "Error In"=w1588, "DriverConnect in"=w1589) -> ("Error Out"=w1591:errorcluster)  [unwired: 6 in, 1 out]
            }
            frame "GNSS_N_TIME_SORTED_MAXTOMIN" {
              # "Массив времен в секундах GNSS спутников- по времени от наибольшего времени"
              n504 = Unbundle By Name(w1599) -> ("BASEBAND"=w1600:string)
              n505 = call "RS_SMBV100A_N_ASKCONFIGURATION.vi"("DriverConnect in"=w1606, "BASEBAND"=w1600, "mass"=w1603) -> ("wrong sat"=w1602:bool, "DriverConnect out"=w1605:T7, "Parsing Satelite"=w1598:T18, "Error Out"=w1604:errorcluster)  [unwired: 9 in]
              n506 = case shown="False" w1602 {
                tunnel: [dbl[] [0.0] ("GNSS_SatSkySortedMinToMax") w1612] -> w1601
                tunnel: w1598 -> [_ w1611]
                frame True {
                  # "Если Тру вернуть Ноль\nтогда в скрипте проверку делать"
                }
                frame False {
                  n507 = call "RS_SMBV100A_PARS_SAT_TIME_AND_NUMBER.vi"("Parsing Satelite"=w1611) -> ("GNSS 2D SAT"=w1613:dbl[][])  [unwired: 13 in, 5 out]
                  n508 = call "RS_SMBV100A_CONVERT_DATASAT_2D_to_N1D.vi"("2D DATA SAT"=w1613) -> ("GNSS_TimeSortedMaxToMin"=w1612:dbl[])  [unwired: 2 in, 5 out]
                }
              }
              n509 = call "RS_SMBV100A_Error_check.vi"("Driver Name"=w1608, "Error Code"=w1609, "Error In"=w1604, "DriverConnect in"=w1605) -> ("Error Out"=w1607:errorcluster)  [unwired: 6 in, 1 out]
            }
            frame "GLONASS_N_TIME_SORTED_MAXTOMIN" {
              # "Массив времен в секундах GLONASS спутников- по времени от наибольшего времени"
              n510 = Unbundle By Name(w1615) -> ("BASEBAND"=w1616:string)
              n511 = call "RS_SMBV100A_N_ASKCONFIGURATION.vi"("DriverConnect in"=w1622, "BASEBAND"=w1616, "mass"=w1619) -> ("wrong sat"=w1618:bool, "DriverConnect out"=w1621:T7, "Parsing Satelite"=w1614:T18, "Error Out"=w1620:errorcluster)  [unwired: 9 in]
              n512 = case shown="False" w1618 {
                tunnel: [dbl[] [0.0] ("GNSS_SatSkySortedMinToMax") w1629] -> w1617
                tunnel: w1614 -> [_ w1627]
                frame True {
                  # "Если Тру вернуть Ноль\nтогда в скрипте проверку делать"
                }
                frame False {
                  n513 = call "RS_SMBV100A_PARS_SAT_TIME_AND_NUMBER.vi"("Parsing Satelite"=w1627) -> ("GLONASS 2D SAT"=w1628:dbl[][])  [unwired: 13 in, 5 out]
                  n514 = call "RS_SMBV100A_CONVERT_DATASAT_2D_to_N1D.vi"("2D DATA SAT"=w1628) -> ("GNSS_TimeSortedMaxToMin"=w1629:dbl[])  [unwired: 2 in, 5 out]
                }
              }
              n515 = call "RS_SMBV100A_Error_check.vi"("Driver Name"=w1624, "Error Code"=w1625, "Error In"=w1620, "DriverConnect in"=w1621) -> ("Error Out"=w1623:errorcluster)  [unwired: 6 in, 1 out]
            }
            frame "GNSS_N_SKY_SORTED_MAXTOMIN" {
              # "Массив номеров GNSS спутников на небе - по времени от наибольшего времени"
              n516 = Unbundle By Name(w1631) -> ("BASEBAND"=w1632:string)
              n517 = call "RS_SMBV100A_N_ASKCONFIGURATION.vi"("DriverConnect in"=w1638, "BASEBAND"=w1632, "mass"=w1635) -> ("wrong sat"=w1633:bool, "DriverConnect out"=w1637:T7, "Parsing Satelite"=w1630:T18, "Error Out"=w1636:errorcluster)  [unwired: 9 in]
              n518 = case shown="False" w1633 {
                tunnel: [dbl[] [0.0] ("GNSS_SatSkySortedMinToMax") w1644] -> w1634
                tunnel: w1630 -> [_ w1643]
                frame True {
                  # "Если Тру вернуть Ноль\nтогда в скрипте проверку делать"
                }
                frame False {
                  n519 = call "RS_SMBV100A_PARS_SAT_TIME_AND_NUMBER.vi"("Parsing Satelite"=w1643) -> ("GNSS 2D SAT"=w1645:dbl[][])  [unwired: 13 in, 5 out]
                  n520 = call "RS_SMBV100A_CONVERT_DATASAT_2D_to_N1D.vi"("2D DATA SAT"=w1645) -> ("GNSS_SatSkySortedMaxToMin"=w1644:dbl[])  [unwired: 2 in, 5 out]
                }
              }
              n521 = call "RS_SMBV100A_Error_check.vi"("Driver Name"=w1640, "Error Code"=w1641, "Error In"=w1636, "DriverConnect in"=w1637) -> ("Error Out"=w1639:errorcluster)  [unwired: 6 in, 1 out]
            }
            frame "GPS_N_SKY_SORTED_MAXTOMIN" {
              # "Массив номеров GPS спутников на небе - по времени от наибольшего времени"
              n522 = Unbundle By Name(w1647) -> ("BASEBAND"=w1648:string)
              n523 = call "RS_SMBV100A_N_ASKCONFIGURATION.vi"("DriverConnect in"=w1654, "BASEBAND"=w1648, "mass"=w1651) -> ("wrong sat"=w1650:bool, "DriverConnect out"=w1653:T7, "Parsing Satelite"=w1646:T18, "Error Out"=w1652:errorcluster)  [unwired: 9 in]
              n524 = case shown="False" w1650 {
                tunnel: [dbl[] [0.0] ("GNSS_SatSkySortedMinToMax") w1661] -> w1649
                tunnel: w1646 -> [_ w1659]
                frame True {
                  # "Если Тру вернуть Ноль\nтогда в скрипте проверку делать"
                }
                frame False {
                  n525 = call "RS_SMBV100A_PARS_SAT_TIME_AND_NUMBER.vi"("Parsing Satelite"=w1659) -> ("GPS 2D SAT"=w1660:dbl[][])  [unwired: 13 in, 5 out]
                  n526 = call "RS_SMBV100A_CONVERT_DATASAT_2D_to_N1D.vi"("2D DATA SAT"=w1660) -> ("GNSS_SatSkySortedMaxToMin"=w1661:dbl[])  [unwired: 2 in, 5 out]
                }
              }
              n527 = call "RS_SMBV100A_Error_check.vi"("Driver Name"=w1656, "Error Code"=w1657, "Error In"=w1652, "DriverConnect in"=w1653) -> ("Error Out"=w1655:errorcluster)  [unwired: 6 in, 1 out]
            }
            frame "GLONASS_N_SKY_SORTED_MAXTOMIN" {
              # "Массив номеров GLONASS спутников на небе - по времени от наибольшего времени"
              n528 = Unbundle By Name(w1663) -> ("BASEBAND"=w1664:string)
              n529 = call "RS_SMBV100A_N_ASKCONFIGURATION.vi"("DriverConnect in"=w1670, "BASEBAND"=w1664, "mass"=w1667) -> ("wrong sat"=w1666:bool, "DriverConnect out"=w1669:T7, "Parsing Satelite"=w1662:T18, "Error Out"=w1668:errorcluster)  [unwired: 9 in]
              n530 = case shown="False" w1666 {
                tunnel: [dbl[] [0.0] ("GNSS_SatSkySortedMinToMax") w1676] -> w1665
                tunnel: w1662 -> [_ w1675]
                frame True {
                  # "Если Тру вернуть Ноль\nтогда в скрипте проверку делать"
                }
                frame False {
                  n531 = call "RS_SMBV100A_PARS_SAT_TIME_AND_NUMBER.vi"("Parsing Satelite"=w1675) -> ("GLONASS 2D SAT"=w1677:dbl[][])  [unwired: 13 in, 5 out]
                  n532 = call "RS_SMBV100A_CONVERT_DATASAT_2D_to_N1D.vi"("2D DATA SAT"=w1677) -> ("GNSS_SatSkySortedMaxToMin"=w1676:dbl[])  [unwired: 2 in, 5 out]
                }
              }
              n533 = call "RS_SMBV100A_Error_check.vi"("Driver Name"=w1672, "Error Code"=w1673, "Error In"=w1668, "DriverConnect in"=w1669) -> ("Error Out"=w1671:errorcluster)  [unwired: 6 in, 1 out]
            }
            frame "----- GLONASS BASEBAND -----" {
            }
            frame "EPHEMERISPARAMETERS_TOE" {
              # "спутник на небе"
              # "Возвращает время TOE от номера на небе спутника"
              n534 = Unbundle By Name(w1679) -> ("BASEBAND"=w1682:string)
              n535 = call "RS_SMBV100A_N_in_SKY_to_SAT_in_DEVICE.vi"("DriverConnect in"=w1701, "BASEBAND"=w1682, "String Value"=w1700) -> ("GNSS"=w1693:string, "DriverConnect out"=w1690:T7, "SATINSKY_for_DEVICE"=w1683:dbl, "Error Out"=w1692:errorcluster)  [unwired: 8 in, 1 out]
              n536 = Concatenate Strings(":" ("regular expression"), w1693) -> (w1695:string)
              n537 = Format Into String(format string="%.;%1.0f" ("format"), error in=w1692, w1683) -> (resulting string=w1697:string, error out=w1689:errorcluster)  [unwired: 1 in]
              n538 = Unbundle By Name(w1679) -> ("BASEBAND"=w1681:string)
              n539 = Concatenate Strings("SOUR:BB:" ("regular expression"), w1681, ":SVID" ("regular expression"), w1697, w1695, ":NMESsage:EPHemeris:TOE?" ("regular expression")) -> (w1691:string)
              n540 = call "RS_SMBV100A_FASTQUERY.vi"("input"=w1691, "Error In"=w1689, "DriverConnect in"=w1690) -> ("Error Out"=w1685:errorcluster, "DriverConnect out"=w1688:T7, "output"=w1687:string)  [unwired: 6 in]
              n541 = call "MLLF_FormatStringValue.vi"("error in"=w1685, "String Value"=w1687) -> ("error out"=w1684:T15, "number"=w1686:dbl)  [unwired: 7 in, 1 out]
              n542 = Build Array(w1686) -> (w1702:dbl[])
              n543 = call "RS_SMBV100A_Error_check.vi"("Driver Name"=w1704, "Error Code"=w1705, "Error In"=w1684, "DriverConnect in"=w1688) -> ("Error Out"=w1703:errorcluster)  [unwired: 6 in, 1 out]
            }
            frame "SIMULATIONDATE" {
              n544 = Unbundle By Name(w1706) -> ("BASEBAND"=w1709:string)
              n545 = Concatenate Strings("SOUR:BB:", w1709, ":NAV:SIM:DATE? " ("regular expression")) -> (w1707:string)
              n546 = call "RS_SMBV100A_FASTQUERY.vi"("input"=w1707, "DriverConnect in"=w1719) -> ("Error Out"=w1714:errorcluster, "DriverConnect out"=w1720:T7, "output"=w1716:string)  [unwired: 7 in]
              n547 = Scan From String(format string="%.;%<%d,%m,%Y>T", input string=w1716, error in=w1714) -> (error out=w1717:errorcluster, output 1=w1718:timestamp)  [unwired: 2 in, 2 out]
              n548 = Format Into String(format string="%,;%<%Y,%m,%d>T", error in=w1717, w1718) -> (resulting string=w1715:string, error out=w1713:errorcluster)  [unwired: 1 in]
              n549 = call "RS_SMBV100A_Error_check.vi"("Driver Name"=w1722, "Error Code"=w1723, "Error In"=w1713, "DriverConnect in"=w1720) -> ("Error Out"=w1721:errorcluster)  [unwired: 6 in, 1 out]
            }
            frame "CURRENTTIME" {
              w1728 = "SOUR:BB:"
              # "возвращает время в UTC"
              n550 = Unbundle By Name(w1741) -> ("BASEBAND"=w1727:string)
              n551 = Concatenate Strings(w1728, w1727, ":NAV:SIM:TIME? " ("regular expression")) -> (w1726:string)
              n552 = call "RS_SMBV100A_FASTQUERY.vi"("input"=w1726, "DriverConnect in"=w1731) -> ("DriverConnect out"=w1730:T7, "output"=w1725:string)  [unwired: 7 in, 1 out]
              n553 = Concatenate Strings(w1728, w1727, ":SPOT:NHOT? " ("regular expression")) -> (w1742:string)
              n554 = call "RS_SMBV100A_FASTQUERY.vi"("input"=w1742, "DriverConnect in"=w1730) -> ("Error Out"=w1732:errorcluster, "DriverConnect out"=w1744:T7, "output"=w1724:string)  [unwired: 7 in]
              n555 = call "MLLF_FormatStringValue.vi"("String Value"=w1724) -> ("number"=w1736:dbl)  [unwired: 8 in, 2 out]
              n556 = Scan From String(format string="%.;%<%H,%M,%S>T", input string=w1725, error in=w1732) -> (error out=w1739:errorcluster, output 1=w1737:timestamp)  [unwired: 2 in, 2 out]
              n557 = Add(x=w1737, y=w1736) -> (x+y=w1735:timestamp)
              n558 = Format Into String(format string="%.;%<%H,%M,%S%3u>T", error in=w1739, w1735) -> (resulting string=w1734:string, error out=w1733:errorcluster)  [unwired: 1 in]
              n559 = call "RS_SMBV100A_Error_check.vi"("Driver Name"=w1746, "Error Code"=w1747, "Error In"=w1733, "DriverConnect in"=w1744) -> ("Error Out"=w1745:errorcluster)  [unwired: 6 in, 1 out]
            }
            frame "SIMULATIONTIME" {
              n560 = Unbundle By Name(w1749) -> ("BASEBAND"=w1751:string)
              n561 = Concatenate Strings("SOUR:BB:", w1751, ":NAV:SIM:TIME? " ("regular expression")) -> (w1748:string)
              n562 = call "RS_SMBV100A_FASTQUERY.vi"("input"=w1748, "DriverConnect in"=w1753) -> ("Error Out"=w1756:errorcluster, "DriverConnect out"=w1755:T7, "output"=w1754:string)  [unwired: 7 in]
              n563 = call "RS_SMBV100A_Error_check.vi"("Driver Name"=w1758, "Error Code"=w1759, "Error In"=w1756, "DriverConnect in"=w1755) -> ("Error Out"=w1757:errorcluster)  [unwired: 6 in, 1 out]
            }
            frame "SATELLITECONFIGURATIONS_DURATION_UTC" {
              w1777 = " ," ("format")
              w1781 = "%1.0f" ("format")
              w1786 = 60.0 ("y")
              # "Определяет время в UTC спутника N(приборе)"
              n564 = Unbundle By Name(w1762) -> ("BASEBAND"=w1760:string)
              n565 = Concatenate Strings("SOUR:BB:", w1760, ":SAT" ("regular expression"), w1765, ":DUR? " ("regular expression")) -> (w1775:string)
              n566 = call "RS_SMBV100A_FASTQUERY.vi"("input"=w1775, "DriverConnect in"=w1766) -> ("Error Out"=w1764:errorcluster, "DriverConnect out"=w1767:T7, "output"=w1772:string)  [unwired: 7 in]
              n567 = call "MLLF_FormatStringValue.vi"("error in"=w1764, "String Value"=w1772) -> ("error out"=w1763:T15, "number"=w1787:dbl)  [unwired: 7 in, 1 out]
              n568 = Quotient & Remainder(x=w1787, y=w1786) -> (x-y*floor(x/y)=w1784:dbl, floor(x/y)=w1785:dbl)
              n569 = Quotient & Remainder(x=w1785, y=w1786) -> (x-y*floor(x/y)=w1783:dbl, floor(x/y)=w1782:dbl)
              n570 = Format Into String(format string=w1781, w1784) -> (resulting string=w1778:string)  [unwired: 2 in, 1 out]
              n571 = Format Into String(format string=w1781, w1783) -> (resulting string=w1779:string)  [unwired: 2 in, 1 out]
              n572 = Format Into String(format string=w1781, w1782) -> (resulting string=w1780:string)  [unwired: 2 in, 1 out]
              n573 = Concatenate Strings(w1780, w1777, w1779, w1777, w1778) -> (w1776:string)
              n574 = Scan From String(format string="%.;%<%H,%M,%S>T", input string=w1776, error in=w1763) -> (error out=w1789:errorcluster, output 1=w1791:timestamp)  [unwired: 2 in, 2 out]
              n575 = Format Into String(format string="%.;%<%H,%M,%S%3u>T", error in=w1789, w1791) -> (resulting string=w1788:string, error out=w1771:errorcluster)  [unwired: 1 in]
              n576 = call "RS_SMBV100A_Error_check.vi"("Driver Name"=w1768, "Error Code"=w1769, "Error In"=w1771, "DriverConnect in"=w1767) -> ("Error Out"=w1770:errorcluster)  [unwired: 6 in, 1 out]
            }
            frame "SATELLITECONFIGURATIONS_REAL_SAT_DURATION_UTC" {
              w1817 = " ," ("format")
              w1821 = "%1.0f" ("format")
              w1826 = 60.0 ("y")
              # "Определяет время в UTC спутника на небе"
              n577 = Unbundle By Name(w1793) -> ("BASEBAND"=w1794:string)
              n578 = call "RS_SMBV100A_N_in_SKY_to_SAT_in_DEVICE.vi"("DriverConnect in"=w1801, "BASEBAND"=w1794, "String Value"=w1797) -> ("DriverConnect out"=w1800:T7, "SAT"=w1803:dbl, "Error Out"=w1802:errorcluster)  [unwired: 8 in, 2 out]
              n579 = Unbundle By Name(w1793) -> ("BASEBAND"=w1795:string)
              n580 = Format Into String(format string="%.;%1.0f" ("format"), error in=w1802, w1803) -> (resulting string=w1798:string, error out=w1799:errorcluster)  [unwired: 1 in]
              n581 = Concatenate Strings("SOUR:BB:", w1795, ":SAT" ("regular expression"), w1798, ":DUR? " ("regular expression")) -> (w1815:string)
              n582 = call "RS_SMBV100A_FASTQUERY.vi"("input"=w1815, "Error In"=w1799, "DriverConnect in"=w1800) -> ("Error Out"=w1806:errorcluster, "DriverConnect out"=w1807:T7, "output"=w1812:string)  [unwired: 6 in]
              n583 = call "MLLF_FormatStringValue.vi"("error in"=w1806, "String Value"=w1812) -> ("error out"=w1805:T15, "number"=w1827:dbl)  [unwired: 7 in, 1 out]
              n584 = Quotient & Remainder(x=w1827, y=w1826) -> (x-y*floor(x/y)=w1824:dbl, floor(x/y)=w1825:dbl)
              n585 = Quotient & Remainder(x=w1825, y=w1826) -> (x-y*floor(x/y)=w1823:dbl, floor(x/y)=w1822:dbl)
              n586 = Format Into String(format string=w1821, w1824) -> (resulting string=w1818:string)  [unwired: 2 in, 1 out]
              n587 = Format Into String(format string=w1821, w1823) -> (resulting string=w1819:string)  [unwired: 2 in, 1 out]
              n588 = Format Into String(format string=w1821, w1822) -> (resulting string=w1820:string)  [unwired: 2 in, 1 out]
              n589 = Concatenate Strings(w1820, w1817, w1819, w1817, w1818) -> (w1816:string)
              n590 = Scan From String(format string="%.;%<%H,%M,%S>T", input string=w1816, error in=w1805) -> (error out=w1829:errorcluster, output 1=w1831:timestamp)  [unwired: 2 in, 2 out]
              n591 = Format Into String(format string="%.;%<%H,%M,%S%3u>T", error in=w1829, w1831) -> (resulting string=w1828:string, error out=w1811:errorcluster)  [unwired: 1 in]
              n592 = call "RS_SMBV100A_Error_check.vi"("Driver Name"=w1808, "Error Code"=w1809, "Error In"=w1811, "DriverConnect in"=w1807) -> ("Error Out"=w1810:errorcluster)  [unwired: 6 in, 1 out]
            }
            frame "SATELLITECONFIGURATIONS_DURATION_SEC" {
              # "Определяет время в UTC спутника N(в приборе)"
              n593 = Unbundle By Name(w1833) -> ("BASEBAND"=w1835:string)
              n594 = Concatenate Strings("SOUR:BB:", w1835, ":SAT" ("regular expression"), w1837, ":DUR? " ("regular expression")) -> (w1849:string)
              n595 = call "RS_SMBV100A_FASTQUERY.vi"("input"=w1849, "DriverConnect in"=w1838) -> ("Error Out"=w1839:errorcluster, "DriverConnect out"=w1843:T7, "output"=w1847:string)  [unwired: 7 in]
              n596 = call "MLLF_FormatStringValue.vi"("error in"=w1839, "String Value"=w1847) -> ("error out"=w1840:T15, "number"=w1842:dbl)  [unwired: 7 in, 1 out]
              n597 = call "RS_SMBV100A_Error_check.vi"("Driver Name"=w1844, "Error Code"=w1845, "Error In"=w1840, "DriverConnect in"=w1843) -> ("Error Out"=w1846:errorcluster)  [unwired: 6 in, 1 out]
              n598 = Build Array(w1842) -> (w1841:dbl[])
            }
            frame "SATELLITECONFIGURATIONS_REAL_SAT_DURATION_SEC" {
              # "Определяет время в UTC спутника на небе"
              n599 = Unbundle By Name(w1850) -> ("BASEBAND"=w1851:string)
              n600 = call "RS_SMBV100A_N_in_SKY_to_SAT_in_DEVICE.vi"("DriverConnect in"=w1860, "BASEBAND"=w1851, "String Value"=w1862) -> ("DriverConnect out"=w1861:T7, "SAT"=w1858:dbl, "Error Out"=w1857:errorcluster)  [unwired: 8 in, 2 out]
              n601 = Format Into String(format string="%.;%1.0f" ("format"), error in=w1857, w1858) -> (resulting string=w1855:string, error out=w1856:errorcluster)  [unwired: 1 in]
              n602 = Unbundle By Name(w1850) -> ("BASEBAND"=w1853:string)
              n603 = Concatenate Strings("SOUR:BB:", w1853, ":SAT" ("regular expression"), w1855, ":DUR? " ("regular expression")) -> (w1873:string)
              n604 = call "RS_SMBV100A_FASTQUERY.vi"("input"=w1873, "Error In"=w1856, "DriverConnect in"=w1861) -> ("Error Out"=w1863:errorcluster, "DriverConnect out"=w1867:T7, "output"=w1871:string)  [unwired: 6 in]
              n605 = call "MLLF_FormatStringValue.vi"("error in"=w1863, "String Value"=w1871) -> ("error out"=w1864:T15, "number"=w1866:dbl)  [unwired: 7 in, 1 out]
              n606 = call "RS_SMBV100A_Error_check.vi"("Driver Name"=w1868, "Error Code"=w1869, "Error In"=w1864, "DriverConnect in"=w1867) -> ("Error Out"=w1870:errorcluster)  [unwired: 6 in, 1 out]
              n607 = Build Array(w1866) -> (w1865:dbl[])
            }
            frame "SATELLITECONFIGURATIONS_DURATION" {
              w1889 = " ," ("format")
              w1893 = "%1.0f" ("format")
              w1898 = 60.0 ("y")
              # "Определяет время в UTC спутника N(приборе)"
              n608 = Unbundle By Name(w1874) -> ("BASEBAND"=w1875:string)
              n609 = Concatenate Strings("SOUR:BB:", w1875, ":SAT" ("regular expression"), w1877, ":DUR? " ("regular expression")) -> (w1887:string)
              n610 = call "RS_SMBV100A_FASTQUERY.vi"("input"=w1887, "DriverConnect in"=w1878) -> ("DriverConnect out"=w1879:T7, "output"=w1884:string)  [unwired: 7 in, 1 out]
              n611 = call "MLLF_FormatStringValue.vi"("String Value"=w1884) -> ("number"=w1899:dbl)  [unwired: 8 in, 2 out]
              n612 = Quotient & Remainder(x=w1899, y=w1898) -> (x-y*floor(x/y)=w1896:dbl, floor(x/y)=w1897:dbl)
              n613 = Quotient & Remainder(x=w1897, y=w1898) -> (x-y*floor(x/y)=w1895:dbl, floor(x/y)=w1894:dbl)
              n614 = Format Into String(format string=w1893, w1896) -> (resulting string=w1890:string)  [unwired: 2 in, 1 out]
              n615 = Format Into String(format string=w1893, w1895) -> (resulting string=w1891:string)  [unwired: 2 in, 1 out]
              n616 = Format Into String(format string=w1893, w1894) -> (resulting string=w1892:string)  [unwired: 2 in, 1 out]
              n617 = Concatenate Strings(w1892, w1889, w1891, w1889, w1890) -> (w1888:string)
              n618 = Scan From String(format string="%.;%<%H,%M,%S>T", input string=w1888) -> (error out=w1901:errorcluster, output 1=w1903:timestamp)  [unwired: 3 in, 2 out]
              n619 = Format Into String(format string="%.;%<%H,%M,%S%3u>T", error in=w1901, w1903) -> (resulting string=w1900:string, error out=w1883:errorcluster)  [unwired: 1 in]
              n620 = call "RS_SMBV100A_Error_check.vi"("Driver Name"=w1880, "Error Code"=w1881, "Error In"=w1883, "DriverConnect in"=w1879) -> ("Error Out"=w1882:errorcluster)  [unwired: 6 in, 1 out]
            }
            frame "GNNS_NUMBER_SAT_IN_SATELLITECONFIGURATIONS" {
              # "Отдает порядковый номер спутника в устройстве по номеру на Небе"
              n621 = Unbundle By Name(w1905) -> ("BASEBAND"=w1906:string)
              n622 = call "RS_SMBV100A_N_in_SKY_to_SAT_in_DEVICE.vi"("DriverConnect in"=w1911, "BASEBAND"=w1906, "String Value"=w1910) -> ("DriverConnect out"=w1908:T7, "SAT"=w1909:dbl, "Error Out"=w1907:errorcluster)  [unwired: 8 in, 2 out]
              n623 = Build Array(w1909) -> (w1912:dbl[])
              n624 = call "RS_SMBV100A_Error_check.vi"("Driver Name"=w1914, "Error Code"=w1915, "Error In"=w1907, "DriverConnect in"=w1908) -> ("Error Out"=w1913:errorcluster)  [unwired: 6 in, 1 out]
            }
            frame "----- GLONASS BASEBAND MASS -----" {
            }
            frame "GNNS_NUMBER_ACTIVE_SAT" {
              # "колличество активных спутников на Созвездии."
              n625 = Unbundle By Name(w1918) -> ("BASEBAND"=w1919:string)
              n626 = call "RS_SMBV100A_ASKCONFIGURATION.vi"("DriverConnect in"=w1923, "BASEBAND"=w1919) -> ("DriverConnect out"=w1922:T7, "Parsing Satelite"=w1917:T18, "Error Out"=w1921:errorcluster)  [unwired: 11 in]
              n627 = call "RS_SMBV100A_PARS_SAT_TIME_AND_NUMBER.vi"("Parsing Satelite"=w1917) -> ("OUT GNSS NUMBERACTIVESAT"=w1920:dbl)  [unwired: 13 in, 5 out]
              n628 = Build Array(w1920) -> (w1924:dbl[])
              n629 = call "RS_SMBV100A_Error_check.vi"("Driver Name"=w1926, "Error Code"=w1927, "Error In"=w1921, "DriverConnect in"=w1922) -> ("Error Out"=w1925:errorcluster)  [unwired: 6 in, 1 out]
            }
            frame "GPS_NUMBER_ACTIVE_SAT" {
              # "колличество активных спутников GPS на Созвездии."
              n630 = Unbundle By Name(w1930) -> ("BASEBAND"=w1929:string)
              n631 = call "RS_SMBV100A_ASKCONFIGURATION.vi"("DriverConnect in"=w1934, "BASEBAND"=w1929) -> ("DriverConnect out"=w1933:T7, "Parsing Satelite"=w1928:T18, "Error Out"=w1932:errorcluster)  [unwired: 11 in]
              n632 = call "RS_SMBV100A_PARS_SAT_TIME_AND_NUMBER.vi"("Parsing Satelite"=w1928) -> ("OUT GPS NUMBERACTIVESAT"=w1931:dbl)  [unwired: 13 in, 5 out]
              n633 = Build Array(w1931) -> (w1935:dbl[])
              n634 = call "RS_SMBV100A_Error_check.vi"("Driver Name"=w1937, "Error Code"=w1938, "Error In"=w1932, "DriverConnect in"=w1933) -> ("Error Out"=w1936:errorcluster)  [unwired: 6 in, 1 out]
            }
            frame "GLONASS_NUMBER_ACTIVE_SAT" {
              # "колличество активных спутников GLONASS на Созвездии."
              n635 = Unbundle By Name(w1941) -> ("BASEBAND"=w1940:string)
              n636 = call "RS_SMBV100A_ASKCONFIGURATION.vi"("DriverConnect in"=w1945, "BASEBAND"=w1940) -> ("DriverConnect out"=w1944:T7, "Parsing Satelite"=w1939:T18, "Error Out"=w1943:errorcluster)  [unwired: 11 in]
              n637 = call "RS_SMBV100A_PARS_SAT_TIME_AND_NUMBER.vi"("Parsing Satelite"=w1939) -> ("OUT GLONASS NUMBERACTIVESAT"=w1942:dbl)  [unwired: 13 in, 5 out]
              n638 = Build Array(w1942) -> (w1946:dbl[])
              n639 = call "RS_SMBV100A_Error_check.vi"("Driver Name"=w1948, "Error Code"=w1949, "Error In"=w1943, "DriverConnect in"=w1944) -> ("Error Out"=w1947:errorcluster)  [unwired: 6 in, 1 out]
            }
            frame "GNSS_SAT_SORTED_MINTOMAX" {
              # "Массив порядка спутников(не номеров собственных) по времени от наименьшего времени"
              n640 = Unbundle By Name(w1952) -> ("BASEBAND"=w1951:string)
              n641 = call "RS_SMBV100A_ASKCONFIGURATION.vi"("DriverConnect in"=w1957, "BASEBAND"=w1951) -> ("DriverConnect out"=w1956:T7, "Parsing Satelite"=w1950:T18, "Error Out"=w1955:errorcluster)  [unwired: 11 in]
              n642 = call "RS_SMBV100A_PARS_SAT_TIME_AND_NUMBER.vi"("Parsing Satelite"=w1950) -> ("GNSS 2D SAT"=w1953:dbl[][])  [unwired: 13 in, 5 out]
              n643 = call "RS_SMBV100A_CONVERT_DATASAT_2D_to_N1D.vi"("2D DATA SAT"=w1953) -> ("GNSS_SatSortedMinToMax"=w1954:dbl[])  [unwired: 2 in, 5 out]
              n644 = call "RS_SMBV100A_Error_check.vi"("Driver Name"=w1959, "Error Code"=w1960, "Error In"=w1955, "DriverConnect in"=w1956) -> ("Error Out"=w1958:errorcluster)  [unwired: 6 in, 1 out]
            }
            frame "GPS_SAT_SORTED_MINTOMAX" {
              # "Массив порядка GPS спутников(не номеров собственных) по времени от наименьшего времени"
              n645 = Unbundle By Name(w1962) -> ("BASEBAND"=w1963:string)
              n646 = call "RS_SMBV100A_ASKCONFIGURATION.vi"("DriverConnect in"=w1968, "BASEBAND"=w1963) -> ("DriverConnect out"=w1967:T7, "Parsing Satelite"=w1961:T18, "Error Out"=w1966:errorcluster)  [unwired: 11 in]
              n647 = call "RS_SMBV100A_PARS_SAT_TIME_AND_NUMBER.vi"("Parsing Satelite"=w1961) -> ("GPS 2D SAT"=w1964:dbl[][])  [unwired: 13 in, 5 out]
              n648 = call "RS_SMBV100A_CONVERT_DATASAT_2D_to_N1D.vi"("2D DATA SAT"=w1964) -> ("GNSS_SatSortedMinToMax"=w1965:dbl[])  [unwired: 2 in, 5 out]
              n649 = call "RS_SMBV100A_Error_check.vi"("Driver Name"=w1970, "Error Code"=w1971, "Error In"=w1966, "DriverConnect in"=w1967) -> ("Error Out"=w1969:errorcluster)  [unwired: 6 in, 1 out]
            }
            frame "GLONASS_SAT_SORTED_MINTOMAX" {
              # "Массив порядка GLONASS спутников(не номеров собственных) по времени от наименьшего времени"
              n650 = Unbundle By Name(w1973) -> ("BASEBAND"=w1974:string)
              n651 = call "RS_SMBV100A_ASKCONFIGURATION.vi"("DriverConnect in"=w1979, "BASEBAND"=w1974) -> ("DriverConnect out"=w1978:T7, "Parsing Satelite"=w1972:T18, "Error Out"=w1977:errorcluster)  [unwired: 11 in]
              n652 = call "RS_SMBV100A_PARS_SAT_TIME_AND_NUMBER.vi"("Parsing Satelite"=w1972) -> ("GLONASS 2D SAT"=w1975:dbl[][])  [unwired: 13 in, 5 out]
              n653 = call "RS_SMBV100A_CONVERT_DATASAT_2D_to_N1D.vi"("2D DATA SAT"=w1975) -> ("GNSS_SatSortedMinToMax"=w1976:dbl[])  [unwired: 2 in, 5 out]
              n654 = call "RS_SMBV100A_Error_check.vi"("Driver Name"=w1981, "Error Code"=w1982, "Error In"=w1977, "DriverConnect in"=w1978) -> ("Error Out"=w1980:errorcluster)  [unwired: 6 in, 1 out]
            }
            frame "GNSS_TIME_SORTED_MINTOMAX" {
              # "Массив времен в секундах GNSS спутников - от наименьшего времени"
              n655 = Unbundle By Name(w1984) -> ("BASEBAND"=w1985:string)
              n656 = call "RS_SMBV100A_ASKCONFIGURATION.vi"("DriverConnect in"=w1990, "BASEBAND"=w1985) -> ("DriverConnect out"=w1989:T7, "Parsing Satelite"=w1983:T18, "Error Out"=w1988:errorcluster)  [unwired: 11 in]
              n657 = call "RS_SMBV100A_PARS_SAT_TIME_AND_NUMBER.vi"("Parsing Satelite"=w1983) -> ("GNSS 2D SAT"=w1987:dbl[][])  [unwired: 13 in, 5 out]
              n658 = call "RS_SMBV100A_CONVERT_DATASAT_2D_to_N1D.vi"("2D DATA SAT"=w1987) -> ("GNSS_TimeSortedMinToMax"=w1986:dbl[])  [unwired: 2 in, 5 out]
              n659 = call "RS_SMBV100A_Error_check.vi"("Driver Name"=w1992, "Error Code"=w1993, "Error In"=w1988, "DriverConnect in"=w1989) -> ("Error Out"=w1991:errorcluster)  [unwired: 6 in, 1 out]
            }
            frame "GPS_TIME_SORTED_MINTOMAX" {
              # "Массив времен в секундах GPS спутников - от наименьшего времени"
              n660 = Unbundle By Name(w1995) -> ("BASEBAND"=w1996:string)
              n661 = call "RS_SMBV100A_ASKCONFIGURATION.vi"("DriverConnect in"=w2001, "BASEBAND"=w1996) -> ("DriverConnect out"=w2000:T7, "Parsing Satelite"=w1994:T18, "Error Out"=w1999:errorcluster)  [unwired: 11 in]
              n662 = call "RS_SMBV100A_PARS_SAT_TIME_AND_NUMBER.vi"("Parsing Satelite"=w1994) -> ("GPS 2D SAT"=w1997:dbl[][])  [unwired: 13 in, 5 out]
              n663 = call "RS_SMBV100A_CONVERT_DATASAT_2D_to_N1D.vi"("2D DATA SAT"=w1997) -> ("GNSS_TimeSortedMinToMax"=w1998:dbl[])  [unwired: 2 in, 5 out]
              n664 = call "RS_SMBV100A_Error_check.vi"("Driver Name"=w2003, "Error Code"=w2004, "Error In"=w1999, "DriverConnect in"=w2000) -> ("Error Out"=w2002:errorcluster)  [unwired: 6 in, 1 out]
            }
            frame "GLONASS_TIME_SORTED_MINTOMAX" {
              # "Массив времен в секундах GLONASS спутников - от наименьшего времени"
              n665 = Unbundle By Name(w2006) -> ("BASEBAND"=w2007:string)
              n666 = call "RS_SMBV100A_ASKCONFIGURATION.vi"("DriverConnect in"=w2012, "BASEBAND"=w2007) -> ("DriverConnect out"=w2011:T7, "Parsing Satelite"=w2005:T18, "Error Out"=w2010:errorcluster)  [unwired: 11 in]
              n667 = call "RS_SMBV100A_PARS_SAT_TIME_AND_NUMBER.vi"("Parsing Satelite"=w2005) -> ("GLONASS 2D SAT"=w2008:dbl[][])  [unwired: 13 in, 5 out]
              n668 = call "RS_SMBV100A_CONVERT_DATASAT_2D_to_N1D.vi"("2D DATA SAT"=w2008) -> ("GNSS_TimeSortedMinToMax"=w2009:dbl[])  [unwired: 2 in, 5 out]
              n669 = call "RS_SMBV100A_Error_check.vi"("Driver Name"=w2014, "Error Code"=w2015, "Error In"=w2010, "DriverConnect in"=w2011) -> ("Error Out"=w2013:errorcluster)  [unwired: 6 in, 1 out]
            }
            frame "GNSS_SKY_SORTED_MINTOMAX" {
              # "Массив номеров GNSS спутников на небе - от наименьшего времени"
              n670 = Unbundle By Name(w2017) -> ("BASEBAND"=w2018:string)
              n671 = call "RS_SMBV100A_ASKCONFIGURATION.vi"("DriverConnect in"=w2023, "BASEBAND"=w2018) -> ("DriverConnect out"=w2022:T7, "Parsing Satelite"=w2016:T18, "Error Out"=w2021:errorcluster)  [unwired: 11 in]
              n672 = call "RS_SMBV100A_PARS_SAT_TIME_AND_NUMBER.vi"("Parsing Satelite"=w2016) -> ("GNSS 2D SAT"=w2019:dbl[][])  [unwired: 13 in, 5 out]
              n673 = call "RS_SMBV100A_CONVERT_DATASAT_2D_to_N1D.vi"("2D DATA SAT"=w2019) -> ("GNSS_SatSkySortedMinToMax"=w2020:dbl[])  [unwired: 2 in, 5 out]
              n674 = call "RS_SMBV100A_Error_check.vi"("Driver Name"=w2025, "Error Code"=w2026, "Error In"=w2021, "DriverConnect in"=w2022) -> ("Error Out"=w2024:errorcluster)  [unwired: 6 in, 1 out]
            }
            frame "GPS_SKY_SORTED_MINTOMAX" {
              # "Массив номеров GPS спутников на небе - от наименьшего времени"
              n675 = Unbundle By Name(w2028) -> ("BASEBAND"=w2029:string)
              n676 = call "RS_SMBV100A_ASKCONFIGURATION.vi"("DriverConnect in"=w2034, "BASEBAND"=w2029) -> ("DriverConnect out"=w2033:T7, "Parsing Satelite"=w2027:T18, "Error Out"=w2032:errorcluster)  [unwired: 11 in]
              n677 = call "RS_SMBV100A_PARS_SAT_TIME_AND_NUMBER.vi"("Parsing Satelite"=w2027) -> ("GPS 2D SAT"=w2030:dbl[][])  [unwired: 13 in, 5 out]
              n678 = call "RS_SMBV100A_CONVERT_DATASAT_2D_to_N1D.vi"("2D DATA SAT"=w2030) -> ("GNSS_SatSkySortedMinToMax"=w2031:dbl[])  [unwired: 2 in, 5 out]
              n679 = call "RS_SMBV100A_Error_check.vi"("Driver Name"=w2036, "Error Code"=w2037, "Error In"=w2032, "DriverConnect in"=w2033) -> ("Error Out"=w2035:errorcluster)  [unwired: 6 in, 1 out]
            }
            frame "GLONASS_SKY_SORTED_MINTOMAX" {
              # "Массив номеров GLONASS спутников на небе - от наименьшего времени"
              n680 = Unbundle By Name(w2039) -> ("BASEBAND"=w2040:string)
              n681 = call "RS_SMBV100A_ASKCONFIGURATION.vi"("DriverConnect in"=w2045, "BASEBAND"=w2040) -> ("DriverConnect out"=w2044:T7, "Parsing Satelite"=w2038:T18, "Error Out"=w2043:errorcluster)  [unwired: 11 in]
              n682 = call "RS_SMBV100A_PARS_SAT_TIME_AND_NUMBER.vi"("Parsing Satelite"=w2038) -> ("GLONASS 2D SAT"=w2041:dbl[][])  [unwired: 13 in, 5 out]
              n683 = call "RS_SMBV100A_CONVERT_DATASAT_2D_to_N1D.vi"("2D DATA SAT"=w2041) -> ("GNSS_SatSkySortedMinToMax"=w2042:dbl[])  [unwired: 2 in, 5 out]
              n684 = call "RS_SMBV100A_Error_check.vi"("Driver Name"=w2047, "Error Code"=w2048, "Error In"=w2043, "DriverConnect in"=w2044) -> ("Error Out"=w2046:errorcluster)  [unwired: 6 in, 1 out]
            }
            frame "GNSS_SAT_SORTED_MAXTOMIN" {
              # "Массив порядка спутников(не номеров собственных) по времени от наибольшего времени"
              n685 = Unbundle By Name(w2050) -> ("BASEBAND"=w2051:string)
              n686 = call "RS_SMBV100A_ASKCONFIGURATION.vi"("DriverConnect in"=w2056, "BASEBAND"=w2051) -> ("DriverConnect out"=w2055:T7, "Parsing Satelite"=w2049:T18, "Error Out"=w2054:errorcluster)  [unwired: 11 in]
              n687 = call "RS_SMBV100A_PARS_SAT_TIME_AND_NUMBER.vi"("Parsing Satelite"=w2049) -> ("GNSS 2D SAT"=w2053:dbl[][])  [unwired: 13 in, 5 out]
              n688 = call "RS_SMBV100A_CONVERT_DATASAT_2D_to_N1D.vi"("2D DATA SAT"=w2053) -> ("GNSS_SatSortedMaxToMin"=w2052:dbl[])  [unwired: 2 in, 5 out]
              n689 = call "RS_SMBV100A_Error_check.vi"("Driver Name"=w2058, "Error Code"=w2059, "Error In"=w2054, "DriverConnect in"=w2055) -> ("Error Out"=w2057:errorcluster)  [unwired: 6 in, 1 out]
            }
            frame "GPS_SAT_SORTED_MAXTOMIN" {
              # "Массив порядка GPS спутников(не номеров собственных) по времени от наибольшего времени"
              n690 = Unbundle By Name(w2061) -> ("BASEBAND"=w2062:string)
              n691 = call "RS_SMBV100A_ASKCONFIGURATION.vi"("DriverConnect in"=w2067, "BASEBAND"=w2062) -> ("DriverConnect out"=w2066:T7, "Parsing Satelite"=w2060:T18, "Error Out"=w2065:errorcluster)  [unwired: 11 in]
              n692 = call "RS_SMBV100A_PARS_SAT_TIME_AND_NUMBER.vi"("Parsing Satelite"=w2060) -> ("GPS 2D SAT"=w2063:dbl[][])  [unwired: 13 in, 5 out]
              n693 = call "RS_SMBV100A_CONVERT_DATASAT_2D_to_N1D.vi"("2D DATA SAT"=w2063) -> ("GNSS_SatSortedMaxToMin"=w2064:dbl[])  [unwired: 2 in, 5 out]
              n694 = call "RS_SMBV100A_Error_check.vi"("Driver Name"=w2069, "Error Code"=w2070, "Error In"=w2065, "DriverConnect in"=w2066) -> ("Error Out"=w2068:errorcluster)  [unwired: 6 in, 1 out]
            }
            frame "GLONASS_SAT_SORTED_MAXTOMIN" {
              # "Массив порядка GLONASS спутников(не номеров собственных) по времени от наибольшего времени"
              n695 = Unbundle By Name(w2072) -> ("BASEBAND"=w2073:string)
              n696 = call "RS_SMBV100A_ASKCONFIGURATION.vi"("DriverConnect in"=w2078, "BASEBAND"=w2073) -> ("DriverConnect out"=w2077:T7, "Parsing Satelite"=w2071:T18, "Error Out"=w2076:errorcluster)  [unwired: 11 in]
              n697 = call "RS_SMBV100A_PARS_SAT_TIME_AND_NUMBER.vi"("Parsing Satelite"=w2071) -> ("GLONASS 2D SAT"=w2074:dbl[][])  [unwired: 13 in, 5 out]
              n698 = call "RS_SMBV100A_CONVERT_DATASAT_2D_to_N1D.vi"("2D DATA SAT"=w2074) -> ("GNSS_SatSortedMaxToMin"=w2075:dbl[])  [unwired: 2 in, 5 out]
              n699 = call "RS_SMBV100A_Error_check.vi"("Driver Name"=w2080, "Error Code"=w2081, "Error In"=w2076, "DriverConnect in"=w2077) -> ("Error Out"=w2079:errorcluster)  [unwired: 6 in, 1 out]
            }
            frame "GNSS_TIME_SORTED_MAXTOMIN" {
              # "Массив времен в секундах GNSS спутников- по времени от наибольшего времени"
              n700 = Unbundle By Name(w2083) -> ("BASEBAND"=w2084:string)
              n701 = call "RS_SMBV100A_ASKCONFIGURATION.vi"("DriverConnect in"=w2089, "BASEBAND"=w2084) -> ("DriverConnect out"=w2088:T7, "Parsing Satelite"=w2082:T18, "Error Out"=w2087:errorcluster)  [unwired: 11 in]
              n702 = call "RS_SMBV100A_PARS_SAT_TIME_AND_NUMBER.vi"("Parsing Satelite"=w2082) -> ("GNSS 2D SAT"=w2085:dbl[][])  [unwired: 13 in, 5 out]
              n703 = call "RS_SMBV100A_CONVERT_DATASAT_2D_to_N1D.vi"("2D DATA SAT"=w2085) -> ("GNSS_TimeSortedMaxToMin"=w2086:dbl[])  [unwired: 2 in, 5 out]
              n704 = call "RS_SMBV100A_Error_check.vi"("Driver Name"=w2091, "Error Code"=w2092, "Error In"=w2087, "DriverConnect in"=w2088) -> ("Error Out"=w2090:errorcluster)  [unwired: 6 in, 1 out]
            }
            frame "GPS_TIME_SORTED_MAXTOMIN" {
              # "Массив времен в секундах GPS спутников- по времени от наибольшего времени"
              n705 = Unbundle By Name(w2094) -> ("BASEBAND"=w2095:string)
              n706 = call "RS_SMBV100A_ASKCONFIGURATION.vi"("DriverConnect in"=w2100, "BASEBAND"=w2095) -> ("DriverConnect out"=w2099:T7, "Parsing Satelite"=w2093:T18, "Error Out"=w2098:errorcluster)  [unwired: 11 in]
              n707 = call "RS_SMBV100A_PARS_SAT_TIME_AND_NUMBER.vi"("Parsing Satelite"=w2093) -> ("GPS 2D SAT"=w2096:dbl[][])  [unwired: 13 in, 5 out]
              n708 = call "RS_SMBV100A_CONVERT_DATASAT_2D_to_N1D.vi"("2D DATA SAT"=w2096) -> ("GNSS_TimeSortedMaxToMin"=w2097:dbl[])  [unwired: 2 in, 5 out]
              n709 = call "RS_SMBV100A_Error_check.vi"("Driver Name"=w2102, "Error Code"=w2103, "Error In"=w2098, "DriverConnect in"=w2099) -> ("Error Out"=w2101:errorcluster)  [unwired: 6 in, 1 out]
            }
            frame "GLONASS_TIME_SORTED_MAXTOMIN" {
              # "Массив времен в секундах GLONASS спутников- по времени от наибольшего времени"
              n710 = Unbundle By Name(w2105) -> ("BASEBAND"=w2106:string)
              n711 = call "RS_SMBV100A_ASKCONFIGURATION.vi"("DriverConnect in"=w2111, "BASEBAND"=w2106) -> ("DriverConnect out"=w2110:T7, "Parsing Satelite"=w2104:T18, "Error Out"=w2109:errorcluster)  [unwired: 11 in]
              n712 = call "RS_SMBV100A_PARS_SAT_TIME_AND_NUMBER.vi"("Parsing Satelite"=w2104) -> ("GLONASS 2D SAT"=w2107:dbl[][])  [unwired: 13 in, 5 out]
              n713 = call "RS_SMBV100A_CONVERT_DATASAT_2D_to_N1D.vi"("2D DATA SAT"=w2107) -> ("GNSS_TimeSortedMaxToMin"=w2108:dbl[])  [unwired: 2 in, 5 out]
              n714 = call "RS_SMBV100A_Error_check.vi"("Driver Name"=w2113, "Error Code"=w2114, "Error In"=w2109, "DriverConnect in"=w2110) -> ("Error Out"=w2112:errorcluster)  [unwired: 6 in, 1 out]
            }
            frame "GNSS_SKY_SORTED_MAXTOMIN" {
              # "Массив номеров GNSS спутников на небе - по времени от наибольшего времени"
              n715 = Unbundle By Name(w2116) -> ("BASEBAND"=w2117:string)
              n716 = call "RS_SMBV100A_ASKCONFIGURATION.vi"("DriverConnect in"=w2124, "BASEBAND"=w2117) -> ("DriverConnect out"=w2121:T7, "Parsing Satelite"=w2115:T18, "Error Out"=w2120:errorcluster)  [unwired: 11 in]
              n717 = call "RS_SMBV100A_PARS_SAT_TIME_AND_NUMBER.vi"("Parsing Satelite"=w2115) -> ("GNSS 2D SAT"=w2119:dbl[][])  [unwired: 13 in, 5 out]
              n718 = call "RS_SMBV100A_CONVERT_DATASAT_2D_to_N1D.vi"("2D DATA SAT"=w2119) -> ("GNSS_SatSkySortedMaxToMin"=w2123:dbl[])  [unwired: 2 in, 5 out]
              n719 = call "RS_SMBV100A_Error_check.vi"("Driver Name"=w2125, "Error Code"=w2126, "Error In"=w2120, "DriverConnect in"=w2121) -> ("Error Out"=w2118:errorcluster)  [unwired: 6 in, 1 out]
              n720 = call "MLLF_ParsingIntArrayToString (SubVI).vi"("Value"=w2123) -> ("String"=w2122:string)  [unwired: 10 in]
            }
            frame "GPS_SKY_SORTED_MAXTOMIN" {
              # "Массив номеров GPS спутников на небе - по времени от наибольшего времени"
              n721 = Unbundle By Name(w2128) -> ("BASEBAND"=w2129:string)
              n722 = call "RS_SMBV100A_ASKCONFIGURATION.vi"("DriverConnect in"=w2134, "BASEBAND"=w2129) -> ("DriverConnect out"=w2133:T7, "Parsing Satelite"=w2127:T18, "Error Out"=w2132:errorcluster)  [unwired: 11 in]
              n723 = call "RS_SMBV100A_PARS_SAT_TIME_AND_NUMBER.vi"("Parsing Satelite"=w2127) -> ("GPS 2D SAT"=w2130:dbl[][])  [unwired: 13 in, 5 out]
              n724 = call "RS_SMBV100A_CONVERT_DATASAT_2D_to_N1D.vi"("2D DATA SAT"=w2130) -> ("GNSS_SatSkySortedMaxToMin"=w2131:dbl[])  [unwired: 2 in, 5 out]
              n725 = call "RS_SMBV100A_Error_check.vi"("Driver Name"=w2136, "Error Code"=w2137, "Error In"=w2132, "DriverConnect in"=w2133) -> ("Error Out"=w2135:errorcluster)  [unwired: 6 in, 1 out]
            }
            frame "GLONASS_SKY_SORTED_MAXTOMIN" {
              # "Массив номеров GLONASS спутников на небе - по времени от наибольшего времени"
              n726 = Unbundle By Name(w2139) -> ("BASEBAND"=w2140:string)
              n727 = call "RS_SMBV100A_ASKCONFIGURATION.vi"("DriverConnect in"=w2145, "BASEBAND"=w2140) -> ("DriverConnect out"=w2144:T7, "Parsing Satelite"=w2138:T18, "Error Out"=w2143:errorcluster)  [unwired: 11 in]
              n728 = call "RS_SMBV100A_PARS_SAT_TIME_AND_NUMBER.vi"("Parsing Satelite"=w2138) -> ("GLONASS 2D SAT"=w2141:dbl[][])  [unwired: 13 in, 5 out]
              n729 = call "RS_SMBV100A_CONVERT_DATASAT_2D_to_N1D.vi"("2D DATA SAT"=w2141) -> ("GNSS_SatSkySortedMaxToMin"=w2142:dbl[])  [unwired: 2 in, 5 out]
              n730 = call "RS_SMBV100A_Error_check.vi"("Driver Name"=w2147, "Error Code"=w2148, "Error In"=w2143, "DriverConnect in"=w2144) -> ("Error Out"=w2146:errorcluster)  [unwired: 6 in, 1 out]
            }
          }
          n731 = call "MLLF_FormatOutputValueWithUnits.vi"("Lower limit"=-1e+32, "Upper limit"=1e+32, "error in"=w1268, "ValuesIn"=w1270) -> ("error out"=w1263:T15, "Result string"=w1271:T16)  [unwired: 6 in]
          n732 = Concatenate Strings(w1271, w1265) -> (w1264:string)
        }
        frame "close" {
          # "Завершение сессии"
          n733 = Unbundle By Name(w2150) -> ("Data.Connect.OpenedSession"=w2152:T9)
          n734 = VISA Close(VISA resource name=w2152) -> (error out=w2151:errorcluster)  [unwired: 1 in]
        }
      }
    }
    frame Error {
    }
  }
  n735 = local write "Settings"(w10) -> ()
  n736 = flat-sequence {
    tunnel: [w2163] -> w3
    tunnel: [w2162] -> w2
    tunnel: w6 -> [w2161]
    tunnel: w4 -> [w2160]
    tunnel: w5 -> [w2157]
    tunnel: [w2155] -> _
    tunnel: [w2155] -> w1
    frame #0 {
      # "driver out"
      n737 = Unbundle By Name(w2157) -> ("Data"=w2156:cluster{"Connect":T7})
      n738 = To Variant(anything=w2156) -> (Variant=w2158:variant)
      n739 = Bundle By Name(cluster=w2157, "Saved Data"=w2158) -> (w2155:T12)
      n740 = call "MLLF_SaveLastSettingUtility.vi"("error in"=w2160, "Saved Data"=w2158) -> ("error out"=w2159:T15)  [unwired: 8 in, 1 out]
      n741 = call "MCF_Output.vi"("Error In"=w2159, "Input"=w2161) -> ("Error Out"=w2162:errorcluster, "Output"=w2163:string)  [unwired: 8 in]
    }
  }
  n742 = local write "Settings"(w1) -> ()
  "error out" <- w2
  "Response" <- w3
